vi "Main.vi"() -> ()   [LabVIEW 2021]
doc: "使用该模板构建简单状态机设计模式。各状态执行代码并决定转移状态。"
uses:
  <vilib>/Utility/miscctls.llb/LVRowAndColumnTypeDef.ctl
  controls/State.ctl
  controls/ProcessState.ctl
  <vilib>/Platform/TimedLoop/XDataNode/timing_clust.ctl
  <vilib>/Platform/TimedLoop/XDataNode/nitl_modes.ctl
  <vilib>/Platform/TimedLoop/XDataNode/wakeup.ctl
  controls/DataInitDef.ctl
  <vilib>/event_ctls.llb/eventvkey.ctl
  <vilib>/Utility/NIReport.llb/Report Type.ctl
  controls/Config Section init.ctl
  <vilib>/Platform/TimedLoop/XDataNode/XDataNode.xnode
  <vilib>/Utility/NIReport.llb/NI_report.lvclass
  <vilib>/Utility/NIReport.llb/NI_ReportGenerationCore.lvlib
  <vilib>/Utility/NIReport.llb/Excel/NI_Excel.lvclass
  <vilib>/Platform/TimedLoop/XDataNode/XDNodeRunTimeDep.lvlib
panel:
  in  "项目名":string caption="PCAN 1.6(2021)"
  in  "i2":u32
  in  "i1":i32
  out "运行ID":u32
  in  "曲线16设置":string
  in  "曲线15设置":string
  in  "曲线14设置":string
  in  "曲线13设置":string
  in  "曲线12设置":string
  in  "曲线11设置":string
  in  "曲线10设置":string
  in  "曲线9设置":string
  out "布控5设置":string
  out "CAN通道":u8
  in  "曲线8设置":string
  in  "曲线7设置":string
  in  "曲线6设置":string
  in  "曲线5设置":string
  in  "曲线4设置":string
  in  "曲线3设置":string
  in  "曲线2设置":string
  in  "曲线1设置":string
  out "故障内容":string[](array[string])
  out "故障信息":string[](array[string])
  out "故障地址":string[](array[string])
  out "故障字典":string[][](table)
  out "设控设置 8":string
  out "设控设置 7":string
  out "设控设置 6":string
  out "设控设置 5":string
  out "设控设置 4":string
  out "设控设置 3":string
  out "设控设置 2":string
  out "设控设置 1":string
  out "延时更新布尔状态":i16
  out "要发送的数据":cluster{"地址":u16, "数据":i32, "行数":i32, "ID":i32}
  out "CANBURF":u32[][](array[numeric])
  out "当前显示表格总行数":i32
  out "布控4设置":string
  out "布控2设置":string
  out "布控3设置":string
  out "控件配置文件":string[][](table)
  out "显控12设置":string
  out "显控11设置":string
  out "显控10设置":string
  out "显控9设置":string
  out "显控8设置":string
  out "显控7设置":string
  out "显控6设置":string
  out "显控5设置":string
  out "显控4设置":string
  out "显控3设置":string
  out "显控2设置":string
  out "显控1设置":string
  out "错误计数器":u32
  out "循环指针":u16
  out "布控1设置":string
  out "配置文件":string[][](array[string])
  out "选择区域起始":T1
  in  "选项卡控件":enum32{"调试界面", "波形记录"}(tab)
  in  "确定按钮":bool
  in  "数据模式":bool
  in  "布尔 5":bool
  in  "布尔 4":bool
  in  "布尔 3":bool
  in  "布尔 2":bool
  in  "布尔 1":bool
  in  "ID":u32=43690 format="%x"
  out "通信状态":string
  in  "刷新间隔":string="5" caption="ms"
  out "轮询一次周期":string caption="s"
  in  "重新连接":bool
  in  "波特率":u16(ring)=28 items=["BAUD_5K"=32639, "BAUD_10K"=26415, "BAUD_20K"=21295, "BAUD_50K"=18223, "BAUD_100K"=17199, "BAUD_125K"=796, "BAUD_250K"=284, "BAUD_500K"=28, "BAUD_1M"=20]
  in  "退出":bool=TRUE
  in  "设控8":string
  in  "设控7":string
  in  "设控6":string
  in  "设控5":string
  in  "设控4":string
  in  "设控3":string
  in  "设控2":string
  in  "设控1":string
  out "状态显示":string
  out "显控12":string
  out "显控11":string
  out "显控10":string
  out "显控9":string
  out "显控5":string
  out "显控1":string
  out "显控8":string
  out "显控7":string
  out "显控6":string
  out "显控4":string
  out "显控3":string
  out "显控2":string
  in  "设置":string caption="WARN_H字"
  in  "选择参数表":path caption="导入参数"
  in  "表格":string[][](table)
  in  "清除历史记录":bool
  out "波形图表":dynamicdata(graph)
  in  "记录波形更新":bool=TRUE
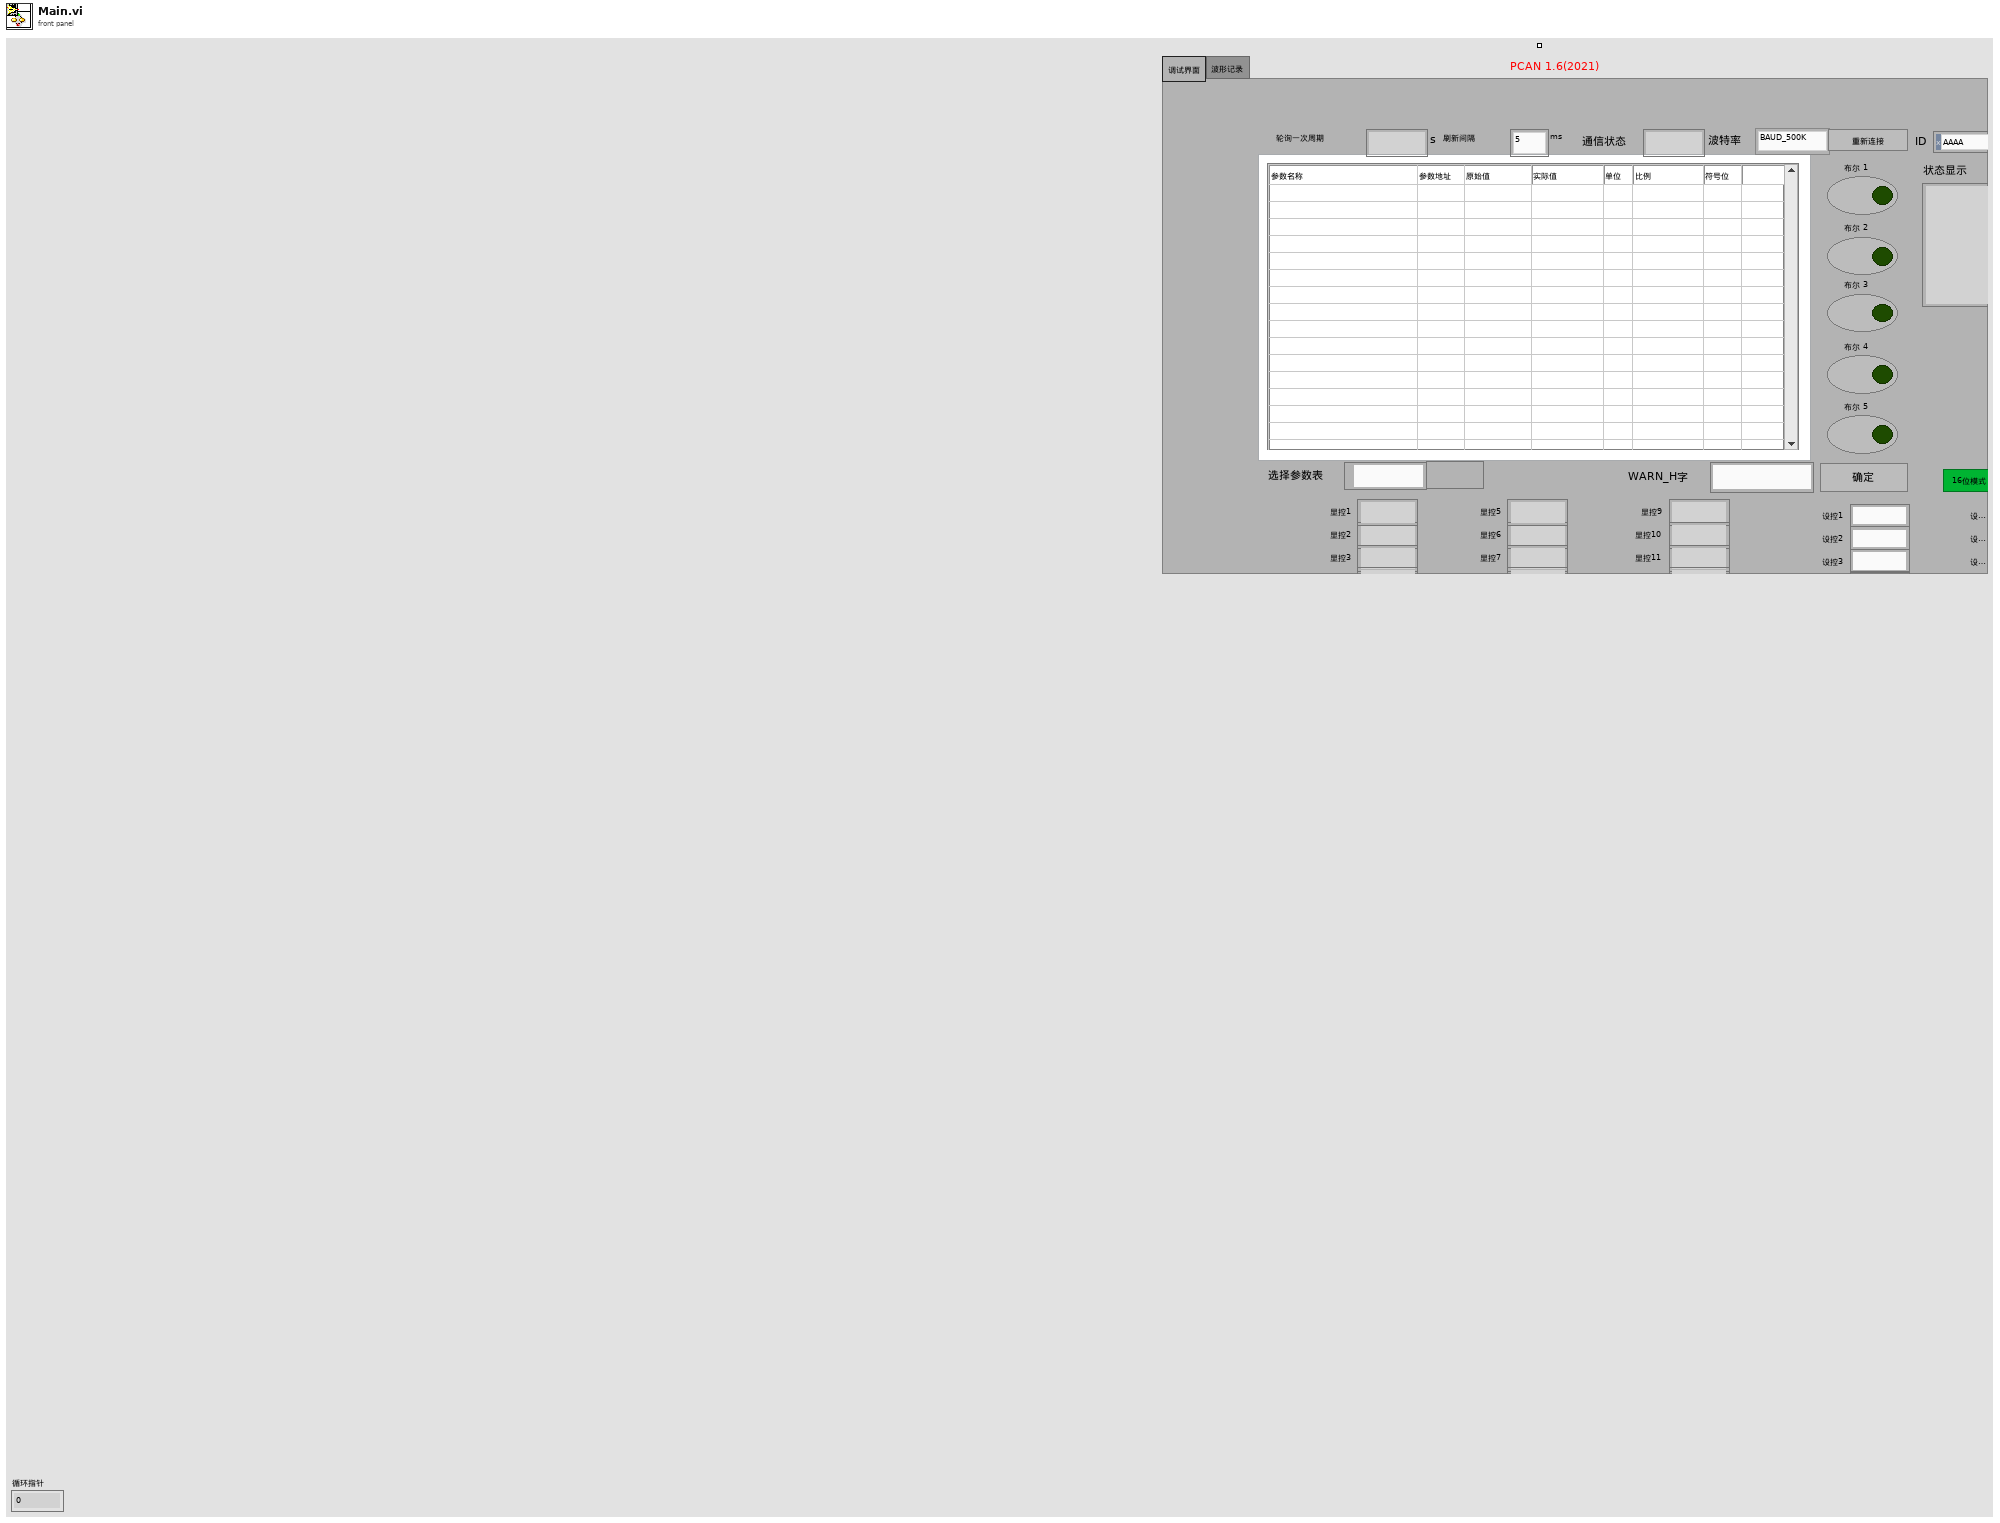
[diagram p1: front panel]
types:
  T1 = typedef "LVRowAndColumnTypeDef.ctl" = cluster{"Row":i32, "Column":i32}
  T2 = typedef "ProcessState.ctl" = enum16{"Start", "Process", "Exit"}
  T3 = typedef "State.ctl" = enum16{"Initialize", "ResetCAN", "SetCAN", "Process", "Exit", "ERROR", "STOP"}
  T4 = typedef "XDNodeRunTimeDep.lvlib/timing_clust.ctl" = cluster{"Expected End [f-1]":u64, "Actual End [f-1]":u64, "Finished Late? [f-1]":bool, "Expected End [i-1]":u64, "Actual End [i-1]":u64, "Finished Late? [i-1]":bool, "Expected Start [i]":u64, "Actual Start [i]":u64, "Expected Start [f]":u64, "Actual Start [f]":u64, "Source Name":string, "Structure Name":string, "Period":i64, "Deadline":i64, "Offset":i64, "Start":i64, "Priority":i32, "Timeout":i32, "Mode":T5, "Wakeup Reason":T6, "Error":errorcluster, "Source Type":string, "Secondary Source Type":string, "Global End Time":u64, "Global Start Time":u64, "Frame Duration":u64, "Iteration Duration":u64, "Assigned CPU":i32, "I/O Scan Engine Mode":u32}
  T5 = typedef "XDNodeRunTimeDep.lvlib/nitl_modes.ctl" = enum32{"No Change", "Process missed periods, maintain original phase", "Discard missed periods, maintain original phase", "Process missed periods, ignore original phase", "Discard missed periods, ignore original phase"}
  T6 = typedef "XDNodeRunTimeDep.lvlib/wakeup.ctl" = enum32{"Normal", "Aborted", "Asynchronous wakeup", "Timing source error", "Timed loop error", "Timeout"}
  T7 = typedef "eventvkey.ctl" = enum16{"ASCII", "Enter", "Return", "Shift", "Ctrl", "Alt", "Cmd", "Opt", "Caps", "NumLock", "Clear", "Break", "Up", "Down", "Left", "Right", "Insert", "Delete", "Home", "End", "PageUp", "PageDown", "Escape", "Help", "Pause", "ScrollLock", "F1", "F2", "F3", "F4", "F5", "F6", "F7", "F8", "F9", "F10", "F11", "F12", "F13", "F14", "F15", "F16", "F17", "F18", "F19", "F20", "F21", "F22", "F23", "F24", "Play", "VolumeUp", "VolumeDown", "Mute", "Two Byte Char"}
  T8 = typedef "NI_ReportGenerationCore.lvlib/Report Type.ctl" = enum16{"HTML", "Word", "Excel"}
  T9 = typedef "DataInitDef.ctl" = u16
  T10 = cluster{u16, i64, "Row":i32, "offset past number":i32}
  T11 = cluster{"position (excel)":cluster{"row":i32, "column":i32}, "name (excel)":string, "bookmark (word)":string}
  T12 = typedef "Config Section init.ctl" = u16
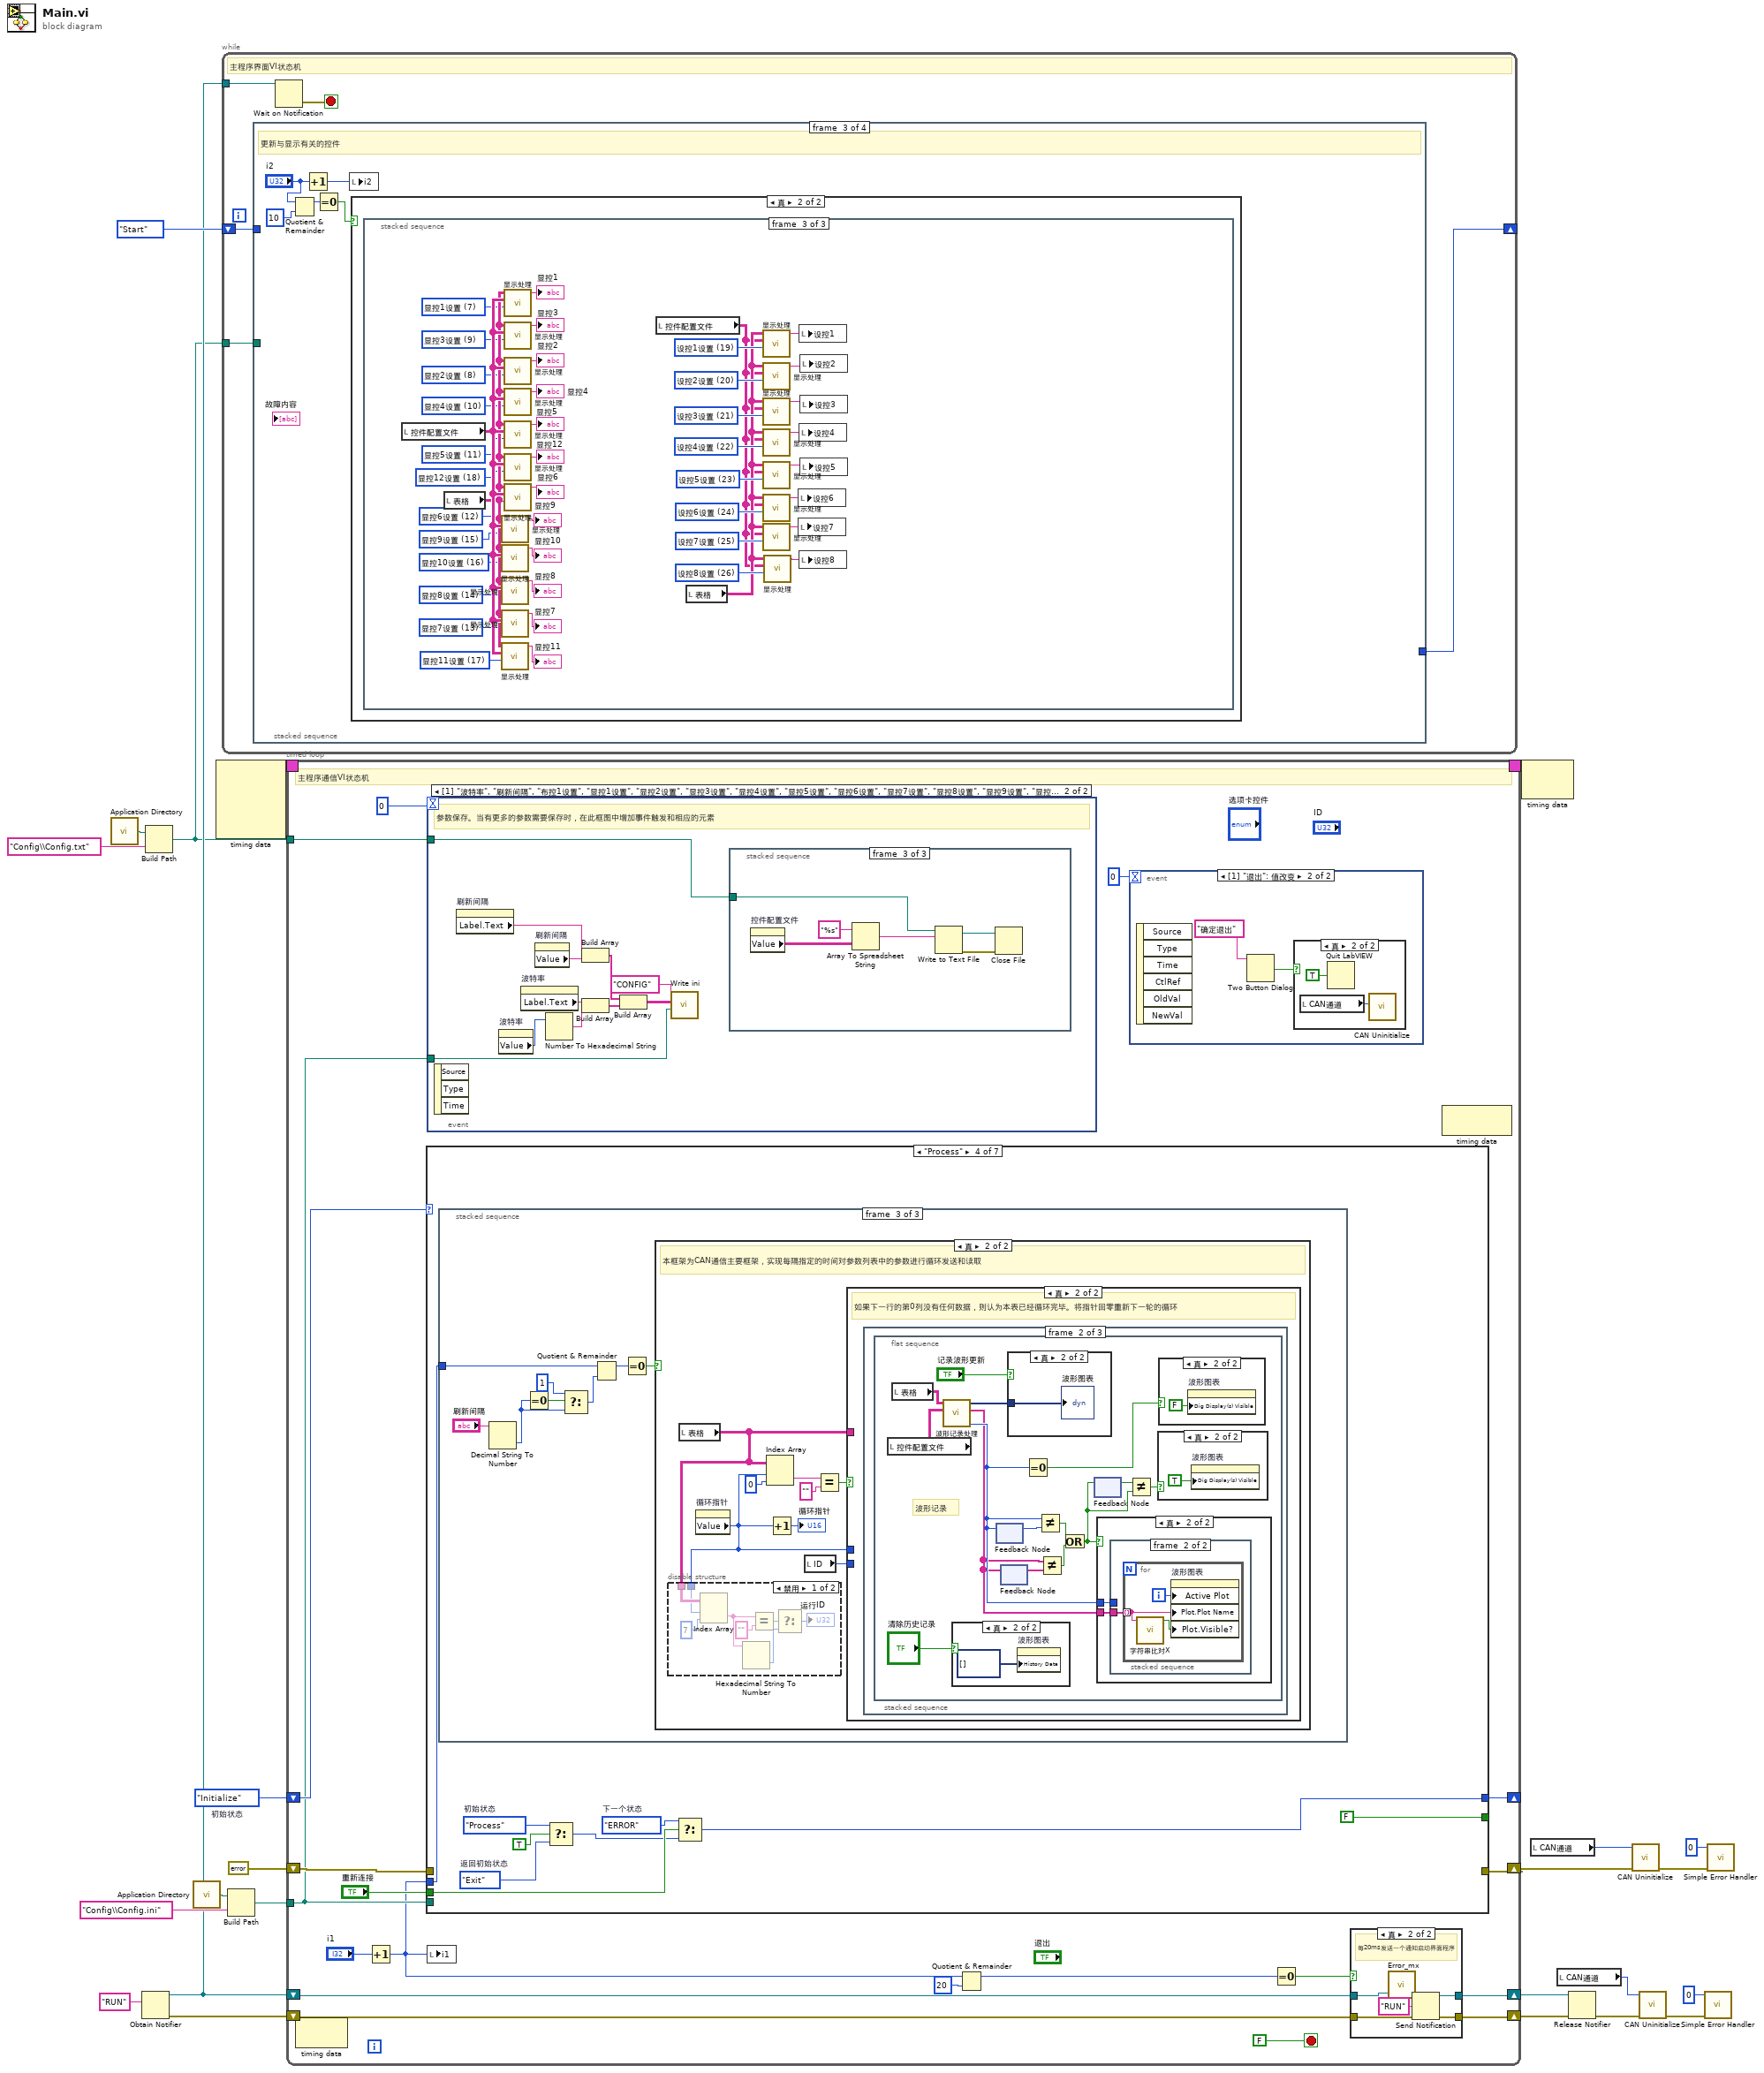
[diagram p0: block diagram]
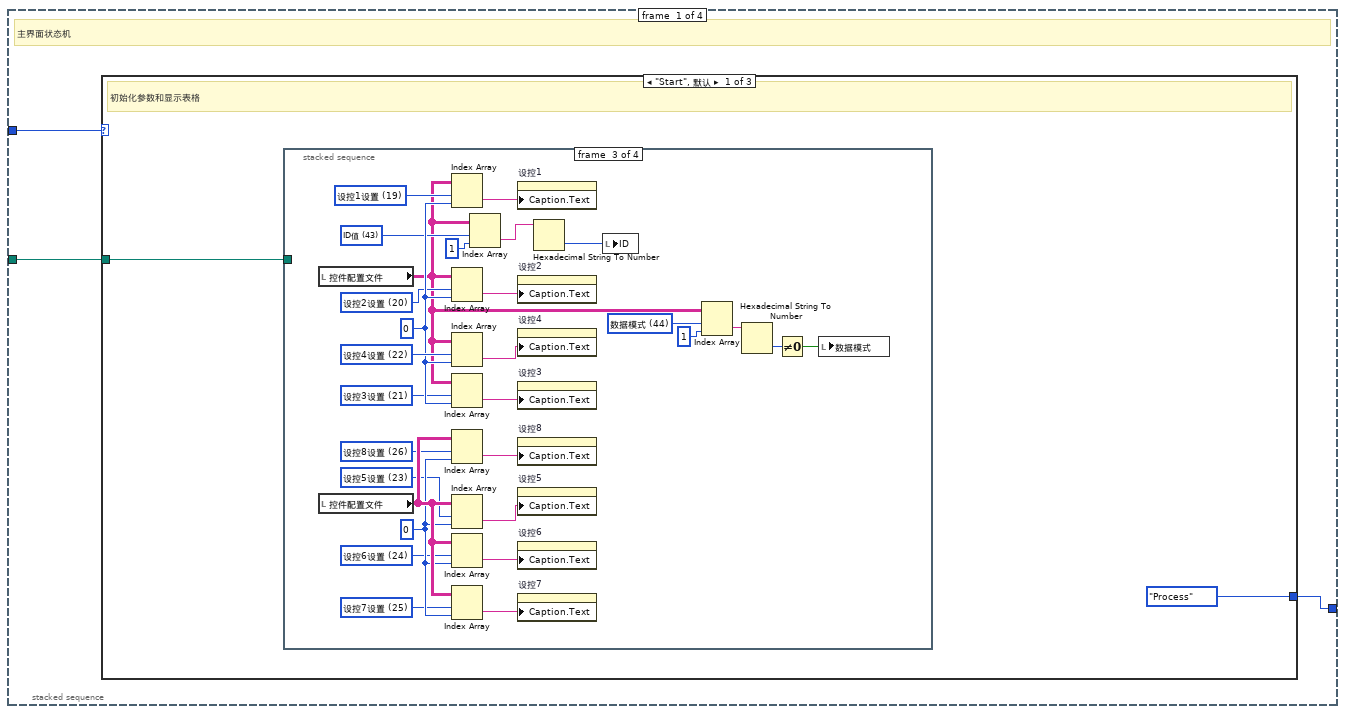
[diagram p2: hidden frame]
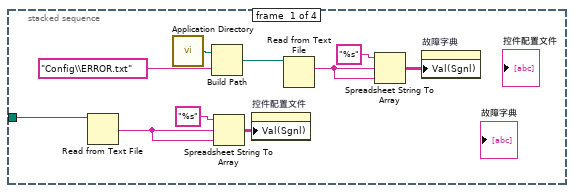
[diagram p3: hidden frame]
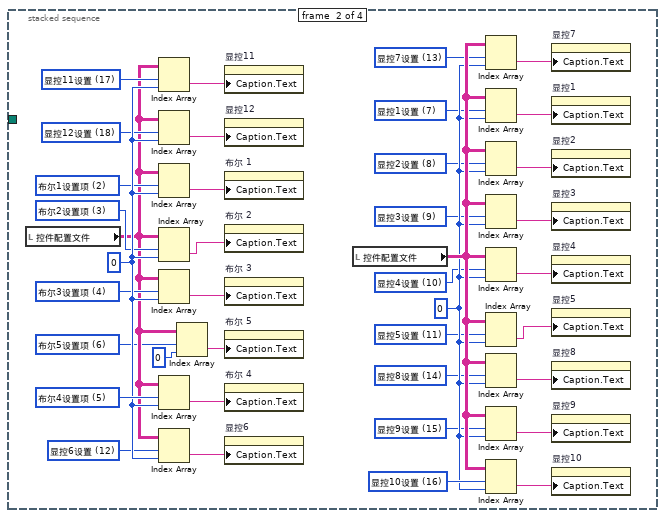
[diagram p4: hidden frame]
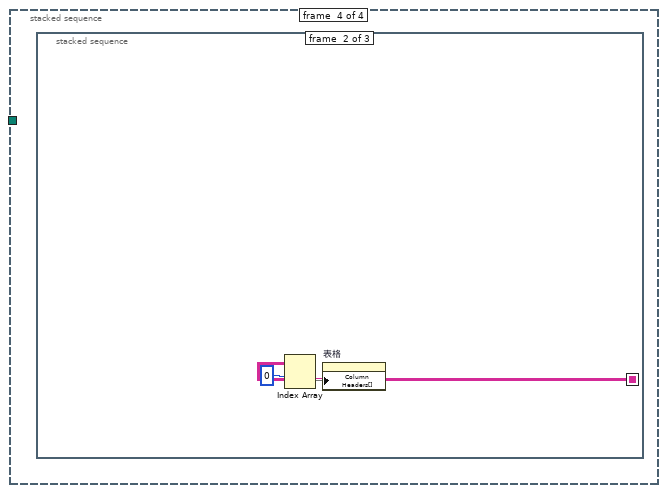
[diagram p5: hidden frame]
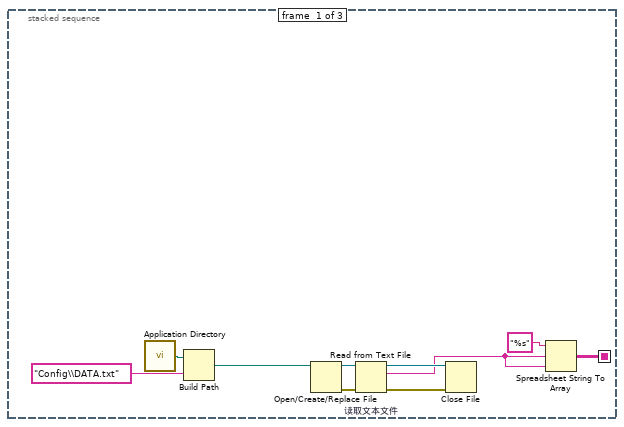
[diagram p6: hidden frame]
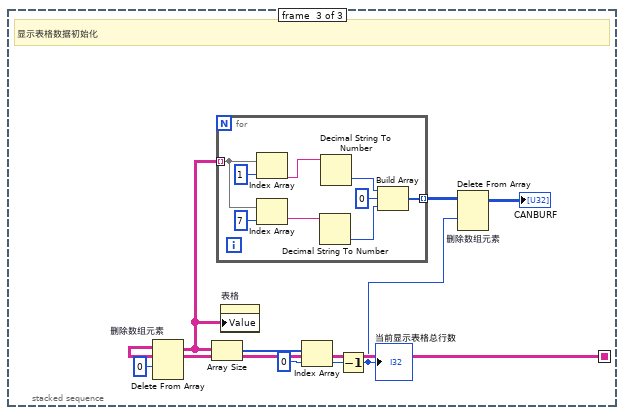
[diagram p7: hidden frame]
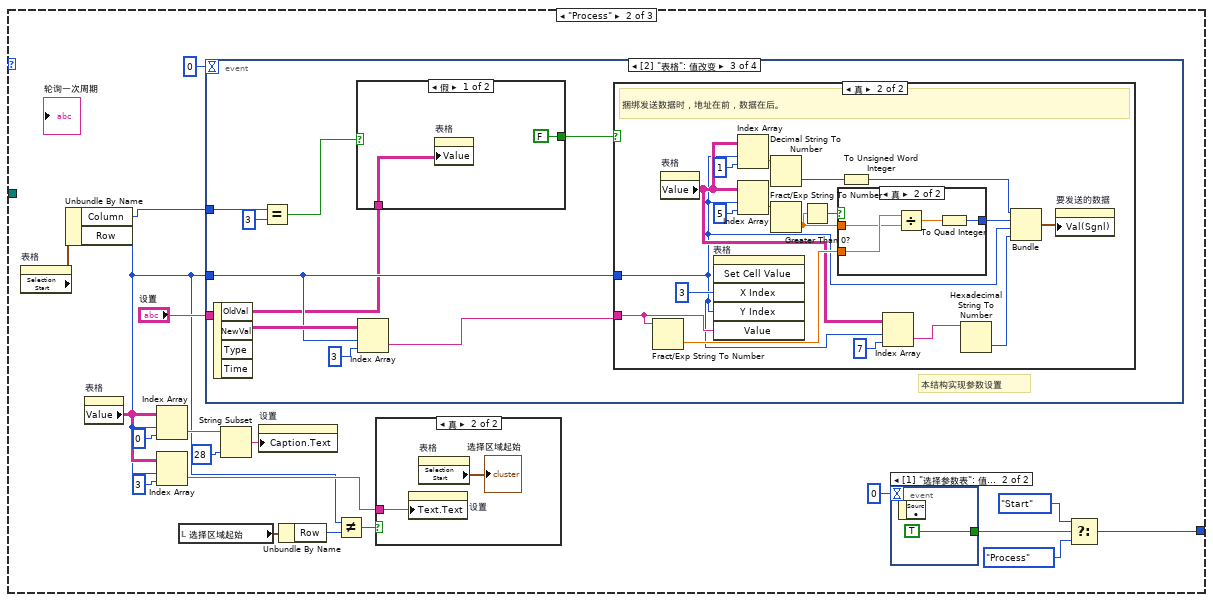
[diagram p8: hidden frame]
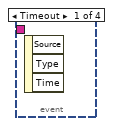
[diagram p10: hidden frame]
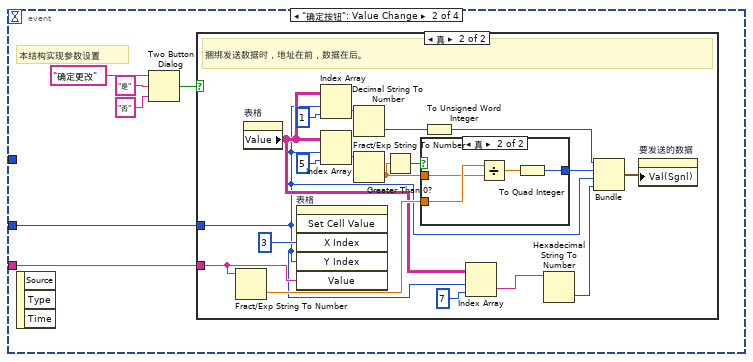
[diagram p11: hidden frame]
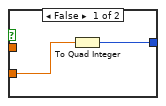
[diagram p13: hidden frame]
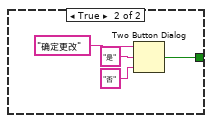
[diagram p14: hidden frame]
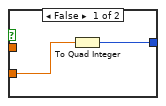
[diagram p16: hidden frame]
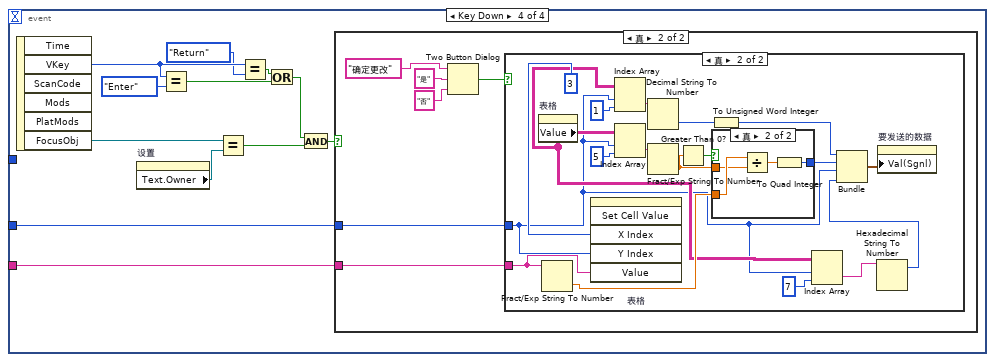
[diagram p17: hidden frame]
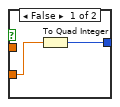
[diagram p20: hidden frame]
diagram:
  w24 = State."Initialize"  # 初始状态
  n1 = call <vilib>:"Application Directory.vi"() -> ("Application Directory"=w9:path)
  n2 = Obtain Notifier(notification data type="RUN" ("通知")) -> (notifier out=w10:refnum<notifier>, error out=w14:errorcluster)  [unwired: 3 in, 1 out]
  n3 = Build Path(base path=w9, name or relative path="Config\\Config.txt" ("名称或相对路径")) -> (appended path=w7:path)
  n4 = call <vilib>:"Application Directory.vi"() -> ("Application Directory"=w16:path)
  n5 = node-c288() -> (w20:T4)  [unwired: 4 in]
  n6 = while {
    shift-right: [w28] -> _
    shift-left: ProcessState."Start" ("ProcessState") -> [w29]
    tunnel: w10 -> [w26]
    tunnel: w7 -> [w25]
    stop <- w27 stop-if-true
    # "主程序界面VI状态机"
    n7 = stacked-sequence {
      tunnel: w29 -> [w32 _ _ _]
      tunnel: [w31 _ _ _] -> w28
      tunnel: w25 -> [w30 _ _ _]
      frame #0 {
        # "主界面状态机"
        n8 = case shown="\"Start\", 默认" w32 {
          tunnel: [ProcessState."Process" ("ProcessState") w161 ProcessState."Exit" ("ProcessState")] -> w31
          tunnel: w30 -> [w33 _ _]
          frame "Start", Default {
            # "初始化参数和显示表格"
            n9 = stacked-sequence {
              tunnel: w33 -> [w42 _ _ _]
              frame #0 {
                n10 = Read from Text File(file (use dialog)=w42) -> (text=w44:string)  [unwired: 3 in, 3 out]
                n11 = call <vilib>:"Application Directory.vi"() -> ("Application Directory"=w39:path)
                n12 = Build Path(base path=w39, name or relative path="Config\\ERROR.txt" ("名称或相对路径")) -> (appended path=w37:path)
                n13 = Spreadsheet String To Array(format string="%s" ("格式字符串"), spreadsheet string=w44, array type (2D Dbl)=w44) -> (array=w36:string[][])  [unwired: 1 in]
                n14 = property on="控件配置文件" class="Tbl (严格)"("Val(Sgnl)"=w36) -> ()  [unwired: 2 in, 2 out]
                n15 = Read from Text File(file (use dialog)=w37) -> (text=w41:string)  [unwired: 3 in, 3 out]
                n16 = Spreadsheet String To Array(format string="%s" ("格式字符串"), spreadsheet string=w41, array type (2D Dbl)=w41) -> (array=w35:string[][])  [unwired: 1 in]
                n17 = property on="故障字典" class="Tbl (严格)"("Val(Sgnl)"=w35) -> ()  [unwired: 2 in, 2 out]
              }
              frame #1 {
                w45 = T9 6 items=["刷新间隔", "波特率", "布尔1设置项", "布尔2设置项", "布尔3设置项", "布尔4设置项", "布尔5设置项", "显控1设置", "显控2设置", "显控3设置", "显控4设置", "显控5设置", "显控6设置", "显控7设置", "显控8设置", "显控9设置", "显控10设置", "显控11设置", "显控12设置", "设控1设置", "设控2设置", "设控3设置", "设控4设置", "设控5设置", "设控6设置", "设控7设置", "设控8设置", "曲线1设置", "曲线2设置", "曲线3设置", "曲线4设置", "曲线5设置", "曲线6设置", "曲线7设置", "曲线8设置", "曲线9设置", "曲线10设置", "曲线11设置", "曲线12设置", "曲线13设置", "曲线14设置", "曲线15设置", "曲线16设置", "ID值"] ("DataInitDef")
                w65 = 0 ("禁用的索引 (列)")
                w66 = T9 5 items=["刷新间隔", "波特率", "布尔1设置项", "布尔2设置项", "布尔3设置项", "布尔4设置项", "布尔5设置项", "显控1设置", "显控2设置", "显控3设置", "显控4设置", "显控5设置", "显控6设置", "显控7设置", "显控8设置", "显控9设置", "显控10设置", "显控11设置", "显控12设置", "设控1设置", "设控2设置", "设控3设置", "设控4设置", "设控5设置", "设控6设置", "设控7设置", "设控8设置", "曲线1设置", "曲线2设置", "曲线3设置", "曲线4设置", "曲线5设置", "曲线6设置", "曲线7设置", "曲线8设置", "曲线9设置", "曲线10设置", "曲线11设置", "曲线12设置", "曲线13设置", "曲线14设置", "曲线15设置", "曲线16设置", "ID值"] ("DataInitDef")
                w64 = T9 4 items=["刷新间隔", "波特率", "布尔1设置项", "布尔2设置项", "布尔3设置项", "布尔4设置项", "布尔5设置项", "显控1设置", "显控2设置", "显控3设置", "显控4设置", "显控5设置", "显控6设置", "显控7设置", "显控8设置", "显控9设置", "显控10设置", "显控11设置", "显控12设置", "设控1设置", "设控2设置", "设控3设置", "设控4设置", "设控5设置", "设控6设置", "设控7设置", "设控8设置", "曲线1设置", "曲线2设置", "曲线3设置", "曲线4设置", "曲线5设置", "曲线6设置", "曲线7设置", "曲线8设置", "曲线9设置", "曲线10设置", "曲线11设置", "曲线12设置", "曲线13设置", "曲线14设置", "曲线15设置", "曲线16设置", "ID值"] ("DataInitDef")
                w63 = T9 3 items=["刷新间隔", "波特率", "布尔1设置项", "布尔2设置项", "布尔3设置项", "布尔4设置项", "布尔5设置项", "显控1设置", "显控2设置", "显控3设置", "显控4设置", "显控5设置", "显控6设置", "显控7设置", "显控8设置", "显控9设置", "显控10设置", "显控11设置", "显控12设置", "设控1设置", "设控2设置", "设控3设置", "设控4设置", "设控5设置", "设控6设置", "设控7设置", "设控8设置", "曲线1设置", "曲线2设置", "曲线3设置", "曲线4设置", "曲线5设置", "曲线6设置", "曲线7设置", "曲线8设置", "曲线9设置", "曲线10设置", "曲线11设置", "曲线12设置", "曲线13设置", "曲线14设置", "曲线15设置", "曲线16设置", "ID值"] ("DataInitDef")
                w62 = T9 2 items=["刷新间隔", "波特率", "布尔1设置项", "布尔2设置项", "布尔3设置项", "布尔4设置项", "布尔5设置项", "显控1设置", "显控2设置", "显控3设置", "显控4设置", "显控5设置", "显控6设置", "显控7设置", "显控8设置", "显控9设置", "显控10设置", "显控11设置", "显控12设置", "设控1设置", "设控2设置", "设控3设置", "设控4设置", "设控5设置", "设控6设置", "设控7设置", "设控8设置", "曲线1设置", "曲线2设置", "曲线3设置", "曲线4设置", "曲线5设置", "曲线6设置", "曲线7设置", "曲线8设置", "曲线9设置", "曲线10设置", "曲线11设置", "曲线12设置", "曲线13设置", "曲线14设置", "曲线15设置", "曲线16设置", "ID值"] ("DataInitDef")
                w61 = T9 18 items=["刷新间隔", "波特率", "布尔1设置项", "布尔2设置项", "布尔3设置项", "布尔4设置项", "布尔5设置项", "显控1设置", "显控2设置", "显控3设置", "显控4设置", "显控5设置", "显控6设置", "显控7设置", "显控8设置", "显控9设置", "显控10设置", "显控11设置", "显控12设置", "设控1设置", "设控2设置", "设控3设置", "设控4设置", "设控5设置", "设控6设置", "设控7设置", "设控8设置", "曲线1设置", "曲线2设置", "曲线3设置", "曲线4设置", "曲线5设置", "曲线6设置", "曲线7设置", "曲线8设置", "曲线9设置", "曲线10设置", "曲线11设置", "曲线12设置", "曲线13设置", "曲线14设置", "曲线15设置", "曲线16设置", "ID值"] ("DataInitDef")
                w60 = T9 17 items=["刷新间隔", "波特率", "布尔1设置项", "布尔2设置项", "布尔3设置项", "布尔4设置项", "布尔5设置项", "显控1设置", "显控2设置", "显控3设置", "显控4设置", "显控5设置", "显控6设置", "显控7设置", "显控8设置", "显控9设置", "显控10设置", "显控11设置", "显控12设置", "设控1设置", "设控2设置", "设控3设置", "设控4设置", "设控5设置", "设控6设置", "设控7设置", "设控8设置", "曲线1设置", "曲线2设置", "曲线3设置", "曲线4设置", "曲线5设置", "曲线6设置", "曲线7设置", "曲线8设置", "曲线9设置", "曲线10设置", "曲线11设置", "曲线12设置", "曲线13设置", "曲线14设置", "曲线15设置", "曲线16设置", "ID值"] ("DataInitDef")
                w59 = T9 16 items=["刷新间隔", "波特率", "布尔1设置项", "布尔2设置项", "布尔3设置项", "布尔4设置项", "布尔5设置项", "显控1设置", "显控2设置", "显控3设置", "显控4设置", "显控5设置", "显控6设置", "显控7设置", "显控8设置", "显控9设置", "显控10设置", "显控11设置", "显控12设置", "设控1设置", "设控2设置", "设控3设置", "设控4设置", "设控5设置", "设控6设置", "设控7设置", "设控8设置", "曲线1设置", "曲线2设置", "曲线3设置", "曲线4设置", "曲线5设置", "曲线6设置", "曲线7设置", "曲线8设置", "曲线9设置", "曲线10设置", "曲线11设置", "曲线12设置", "曲线13设置", "曲线14设置", "曲线15设置", "曲线16设置", "ID值"] ("DataInitDef")
                w57 = T9 15 items=["刷新间隔", "波特率", "布尔1设置项", "布尔2设置项", "布尔3设置项", "布尔4设置项", "布尔5设置项", "显控1设置", "显控2设置", "显控3设置", "显控4设置", "显控5设置", "显控6设置", "显控7设置", "显控8设置", "显控9设置", "显控10设置", "显控11设置", "显控12设置", "设控1设置", "设控2设置", "设控3设置", "设控4设置", "设控5设置", "设控6设置", "设控7设置", "设控8设置", "曲线1设置", "曲线2设置", "曲线3设置", "曲线4设置", "曲线5设置", "曲线6设置", "曲线7设置", "曲线8设置", "曲线9设置", "曲线10设置", "曲线11设置", "曲线12设置", "曲线13设置", "曲线14设置", "曲线15设置", "曲线16设置", "ID值"] ("DataInitDef")
                w56 = T9 14 items=["刷新间隔", "波特率", "布尔1设置项", "布尔2设置项", "布尔3设置项", "布尔4设置项", "布尔5设置项", "显控1设置", "显控2设置", "显控3设置", "显控4设置", "显控5设置", "显控6设置", "显控7设置", "显控8设置", "显控9设置", "显控10设置", "显控11设置", "显控12设置", "设控1设置", "设控2设置", "设控3设置", "设控4设置", "设控5设置", "设控6设置", "设控7设置", "设控8设置", "曲线1设置", "曲线2设置", "曲线3设置", "曲线4设置", "曲线5设置", "曲线6设置", "曲线7设置", "曲线8设置", "曲线9设置", "曲线10设置", "曲线11设置", "曲线12设置", "曲线13设置", "曲线14设置", "曲线15设置", "曲线16设置", "ID值"] ("DataInitDef")
                w55 = T9 11 items=["刷新间隔", "波特率", "布尔1设置项", "布尔2设置项", "布尔3设置项", "布尔4设置项", "布尔5设置项", "显控1设置", "显控2设置", "显控3设置", "显控4设置", "显控5设置", "显控6设置", "显控7设置", "显控8设置", "显控9设置", "显控10设置", "显控11设置", "显控12设置", "设控1设置", "设控2设置", "设控3设置", "设控4设置", "设控5设置", "设控6设置", "设控7设置", "设控8设置", "曲线1设置", "曲线2设置", "曲线3设置", "曲线4设置", "曲线5设置", "曲线6设置", "曲线7设置", "曲线8设置", "曲线9设置", "曲线10设置", "曲线11设置", "曲线12设置", "曲线13设置", "曲线14设置", "曲线15设置", "曲线16设置", "ID值"] ("DataInitDef")
                w54 = T9 10 items=["刷新间隔", "波特率", "布尔1设置项", "布尔2设置项", "布尔3设置项", "布尔4设置项", "布尔5设置项", "显控1设置", "显控2设置", "显控3设置", "显控4设置", "显控5设置", "显控6设置", "显控7设置", "显控8设置", "显控9设置", "显控10设置", "显控11设置", "显控12设置", "设控1设置", "设控2设置", "设控3设置", "设控4设置", "设控5设置", "设控6设置", "设控7设置", "设控8设置", "曲线1设置", "曲线2设置", "曲线3设置", "曲线4设置", "曲线5设置", "曲线6设置", "曲线7设置", "曲线8设置", "曲线9设置", "曲线10设置", "曲线11设置", "曲线12设置", "曲线13设置", "曲线14设置", "曲线15设置", "曲线16设置", "ID值"] ("DataInitDef")
                w53 = T9 9 items=["刷新间隔", "波特率", "布尔1设置项", "布尔2设置项", "布尔3设置项", "布尔4设置项", "布尔5设置项", "显控1设置", "显控2设置", "显控3设置", "显控4设置", "显控5设置", "显控6设置", "显控7设置", "显控8设置", "显控9设置", "显控10设置", "显控11设置", "显控12设置", "设控1设置", "设控2设置", "设控3设置", "设控4设置", "设控5设置", "设控6设置", "设控7设置", "设控8设置", "曲线1设置", "曲线2设置", "曲线3设置", "曲线4设置", "曲线5设置", "曲线6设置", "曲线7设置", "曲线8设置", "曲线9设置", "曲线10设置", "曲线11设置", "曲线12设置", "曲线13设置", "曲线14设置", "曲线15设置", "曲线16设置", "ID值"] ("DataInitDef")
                w52 = T9 8 items=["刷新间隔", "波特率", "布尔1设置项", "布尔2设置项", "布尔3设置项", "布尔4设置项", "布尔5设置项", "显控1设置", "显控2设置", "显控3设置", "显控4设置", "显控5设置", "显控6设置", "显控7设置", "显控8设置", "显控9设置", "显控10设置", "显控11设置", "显控12设置", "设控1设置", "设控2设置", "设控3设置", "设控4设置", "设控5设置", "设控6设置", "设控7设置", "设控8设置", "曲线1设置", "曲线2设置", "曲线3设置", "曲线4设置", "曲线5设置", "曲线6设置", "曲线7设置", "曲线8设置", "曲线9设置", "曲线10设置", "曲线11设置", "曲线12设置", "曲线13设置", "曲线14设置", "曲线15设置", "曲线16设置", "ID值"] ("DataInitDef")
                w51 = T9 7 items=["刷新间隔", "波特率", "布尔1设置项", "布尔2设置项", "布尔3设置项", "布尔4设置项", "布尔5设置项", "显控1设置", "显控2设置", "显控3设置", "显控4设置", "显控5设置", "显控6设置", "显控7设置", "显控8设置", "显控9设置", "显控10设置", "显控11设置", "显控12设置", "设控1设置", "设控2设置", "设控3设置", "设控4设置", "设控5设置", "设控6设置", "设控7设置", "设控8设置", "曲线1设置", "曲线2设置", "曲线3设置", "曲线4设置", "曲线5设置", "曲线6设置", "曲线7设置", "曲线8设置", "曲线9设置", "曲线10设置", "曲线11设置", "曲线12设置", "曲线13设置", "曲线14设置", "曲线15设置", "曲线16设置", "ID值"] ("DataInitDef")
                w50 = T9 13 items=["刷新间隔", "波特率", "布尔1设置项", "布尔2设置项", "布尔3设置项", "布尔4设置项", "布尔5设置项", "显控1设置", "显控2设置", "显控3设置", "显控4设置", "显控5设置", "显控6设置", "显控7设置", "显控8设置", "显控9设置", "显控10设置", "显控11设置", "显控12设置", "设控1设置", "设控2设置", "设控3设置", "设控4设置", "设控5设置", "设控6设置", "设控7设置", "设控8设置", "曲线1设置", "曲线2设置", "曲线3设置", "曲线4设置", "曲线5设置", "曲线6设置", "曲线7设置", "曲线8设置", "曲线9设置", "曲线10设置", "曲线11设置", "曲线12设置", "曲线13设置", "曲线14设置", "曲线15设置", "曲线16设置", "ID值"] ("DataInitDef")
                w49 = T9 12 items=["刷新间隔", "波特率", "布尔1设置项", "布尔2设置项", "布尔3设置项", "布尔4设置项", "布尔5设置项", "显控1设置", "显控2设置", "显控3设置", "显控4设置", "显控5设置", "显控6设置", "显控7设置", "显控8设置", "显控9设置", "显控10设置", "显控11设置", "显控12设置", "设控1设置", "设控2设置", "设控3设置", "设控4设置", "设控5设置", "设控6设置", "设控7设置", "设控8设置", "曲线1设置", "曲线2设置", "曲线3设置", "曲线4设置", "曲线5设置", "曲线6设置", "曲线7设置", "曲线8设置", "曲线9设置", "曲线10设置", "曲线11设置", "曲线12设置", "曲线13设置", "曲线14设置", "曲线15设置", "曲线16设置", "ID值"] ("DataInitDef")
                w58 = 0 ("禁用的索引 (列)")
                n18 = local read "控件配置文件"() -> (w47:string[][])
                n19 = Index Array(array=w47, index (row)=w60, index (col)=w65) -> (element=w77:string)
                n20 = Index Array(array=w47, index (row)=w61, index (col)=w65) -> (element=w78:string)
                n21 = Index Array(array=w47, index (row)=w62, index (col)=w65) -> (element=w80:string)
                n22 = Index Array(array=w47, index (row)=w63, index (col)=w65) -> (element=w81:string)
                n23 = Index Array(array=w47, index (row)=w64, index (col)=w65) -> (element=w82:string)
                n24 = Index Array(array=w47, index (row)=w66, index (col)=w65) -> (element=w83:string)
                n25 = Index Array(array=w47, index (row)=w49, index (col)=w65) -> (element=w67:string)
                n26 = Index Array(array=w47, index (row)=w45, index (col)=0 ("禁用的索引 (列)")) -> (element=w48:string)
                n27 = property on="显控11" class="Str"("Caption.Text"=w77) -> ()  [unwired: 2 in, 2 out]
                n28 = property on="显控12" class="Str"("Caption.Text"=w78) -> ()  [unwired: 2 in, 2 out]
                n29 = property on="布尔 1" class="Bool (严格)"("Caption.Text"=w80) -> ()  [unwired: 2 in, 2 out]
                n30 = property on="布尔 2" class="Bool (严格)"("Caption.Text"=w81) -> ()  [unwired: 2 in, 2 out]
                n31 = property on="布尔 3" class="Bool (严格)"("Caption.Text"=w82) -> ()  [unwired: 2 in, 2 out]
                n32 = property on="布尔 5" class="Bool (严格)"("Caption.Text"=w48) -> ()  [unwired: 2 in, 2 out]
                n33 = property on="布尔 4" class="Bool (严格)"("Caption.Text"=w83) -> ()  [unwired: 2 in, 2 out]
                n34 = property on="显控6" class="Str"("Caption.Text"=w67) -> ()  [unwired: 2 in, 2 out]
                n35 = local read "控件配置文件"() -> (w79:string[][])
                n36 = Index Array(array=w79, index (row)=w50, index (col)=w58) -> (element=w68:string)
                n37 = Index Array(array=w79, index (row)=w51, index (col)=w58) -> (element=w69:string)
                n38 = Index Array(array=w79, index (row)=w52, index (col)=w58) -> (element=w70:string)
                n39 = Index Array(array=w79, index (row)=w53, index (col)=w58) -> (element=w71:string)
                n40 = Index Array(array=w79, index (row)=w54, index (col)=w58) -> (element=w72:string)
                n41 = Index Array(array=w79, index (row)=w55, index (col)=w58) -> (element=w73:string)
                n42 = Index Array(array=w79, index (row)=w56, index (col)=w58) -> (element=w74:string)
                n43 = Index Array(array=w79, index (row)=w57, index (col)=w58) -> (element=w75:string)
                n44 = Index Array(array=w79, index (row)=w59, index (col)=w58) -> (element=w76:string)
                n45 = property on="显控7" class="Str"("Caption.Text"=w68) -> ()  [unwired: 2 in, 2 out]
                n46 = property on="显控1" class="Str"("Caption.Text"=w69) -> ()  [unwired: 2 in, 2 out]
                n47 = property on="显控2" class="Str"("Caption.Text"=w70) -> ()  [unwired: 2 in, 2 out]
                n48 = property on="显控3" class="Str"("Caption.Text"=w71) -> ()  [unwired: 2 in, 2 out]
                n49 = property on="显控4" class="Str"("Caption.Text"=w72) -> ()  [unwired: 2 in, 2 out]
                n50 = property on="显控5" class="Str"("Caption.Text"=w73) -> ()  [unwired: 2 in, 2 out]
                n51 = property on="显控8" class="Str"("Caption.Text"=w74) -> ()  [unwired: 2 in, 2 out]
                n52 = property on="显控9" class="Str"("Caption.Text"=w75) -> ()  [unwired: 2 in, 2 out]
                n53 = property on="显控10" class="Str"("Caption.Text"=w76) -> ()  [unwired: 2 in, 2 out]
              }
              frame #2 {
                w84 = T9 44 items=["刷新间隔", "波特率", "布尔1设置项", "布尔2设置项", "布尔3设置项", "布尔4设置项", "布尔5设置项", "显控1设置", "显控2设置", "显控3设置", "显控4设置", "显控5设置", "显控6设置", "显控7设置", "显控8设置", "显控9设置", "显控10设置", "显控11设置", "显控12设置", "设控1设置", "设控2设置", "设控3设置", "设控4设置", "设控5设置", "设控6设置", "设控7设置", "设控8设置", "曲线1设置", "曲线2设置", "曲线3设置", "曲线4设置", "曲线5设置", "曲线6设置", "曲线7设置", "曲线8设置", "曲线9设置", "曲线10设置", "曲线11设置", "曲线12设置", "曲线13设置", "曲线14设置", "曲线15设置", "曲线16设置", "ID值", "数据模式"] ("DataInitDef")
                w93 = T9 43 items=["刷新间隔", "波特率", "布尔1设置项", "布尔2设置项", "布尔3设置项", "布尔4设置项", "布尔5设置项", "显控1设置", "显控2设置", "显控3设置", "显控4设置", "显控5设置", "显控6设置", "显控7设置", "显控8设置", "显控9设置", "显控10设置", "显控11设置", "显控12设置", "设控1设置", "设控2设置", "设控3设置", "设控4设置", "设控5设置", "设控6设置", "设控7设置", "设控8设置", "曲线1设置", "曲线2设置", "曲线3设置", "曲线4设置", "曲线5设置", "曲线6设置", "曲线7设置", "曲线8设置", "曲线9设置", "曲线10设置", "曲线11设置", "曲线12设置", "曲线13设置", "曲线14设置", "曲线15设置", "曲线16设置", "ID值"] ("DataInitDef")
                w103 = T9 26 items=["刷新间隔", "波特率", "布尔1设置项", "布尔2设置项", "布尔3设置项", "布尔4设置项", "布尔5设置项", "显控1设置", "显控2设置", "显控3设置", "显控4设置", "显控5设置", "显控6设置", "显控7设置", "显控8设置", "显控9设置", "显控10设置", "显控11设置", "显控12设置", "设控1设置", "设控2设置", "设控3设置", "设控4设置", "设控5设置", "设控6设置", "设控7设置", "设控8设置", "曲线1设置", "曲线2设置", "曲线3设置", "曲线4设置", "曲线5设置", "曲线6设置", "曲线7设置", "曲线8设置", "曲线9设置", "曲线10设置", "曲线11设置", "曲线12设置", "曲线13设置", "曲线14设置", "曲线15设置", "曲线16设置", "ID值"] ("DataInitDef")
                w99 = T9 25 items=["刷新间隔", "波特率", "布尔1设置项", "布尔2设置项", "布尔3设置项", "布尔4设置项", "布尔5设置项", "显控1设置", "显控2设置", "显控3设置", "显控4设置", "显控5设置", "显控6设置", "显控7设置", "显控8设置", "显控9设置", "显控10设置", "显控11设置", "显控12设置", "设控1设置", "设控2设置", "设控3设置", "设控4设置", "设控5设置", "设控6设置", "设控7设置", "设控8设置", "曲线1设置", "曲线2设置", "曲线3设置", "曲线4设置", "曲线5设置", "曲线6设置", "曲线7设置", "曲线8设置", "曲线9设置", "曲线10设置", "曲线11设置", "曲线12设置", "曲线13设置", "曲线14设置", "曲线15设置", "曲线16设置", "ID值"] ("DataInitDef")
                w101 = T9 24 items=["刷新间隔", "波特率", "布尔1设置项", "布尔2设置项", "布尔3设置项", "布尔4设置项", "布尔5设置项", "显控1设置", "显控2设置", "显控3设置", "显控4设置", "显控5设置", "显控6设置", "显控7设置", "显控8设置", "显控9设置", "显控10设置", "显控11设置", "显控12设置", "设控1设置", "设控2设置", "设控3设置", "设控4设置", "设控5设置", "设控6设置", "设控7设置", "设控8设置", "曲线1设置", "曲线2设置", "曲线3设置", "曲线4设置", "曲线5设置", "曲线6设置", "曲线7设置", "曲线8设置", "曲线9设置", "曲线10设置", "曲线11设置", "曲线12设置", "曲线13设置", "曲线14设置", "曲线15设置", "曲线16设置", "ID值"] ("DataInitDef")
                w100 = T9 23 items=["刷新间隔", "波特率", "布尔1设置项", "布尔2设置项", "布尔3设置项", "布尔4设置项", "布尔5设置项", "显控1设置", "显控2设置", "显控3设置", "显控4设置", "显控5设置", "显控6设置", "显控7设置", "显控8设置", "显控9设置", "显控10设置", "显控11设置", "显控12设置", "设控1设置", "设控2设置", "设控3设置", "设控4设置", "设控5设置", "设控6设置", "设控7设置", "设控8设置", "曲线1设置", "曲线2设置", "曲线3设置", "曲线4设置", "曲线5设置", "曲线6设置", "曲线7设置", "曲线8设置", "曲线9设置", "曲线10设置", "曲线11设置", "曲线12设置", "曲线13设置", "曲线14设置", "曲线15设置", "曲线16设置", "ID值"] ("DataInitDef")
                w102 = 0 ("禁用的索引 (列)")
                w98 = T9 22 items=["刷新间隔", "波特率", "布尔1设置项", "布尔2设置项", "布尔3设置项", "布尔4设置项", "布尔5设置项", "显控1设置", "显控2设置", "显控3设置", "显控4设置", "显控5设置", "显控6设置", "显控7设置", "显控8设置", "显控9设置", "显控10设置", "显控11设置", "显控12设置", "设控1设置", "设控2设置", "设控3设置", "设控4设置", "设控5设置", "设控6设置", "设控7设置", "设控8设置", "曲线1设置", "曲线2设置", "曲线3设置", "曲线4设置", "曲线5设置", "曲线6设置", "曲线7设置", "曲线8设置", "曲线9设置", "曲线10设置", "曲线11设置", "曲线12设置", "曲线13设置", "曲线14设置", "曲线15设置", "曲线16设置", "ID值"] ("DataInitDef")
                w94 = T9 21 items=["刷新间隔", "波特率", "布尔1设置项", "布尔2设置项", "布尔3设置项", "布尔4设置项", "布尔5设置项", "显控1设置", "显控2设置", "显控3设置", "显控4设置", "显控5设置", "显控6设置", "显控7设置", "显控8设置", "显控9设置", "显控10设置", "显控11设置", "显控12设置", "设控1设置", "设控2设置", "设控3设置", "设控4设置", "设控5设置", "设控6设置", "设控7设置", "设控8设置", "曲线1设置", "曲线2设置", "曲线3设置", "曲线4设置", "曲线5设置", "曲线6设置", "曲线7设置", "曲线8设置", "曲线9设置", "曲线10设置", "曲线11设置", "曲线12设置", "曲线13设置", "曲线14设置", "曲线15设置", "曲线16设置", "ID值"] ("DataInitDef")
                w96 = T9 20 items=["刷新间隔", "波特率", "布尔1设置项", "布尔2设置项", "布尔3设置项", "布尔4设置项", "布尔5设置项", "显控1设置", "显控2设置", "显控3设置", "显控4设置", "显控5设置", "显控6设置", "显控7设置", "显控8设置", "显控9设置", "显控10设置", "显控11设置", "显控12设置", "设控1设置", "设控2设置", "设控3设置", "设控4设置", "设控5设置", "设控6设置", "设控7设置", "设控8设置", "曲线1设置", "曲线2设置", "曲线3设置", "曲线4设置", "曲线5设置", "曲线6设置", "曲线7设置", "曲线8设置", "曲线9设置", "曲线10设置", "曲线11设置", "曲线12设置", "曲线13设置", "曲线14设置", "曲线15设置", "曲线16设置", "ID值"] ("DataInitDef")
                w95 = T9 19 items=["刷新间隔", "波特率", "布尔1设置项", "布尔2设置项", "布尔3设置项", "布尔4设置项", "布尔5设置项", "显控1设置", "显控2设置", "显控3设置", "显控4设置", "显控5设置", "显控6设置", "显控7设置", "显控8设置", "显控9设置", "显控10设置", "显控11设置", "显控12设置", "设控1设置", "设控2设置", "设控3设置", "设控4设置", "设控5设置", "设控6设置", "设控7设置", "设控8设置", "曲线1设置", "曲线2设置", "曲线3设置", "曲线4设置", "曲线5设置", "曲线6设置", "曲线7设置", "曲线8设置", "曲线9设置", "曲线10设置", "曲线11设置", "曲线12设置", "曲线13设置", "曲线14设置", "曲线15设置", "曲线16设置", "ID值"] ("DataInitDef")
                w97 = 0 ("禁用的索引 (列)")
                n54 = local read "控件配置文件"() -> (w87:string[][])
                n55 = local read "控件配置文件"() -> (w108:string[][])
                n56 = Index Array(array=w87, index (row)=w95, index (col)=w97) -> (element=w111:string)
                n57 = Index Array(array=w87, index (row)=w96, index (col)=w97) -> (element=w110:string)
                n58 = Index Array(array=w87, index (row)=w98, index (col)=w97) -> (element=w109:string)
                n59 = Index Array(array=w87, index (row)=w94, index (col)=w97) -> (element=w112:string)
                n60 = Index Array(array=w108, index (row)=w103, index (col)=w102) -> (element=w107:string)
                n61 = Index Array(array=w108, index (row)=w100, index (col)=w102) -> (element=w105:string)
                n62 = Index Array(array=w108, index (row)=w101, index (col)=w102) -> (element=w106:string)
                n63 = Index Array(array=w108, index (row)=w99, index (col)=w102) -> (element=w104:string)
                n64 = Index Array(array=w87, index (row)=w93, index (col)=1 ("禁用的索引 (列)")) -> (element=w91:string)
                n65 = property on="设控1" class="Str"("Caption.Text"=w111) -> ()  [unwired: 2 in, 2 out]
                n66 = property on="设控2" class="Str"("Caption.Text"=w110) -> ()  [unwired: 2 in, 2 out]
                n67 = property on="设控4" class="Str"("Caption.Text"=w109) -> ()  [unwired: 2 in, 2 out]
                n68 = property on="设控3" class="Str"("Caption.Text"=w112) -> ()  [unwired: 2 in, 2 out]
                n69 = property on="设控8" class="Str"("Caption.Text"=w107) -> ()  [unwired: 2 in, 2 out]
                n70 = property on="设控5" class="Str"("Caption.Text"=w105) -> ()  [unwired: 2 in, 2 out]
                n71 = property on="设控6" class="Str"("Caption.Text"=w106) -> ()  [unwired: 2 in, 2 out]
                n72 = property on="设控7" class="Str"("Caption.Text"=w104) -> ()  [unwired: 2 in, 2 out]
                n73 = Hexadecimal String To Number(string=w91) -> (number=w90:u32)  [unwired: 2 in, 1 out]
                n74 = local write "ID"(w90) -> ()
                n75 = Index Array(array=w87, index (row)=w84, index (col)=1 ("禁用的索引 (列)")) -> (element=w88:string)
                n76 = Hexadecimal String To Number(string=w88) -> (number=w86:u32)  [unwired: 2 in, 1 out]
                n77 = Not Equal To 0?(x=w86) -> (x != 0?=w85:bool)
                n78 = local write "数据模式"(w85) -> ()
              }
              frame #3 {
                n79 = stacked-sequence {
                  seq-local: [w113 _ _] -> [_ w123 w132]
                  frame #0 {
                    n80 = call <vilib>:"Application Directory.vi"() -> ("Application Directory"=w119:path)
                    n81 = Build Path(base path=w119, name or relative path="Config\\DATA.txt" ("名称或相对路径")) -> (appended path=w120:path)
                    n82 = Open/Create/Replace File(file path (use dialog)=w120) -> (refnum out=w118:refnum<file>, error out=w117:errorcluster)  [unwired: 5 in, 1 out]
                    n83 = Read from Text File "读取文本文件"(file (use dialog)=w118, error in=w117) -> (refnum out=w121:refnum<file>, text=w116:string, error out=w122:errorcluster)  [unwired: 2 in, 1 out]
                    n84 = Close File(refnum=w121, error in=w122) -> ()  [unwired: 2 out]
                    n85 = Spreadsheet String To Array(format string="%s" ("格式字符串"), spreadsheet string=w116, array type (2D Dbl)=w116) -> (array=w113:string[][])  [unwired: 1 in]
                  }
                  frame #1 {
                    n86 = Index Array(array=w123, index (row)=0 ("索引 (行)")) -> (element=w125:string[])  [unwired: 1 in]
                    n87 = property on="表格" class="Tbl (严格)"("Column Headers[]"=w125) -> ()  [unwired: 2 in, 2 out]
                  }
                  frame #2 {
                    # "显示表格数据初始化"
                    n88 = Delete From Array "删除数组元素"(array=w132, index (row)=0 ("索引 (行)")) -> (array with subset deleted=w130:string[][])  [unwired: 2 in, 1 out]
                    n89 = Array Size(array=w130) -> (size(s)=w131:i32[])
                    n90 = for "For循环" {
                      tunnel: w130 -> [w141] mode=indexing
                      tunnel: [w135] -> w129 mode=indexing
                      n91 = Index Array(array=w141, index=1 ("索引")) -> (element=w140:string)
                      n92 = Index Array(array=w141, index=7 ("索引")) -> (element=w139:string)
                      n93 = Decimal String To Number(string=w139) -> (number=w136:i32)  [unwired: 2 in, 1 out]
                      n94 = Decimal String To Number(string=w140) -> (number=w138:i32)  [unwired: 2 in, 1 out]
                      n95 = Build Array(w138, u32 0 ("元素"), w136) -> (w135:u32[])
                    }
                    n96 = property on="表格" class="Tbl (严格)"("Value"=w130) -> ()  [unwired: 2 in, 2 out]
                    n97 = Index Array(array=w131, index=0 ("索引")) -> (element=w127:i32)
                    n98 = Decrement(x=w127) -> (x-1=w126:i32)
                    "当前显示表格总行数" <- w126
                    n99 = Delete From Array "删除数组元素"(array=w129, index (row)=w126) -> (array with subset deleted=→"CANBURF":u32[][])  [unwired: 2 in, 1 out]
                  }
                }
              }
            }
          }
          frame "Process" {
            n100 = property on="表格" class="Tbl (严格)"() -> ("Selection Start"=w148:T1)  [unwired: 2 in, 2 out]
            n101 = Unbundle By Name(w148) -> ("Column"=w146:i32, "Row"=w145:i32)
            n102 = property on="表格" class="Tbl (严格)"() -> ("Value"=w154:string[][])  [unwired: 2 in, 2 out]
            n103 = Index Array(array=w154, index (row)=w145, index (col)=0 ("禁用的索引 (列)")) -> (element=w157:string)
            n104 = Index Array(array=w154, index (row)=w145, index (col)=3 ("禁用的索引 (列)")) -> (element=w152:string)
            n105 = local read "选择区域起始"() -> (w149:T1)
            n106 = event shown="[2] \"表格\": 值改变" {
              selector: _ -> [_ _ _ _]
              dyn-events: _ -> [_ _ _ _]
              timeout: 0 -> [_ _ _ _]
              tunnel: w145 -> [_ w167 w202 w245]
              tunnel: "设置" -> [_ w168 _ w246]
              tunnel: w146 -> [_ _ w199 _]
              event Timeout {
                n107 = event-data() -> ()  [unwired: 1 in, 3 out]
              }
              event "确定按钮": Value Change {
                # "本结构实现参数设置"
                n108 = event-data() -> ()  [unwired: 1 in, 3 out]
                n109 = Two Button Dialog(message="确定更改" ("消息"), 1:"否" ("F按钮名称（“取消”）"), 2:"是" ("T按钮名称（“确定”）")) -> (T button?=w166:bool)
                n110 = case shown="真" w166 {
                  tunnel: w168 -> [_ w188]
                  tunnel: w167 -> [_ w175]
                  frame False {
                  }
                  frame True {
                    # "捆绑发送数据时，地址在前，数据在后。"
                    n111 = Fract/Exp String To Number(string=w188) -> (number=w185:dbl)  [unwired: 3 in, 1 out]
                    n112 = property on="表格" class="Tbl (严格)"() -> ("Value"=w176:string[][])  [unwired: 2 in, 2 out]
                    n113 = invoke on="表格" class="Tbl (严格)" method="Set Cell Value"("X Index"=3 ("X索引"), "Y Index"=w175, "Value"=w188) -> ()  [unwired: 3 in, 6 out]
                    n114 = Index Array(array=w176, index (row)=w175, index (col)=1 ("禁用的索引 (列)")) -> (element=w180:string)
                    n115 = Index Array(array=w176, index (row)=w175, index (col)=5 ("禁用的索引 (行)")) -> (element=w187:string)
                    n116 = Decimal String To Number(string=w180) -> (number=w179:i32)  [unwired: 2 in, 1 out]
                    n117 = Fract/Exp String To Number(string=w187) -> (number=w184:dbl)  [unwired: 3 in, 1 out]
                    n118 = Greater Than 0?(x=w184) -> (x > 0?=w186:bool)
                    n119 = case shown="真" w186 {
                      tunnel: w185 -> [w191 w195]
                      tunnel: w184 -> [_ w194]
                      tunnel: [w190 w192] -> w183
                      frame False {
                        n120 = To Quad Integer(1:w191) -> (0:w190:i64)
                      }
                      frame True {
                        n121 = Divide(x=w195, y=w194) -> (x/y=w193:dbl)
                        n122 = To Quad Integer(1:w193) -> (0:w192:i64)
                      }
                    }
                    n123 = To Unsigned Word Integer(number=w179) -> (unsigned 16bit integer=w178:u16)
                    n124 = Index Array(array=w176, index (row)=w175, index (col)=7 ("禁用的索引 (列)")) -> (element=w173:string)
                    n125 = Hexadecimal String To Number(string=w173) -> (number=w172:u32)  [unwired: 2 in, 1 out]
                    n126 = Bundle(w178, w183, "Row"=w175, w172) -> (w177:cluster{u16, i64, "Row":i32, u32})  [unwired: 1 in]
                    n127 = property on="要发送的数据" class="Clust (严格)"("Val(Sgnl)"=w177) -> ()  [unwired: 2 in, 2 out]
                  }
                }
              }
              event "表格": Value Change {
                # "本结构实现参数设置"
                n128 = event-data() -> ("OldVal"=w196:string[][], "NewVal"=w203:string[][])  [unwired: 1 in, 2 out]
                n129 = Equal?(x=w199, y=3) -> (x = y?=w197:bool)
                n130 = case shown="假" w197 {
                  tunnel: [FALSE ("T button?") w207] -> w204
                  tunnel: w196 -> [w206 _]
                  frame False {
                    n131 = property on="表格" class="Tbl (严格)"("Value"=w206) -> ()  [unwired: 2 in, 2 out]
                  }
                  frame True {
                    n132 = Two Button Dialog(message="确定更改" ("消息"), 1:"否" ("F按钮名称（“取消”）"), 2:"是" ("T按钮名称（“确定”）")) -> (T button?=w207:bool)
                  }
                }
                n133 = Index Array(array=w203, index (row)=w202, index (col)=3 ("禁用的索引 (列)")) -> (element=w201:string)
                n134 = case shown="真" w204 {
                  tunnel: w201 -> [_ w227]
                  tunnel: w202 -> [_ w214]
                  frame False {
                  }
                  frame True {
                    # "捆绑发送数据时，地址在前，数据在后。"
                    n135 = Fract/Exp String To Number(string=w227) -> (number=w224:dbl)  [unwired: 3 in, 1 out]
                    n136 = property on="表格" class="Tbl (严格)"() -> ("Value"=w215:string[][])  [unwired: 2 in, 2 out]
                    n137 = invoke on="表格" class="Tbl (严格)" method="Set Cell Value"("X Index"=3 ("X索引"), "Y Index"=w214, "Value"=w227) -> ()  [unwired: 3 in, 6 out]
                    n138 = Index Array(array=w215, index (row)=w214, index (col)=1 ("禁用的索引 (列)")) -> (element=w219:string)
                    n139 = Index Array(array=w215, index (row)=w214, index (col)=5 ("禁用的索引 (行)")) -> (element=w226:string)
                    n140 = Decimal String To Number(string=w219) -> (number=w218:i32)  [unwired: 2 in, 1 out]
                    n141 = Fract/Exp String To Number(string=w226) -> (number=w223:dbl)  [unwired: 3 in, 1 out]
                    n142 = Greater Than 0?(x=w223) -> (x > 0?=w225:bool)
                    n143 = case shown="真" w225 {
                      tunnel: w224 -> [w230 w234]
                      tunnel: w223 -> [_ w233]
                      tunnel: [w229 w231] -> w222
                      frame False {
                        n144 = To Quad Integer(1:w230) -> (0:w229:i64)
                      }
                      frame True {
                        n145 = Divide(x=w234, y=w233) -> (x/y=w232:dbl)
                        n146 = To Quad Integer(1:w232) -> (0:w231:i64)
                      }
                    }
                    n147 = To Unsigned Word Integer(number=w218) -> (unsigned 16bit integer=w217:u16)
                    n148 = Index Array(array=w215, index (row)=w214, index (col)=7 ("禁用的索引 (列)")) -> (element=w212:string)
                    n149 = Hexadecimal String To Number(string=w212) -> (number=w211:u32)  [unwired: 2 in, 1 out]
                    n150 = Bundle(w217, w222, "Row"=w214, w211) -> (w216:cluster{u16, i64, "Row":i32, u32})  [unwired: 1 in]
                    n151 = property on="要发送的数据" class="Clust (严格)"("Val(Sgnl)"=w216) -> ()  [unwired: 2 in, 2 out]
                  }
                }
              }
              event Key Down {
                n152 = event-data() -> ("VKey"=w239:T7, "FocusObj"=w243:refnum<vi>)  [unwired: 1 in, 4 out]
                n153 = property on="设置" class="Str"() -> ("Text.Owner"=w242:refnum<vi>)  [unwired: 2 in, 2 out]
                n154 = Equal?(x=w239, y=eventvkey."Enter") -> (x = y?=w236:bool)
                n155 = Equal?(x=w243, y=w242) -> (x = y?=w240:bool)
                n156 = Equal?(x=w239, y=eventvkey."Return") -> (x = y?=w237:bool)
                n157 = Or(x=w237, y=w236) -> (x .or. y?=w235:bool)
                n158 = And(x=w235, y=w240) -> (x .and. y?=w241:bool)
                n159 = case shown="真" w241 {
                  tunnel: w246 -> [_ w248]
                  tunnel: w245 -> [_ w247]
                  frame False {
                  }
                  frame True {
                    n160 = Two Button Dialog(message="确定更改" ("消息"), 1:"否" ("F按钮名称（“取消”）"), 2:"是" ("T按钮名称（“确定”）")) -> (T button?=w249:bool)
                    n161 = case shown="真" w249 {
                      tunnel: w248 -> [_ w264]
                      tunnel: w247 -> [_ w254]
                      frame False {
                      }
                      frame True {
                        n162 = property on="表格" class="Tbl (严格)"() -> ("Value"=w255:string[][])  [unwired: 2 in, 2 out]
                        n163 = Fract/Exp String To Number(string=w264) -> (number=w263:dbl)  [unwired: 3 in, 1 out]
                        n164 = invoke on="表格" class="Tbl (严格)" method="Set Cell Value"("X Index"=3 ("X索引"), "Y Index"=w254, "Value"=w264) -> ()  [unwired: 3 in, 6 out]
                        n165 = Index Array(array=w255, index (row)=w254, index (col)=1 ("禁用的索引 (列)")) -> (element=w262:string)
                        n166 = Index Array(array=w255, index (row)=w254, index (col)=5 ("禁用的索引 (行)")) -> (element=w269:string)
                        n167 = Decimal String To Number(string=w262) -> (number=w260:i32)  [unwired: 2 in, 1 out]
                        n168 = Fract/Exp String To Number(string=w269) -> (number=w267:dbl)  [unwired: 3 in, 1 out]
                        n169 = Greater Than 0?(x=w267) -> (x > 0?=w268:bool)
                        n170 = To Unsigned Word Integer(number=w260) -> (unsigned 16bit integer=w259:u16)
                        n171 = case shown="真" w268 {
                          tunnel: w263 -> [w272 w276]
                          tunnel: w267 -> [_ w275]
                          tunnel: [w271 w273] -> w261
                          frame False {
                            n172 = To Quad Integer(1:w272) -> (0:w271:i64)
                          }
                          frame True {
                            n173 = Divide(x=w276, y=w275) -> (x/y=w274:dbl)
                            n174 = To Quad Integer(1:w274) -> (0:w273:i64)
                          }
                        }
                        n175 = Index Array(array=w255, index (row)=w254, index (col)=7 ("禁用的索引 (列)")) -> (element=w256:string)
                        n176 = Hexadecimal String To Number(string=w256) -> (offset past number=w253:i32)  [unwired: 2 in, 1 out]
                        n177 = Bundle(w259, w261, "Row"=w254, "offset past number"=w253) -> (w258:T10)  [unwired: 1 in]
                        n178 = property on="要发送的数据" class="Clust (严格)"("Val(Sgnl)"=w258) -> ()  [unwired: 2 in, 2 out]
                      }
                    }
                  }
                }
              }
            }
            n179 = String Subset(string=w157, length (rest)=28 ("长度（剩余）")) -> (substring=w156:string)  [unwired: 1 in]
            n180 = property on="设置" class="Str"("Caption.Text"=w156) -> ()  [unwired: 2 in, 2 out]
            n181 = Unbundle By Name(w149) -> ("Row"=w144:i32)
            n182 = Not Equal?(x=w145, y=w144) -> (x != y?=w151:bool)
            n183 = case shown="真" w151 {
              tunnel: w152 -> [_ w165]
              frame False {
              }
              frame True {
                n184 = property on="设置" class="Str"("Text.Text"=w165) -> ()  [unwired: 2 in, 2 out]
                n185 = property on="表格" class="Tbl (严格)"() -> ("Selection Start"=→"选择区域起始":T1)  [unwired: 2 in, 2 out]
              }
            }
            n186 = event shown="[1] \"选择参数表\": 值改变" {
              selector: _ -> [_ _]
              dyn-events: _ -> [_ _]
              timeout: 0 -> [_ _]
              tunnel: [FALSE TRUE] -> w163
              event Timeout {
                n187 = event-data() -> ()  [unwired: 1 in, 3 out]
              }
              event "选择参数表": Value Change {
                n188 = event-data() -> ()  [unwired: 1 in, 1 out]
              }
            }
            n189 = Select(t=ProcessState."Start" ("ProcessState"), s=w163, f=ProcessState."Process" ("ProcessState")) -> (s? t:f=w161:T2)
          }
          frame "Exit" {
            # "信号处理。信号处理引擎本身也是一个带退出的状态机"
          }
        }
      }
      frame #1 {
        n190 = stacked-sequence {
          frame #0 {
            # "布尔状态更新处理代码"
            n191 = event shown="[0] 超时" {
              selector: _ -> [_ _ _ _ _ _ _ _ _ _ _ _ _ _]
              dyn-events: _ -> [_ _ _ _ _ _ _ _ _ _ _ _ _ _]
              timeout: 0 -> [_ _ _ _ _ _ _ _ _ _ _ _ _ _]
              event Timeout {
                n192 = event-data() -> ()  [unwired: 1 in, 3 out]
                n193 = local read "延时更新布尔状态"() -> (w281:i16)
                n194 = Increment(x=w281) -> (x+1=w282:i16)
                n195 = Greater?(x=w281, y=i16 8) -> (0:w283:bool)
                n196 = case shown="真" w283 {
                  tunnel: w282 -> [w285 _]
                  frame False {
                    n197 = local write "延时更新布尔状态"(w285) -> ()
                  }
                  frame True {
                    w286 = T9 6 items=["刷新间隔", "波特率", "布尔1设置项", "布尔2设置项", "布尔3设置项", "布尔4设置项", "布尔5设置项", "显控1设置", "显控2设置", "显控3设置", "显控4设置", "显控5设置", "显控6设置", "显控7设置", "显控8设置", "显控9设置", "显控10设置", "显控11设置", "显控12设置", "设控1设置", "设控2设置", "设控3设置", "设控4设置", "设控5设置", "设控6设置", "设控7设置", "设控8设置", "曲线1设置", "曲线2设置", "曲线3设置", "曲线4设置", "曲线5设置", "曲线6设置", "曲线7设置", "曲线8设置", "曲线9设置", "曲线10设置", "曲线11设置", "曲线12设置", "曲线13设置", "曲线14设置", "曲线15设置", "曲线16设置", "ID值"] ("DataInitDef")
                    w294 = T9 5 items=["刷新间隔", "波特率", "布尔1设置项", "布尔2设置项", "布尔3设置项", "布尔4设置项", "布尔5设置项", "显控1设置", "显控2设置", "显控3设置", "显控4设置", "显控5设置", "显控6设置", "显控7设置", "显控8设置", "显控9设置", "显控10设置", "显控11设置", "显控12设置", "设控1设置", "设控2设置", "设控3设置", "设控4设置", "设控5设置", "设控6设置", "设控7设置", "设控8设置", "曲线1设置", "曲线2设置", "曲线3设置", "曲线4设置", "曲线5设置", "曲线6设置", "曲线7设置", "曲线8设置", "曲线9设置", "曲线10设置", "曲线11设置", "曲线12设置", "曲线13设置", "曲线14设置", "曲线15设置", "曲线16设置", "ID值"] ("DataInitDef")
                    w298 = T9 4 items=["刷新间隔", "波特率", "布尔1设置项", "布尔2设置项", "布尔3设置项", "布尔4设置项", "布尔5设置项", "显控1设置", "显控2设置", "显控3设置", "显控4设置", "显控5设置", "显控6设置", "显控7设置", "显控8设置", "显控9设置", "显控10设置", "显控11设置", "显控12设置", "设控1设置", "设控2设置", "设控3设置", "设控4设置", "设控5设置", "设控6设置", "设控7设置", "设控8设置", "曲线1设置", "曲线2设置", "曲线3设置", "曲线4设置", "曲线5设置", "曲线6设置", "曲线7设置", "曲线8设置", "曲线9设置", "曲线10设置", "曲线11设置", "曲线12设置", "曲线13设置", "曲线14设置", "曲线15设置", "曲线16设置", "ID值"] ("DataInitDef")
                    w302 = T9 3 items=["刷新间隔", "波特率", "布尔1设置项", "布尔2设置项", "布尔3设置项", "布尔4设置项", "布尔5设置项", "显控1设置", "显控2设置", "显控3设置", "显控4设置", "显控5设置", "显控6设置", "显控7设置", "显控8设置", "显控9设置", "显控10设置", "显控11设置", "显控12设置", "设控1设置", "设控2设置", "设控3设置", "设控4设置", "设控5设置", "设控6设置", "设控7设置", "设控8设置", "曲线1设置", "曲线2设置", "曲线3设置", "曲线4设置", "曲线5设置", "曲线6设置", "曲线7设置", "曲线8设置", "曲线9设置", "曲线10设置", "曲线11设置", "曲线12设置", "曲线13设置", "曲线14设置", "曲线15设置", "曲线16设置", "ID值"] ("DataInitDef")
                    w306 = T9 2 items=["刷新间隔", "波特率", "布尔1设置项", "布尔2设置项", "布尔3设置项", "布尔4设置项", "布尔5设置项", "显控1设置", "显控2设置", "显控3设置", "显控4设置", "显控5设置", "显控6设置", "显控7设置", "显控8设置", "显控9设置", "显控10设置", "显控11设置", "显控12设置", "设控1设置", "设控2设置", "设控3设置", "设控4设置", "设控5设置", "设控6设置", "设控7设置", "设控8设置", "曲线1设置", "曲线2设置", "曲线3设置", "曲线4设置", "曲线5设置", "曲线6设置", "曲线7设置", "曲线8设置", "曲线9设置", "曲线10设置", "曲线11设置", "曲线12设置", "曲线13设置", "曲线14设置", "曲线15设置", "曲线16设置", "ID值"] ("DataInitDef")
                    # "布尔控件状态与表格显示联动"
                    n198 = local write "延时更新布尔状态"(i16 5 ("延时更新布尔状态")) -> ()
                    n199 = local read "控件配置文件"() -> (w287:string[][])
                    n200 = Index Array(array=w287, index (row)=w286, index (col)=1 ("禁用的索引 (列)")) -> (element=w289:string)
                    n201 = Index Array(array=w287, index (row)=w306, index (col)=1 ("禁用的索引 (列)")) -> (element=w304:string)
                    n202 = Index Array(array=w287, index (row)=w302, index (col)=1 ("禁用的索引 (列)")) -> (element=w300:string)
                    n203 = Index Array(array=w287, index (row)=w298, index (col)=1 ("禁用的索引 (列)")) -> (element=w296:string)
                    n204 = Index Array(array=w287, index (row)=w294, index (col)=1 ("禁用的索引 (列)")) -> (element=w292:string)
                    n205 = call "字符串比对X.vi"("字符串"=w289) -> ("布尔"=w290:bool)  [unwired: 10 in]
                    n206 = call "字符串比对X.vi"("字符串"=w304) -> ("布尔"=w305:bool)  [unwired: 10 in]
                    n207 = call "字符串比对X.vi"("字符串"=w300) -> ("布尔"=w301:bool)  [unwired: 10 in]
                    n208 = local read "表格"() -> (w291:string[][])
                    n209 = call "字符串比对X.vi"("字符串"=w296) -> ("布尔"=w297:bool)  [unwired: 10 in]
                    n210 = call "字符串比对X.vi"("字符串"=w292) -> ("布尔"=w293:bool)  [unwired: 10 in]
                    n211 = case shown="真" w305 {
                      tunnel: w291 -> [_ w346]
                      tunnel: w304 -> [_ w345]
                      frame False {
                      }
                      frame True {
                        n212 = Decimal String To Number(string=w345) -> (number=w347:i32)  [unwired: 2 in, 1 out]
                        n213 = Index Array(array=w346, index (row)=w347, index (col)=2 ("禁用的索引 (列)")) -> (element=w344:string)
                        n214 = Decimal String To Number(string=w344) -> (number=w343:i32)  [unwired: 2 in, 1 out]
                        n215 = Equal?(x=1, y=w343) -> (x = y?=w342:bool)
                        n216 = property on="布尔 1" class="Bool (严格)"("Value"=w342) -> ()  [unwired: 2 in, 2 out]
                      }
                    }
                    n217 = case shown="真" w301 {
                      tunnel: w291 -> [_ w338]
                      tunnel: w300 -> [_ w337]
                      frame False {
                      }
                      frame True {
                        n218 = Decimal String To Number(string=w337) -> (number=w339:i32)  [unwired: 2 in, 1 out]
                        n219 = Index Array(array=w338, index (row)=w339, index (col)=2 ("禁用的索引 (列)")) -> (element=w336:string)
                        n220 = Decimal String To Number(string=w336) -> (number=w335:i32)  [unwired: 2 in, 1 out]
                        n221 = Equal?(x=1, y=w335) -> (x = y?=w334:bool)
                        n222 = property on="布尔 2" class="Bool (严格)"("Value"=w334) -> ()  [unwired: 2 in, 2 out]
                      }
                    }
                    n223 = case shown="真" w297 {
                      tunnel: w291 -> [_ w330]
                      tunnel: w296 -> [_ w329]
                      frame False {
                      }
                      frame True {
                        n224 = Decimal String To Number(string=w329) -> (number=w331:i32)  [unwired: 2 in, 1 out]
                        n225 = Index Array(array=w330, index (row)=w331, index (col)=2 ("禁用的索引 (列)")) -> (element=w328:string)
                        n226 = Decimal String To Number(string=w328) -> (number=w327:i32)  [unwired: 2 in, 1 out]
                        n227 = Equal?(x=1, y=w327) -> (x = y?=w326:bool)
                        n228 = property on="布尔 3" class="Bool (严格)"("Value"=w326) -> ()  [unwired: 2 in, 2 out]
                      }
                    }
                    n229 = case shown="真" w293 {
                      tunnel: w291 -> [_ w322]
                      tunnel: w292 -> [_ w321]
                      frame False {
                      }
                      frame True {
                        n230 = Decimal String To Number(string=w321) -> (number=w323:i32)  [unwired: 2 in, 1 out]
                        n231 = Index Array(array=w322, index (row)=w323, index (col)=2 ("禁用的索引 (列)")) -> (element=w320:string)
                        n232 = Decimal String To Number(string=w320) -> (number=w319:i32)  [unwired: 2 in, 1 out]
                        n233 = Equal?(x=1, y=w319) -> (x = y?=w318:bool)
                        n234 = property on="布尔 4" class="Bool (严格)"("Value"=w318) -> ()  [unwired: 2 in, 2 out]
                      }
                    }
                    n235 = case shown="真" w290 {
                      tunnel: w291 -> [_ w314]
                      tunnel: w289 -> [_ w313]
                      frame False {
                      }
                      frame True {
                        n236 = Decimal String To Number(string=w313) -> (number=w315:i32)  [unwired: 2 in, 1 out]
                        n237 = Index Array(array=w314, index (row)=w315, index (col)=2 ("禁用的索引 (列)")) -> (element=w312:string)
                        n238 = Decimal String To Number(string=w312) -> (number=w311:i32)  [unwired: 2 in, 1 out]
                        n239 = Equal?(x=1, y=w311) -> (x = y?=w310:bool)
                        n240 = property on="布尔 5" class="Bool (严格)"("Value"=w310) -> ()  [unwired: 2 in, 2 out]
                      }
                    }
                  }
                }
              }
              event "布尔 1": Value Change {
                w356 = T9 2 items=["刷新间隔", "波特率", "布尔1设置项", "布尔2设置项", "布尔3设置项", "布尔4设置项", "布尔5设置项", "显控1设置", "显控2设置", "显控3设置", "显控4设置", "显控5设置", "显控6设置", "显控7设置", "显控8设置", "显控9设置", "显控10设置", "显控11设置", "显控12设置", "设控1设置", "设控2设置", "设控3设置", "设控4设置", "设控5设置", "设控6设置", "设控7设置", "设控8设置", "曲线1设置", "曲线2设置", "曲线3设置", "曲线4设置", "曲线5设置", "曲线6设置", "曲线7设置", "曲线8设置", "曲线9设置", "曲线10设置", "曲线11设置", "曲线12设置", "曲线13设置", "曲线14设置", "曲线15设置", "曲线16设置", "ID值"] ("DataInitDef")
                n241 = event-data() -> ("NewVal"=w349:bool)  [unwired: 1 in]
                n242 = local read "控件配置文件"() -> (w355:string[][])
                n243 = Index Array(array=w355, index (row)=w356, index (col)=1 ("禁用的索引 (列)")) -> (element=w354:string)
                n244 = Not Equal?(x=w354, y="") -> (x != y?=w351:bool)
                n245 = Not Equal?(x=w354, y="X") -> (x != y?=w350:bool)
                n246 = And(x=w351, y=w350) -> (x .and. y?=w352:bool)
                n247 = case shown="真" w352 {
                  tunnel: w349 -> [_ w371]
                  tunnel: w354 -> [_ w368]
                  frame False {
                  }
                  frame True {
                    n248 = Decimal String To Number(string=w368) -> (number=w361:i32)  [unwired: 2 in, 1 out]
                    n249 = local write "延时更新布尔状态"(i16 0 ("延时更新布尔状态")) -> ()
                    n250 = property on="表格" class="Tbl (严格)"() -> ("Value"=w362:string[][])  [unwired: 2 in, 2 out]
                    n251 = Index Array(array=w362, index (row)=w361, index (col)=7 ("禁用的索引 (列)")) -> (element=w360:string)
                    n252 = Index Array(array=w362, index (row)=w361, index (col)=1 ("禁用的索引 (列)")) -> (element=w367:string)
                    n253 = Hexadecimal String To Number(string=w360) -> (number=w359:u32)  [unwired: 2 in, 1 out]
                    n254 = Decimal String To Number(string=w367) -> (number=w365:i32)  [unwired: 2 in, 1 out]
                    n255 = To Unsigned Word Integer(number=w365) -> (unsigned 16bit integer=w372:u16)
                    n256 = Boolean To (0,1)(Boolean=w371) -> (0, 1=w370:i16)
                    n257 = Bundle(w372, w370, w361, w359) -> (w369:cluster{u16, i16, i32, u32})  [unwired: 1 in]
                    n258 = property on="要发送的数据" class="Clust (严格)"("Val(Sgnl)"=w369) -> ()  [unwired: 2 in, 2 out]
                  }
                }
              }
              event "设控1": Value Change {
                w376 = T9 19 items=["刷新间隔", "波特率", "布尔1设置项", "布尔2设置项", "布尔3设置项", "布尔4设置项", "布尔5设置项", "显控1设置", "显控2设置", "显控3设置", "显控4设置", "显控5设置", "显控6设置", "显控7设置", "显控8设置", "显控9设置", "显控10设置", "显控11设置", "显控12设置", "设控1设置", "设控2设置", "设控3设置", "设控4设置", "设控5设置", "设控6设置", "设控7设置", "设控8设置", "曲线1设置", "曲线2设置", "曲线3设置", "曲线4设置", "曲线5设置", "曲线6设置", "曲线7设置", "曲线8设置", "曲线9设置", "曲线10设置", "曲线11设置", "曲线12设置", "曲线13设置", "曲线14设置", "曲线15设置", "曲线16设置", "ID值"] ("DataInitDef")
                n259 = event-data() -> ("NewVal"=w377:string)  [unwired: 1 in, 5 out]
                n260 = Two Button Dialog(message="确定修改？" ("消息")) -> (T button?=w378:bool)  [unwired: 2 in]
                n261 = local read "控件配置文件"() -> (w375:string[][])
                n262 = property on="表格" class="Tbl (严格)"() -> ("Value"=w374:string[][])  [unwired: 2 in, 2 out]
                n263 = call "设控值写入.vi"("表格"=w374, "控件配置文件"=w375, "DataInitDef"=w376, "NewVal"=w377, "布尔"=w378) -> ("输出簇"=w373:cluster{u16, i32, i32, i32})  [unwired: 10 in]
                n264 = property on="要发送的数据" class="Clust (严格)"("Val(Sgnl)"=w373) -> ()  [unwired: 2 in, 2 out]
              }
              event "设控2": Value Change {
                w382 = T9 20 items=["刷新间隔", "波特率", "布尔1设置项", "布尔2设置项", "布尔3设置项", "布尔4设置项", "布尔5设置项", "显控1设置", "显控2设置", "显控3设置", "显控4设置", "显控5设置", "显控6设置", "显控7设置", "显控8设置", "显控9设置", "显控10设置", "显控11设置", "显控12设置", "设控1设置", "设控2设置", "设控3设置", "设控4设置", "设控5设置", "设控6设置", "设控7设置", "设控8设置", "曲线1设置", "曲线2设置", "曲线3设置", "曲线4设置", "曲线5设置", "曲线6设置", "曲线7设置", "曲线8设置", "曲线9设置", "曲线10设置", "曲线11设置", "曲线12设置", "曲线13设置", "曲线14设置", "曲线15设置", "曲线16设置", "ID值"] ("DataInitDef")
                n265 = event-data() -> ("NewVal"=w381:string)  [unwired: 1 in, 5 out]
                n266 = Two Button Dialog(message="确定修改？" ("消息")) -> (T button?=w380:bool)  [unwired: 2 in]
                n267 = local read "控件配置文件"() -> (w383:string[][])
                n268 = property on="表格" class="Tbl (严格)"() -> ("Value"=w384:string[][])  [unwired: 2 in, 2 out]
                n269 = call "设控值写入.vi"("表格"=w384, "控件配置文件"=w383, "DataInitDef"=w382, "NewVal"=w381, "布尔"=w380) -> ("输出簇"=w385:cluster{u16, i32, i32, i32})  [unwired: 10 in]
                n270 = property on="要发送的数据" class="Clust (严格)"("Val(Sgnl)"=w385) -> ()  [unwired: 2 in, 2 out]
              }
              event "设控3": Value Change {
                w390 = T9 21 items=["刷新间隔", "波特率", "布尔1设置项", "布尔2设置项", "布尔3设置项", "布尔4设置项", "布尔5设置项", "显控1设置", "显控2设置", "显控3设置", "显控4设置", "显控5设置", "显控6设置", "显控7设置", "显控8设置", "显控9设置", "显控10设置", "显控11设置", "显控12设置", "设控1设置", "设控2设置", "设控3设置", "设控4设置", "设控5设置", "设控6设置", "设控7设置", "设控8设置", "曲线1设置", "曲线2设置", "曲线3设置", "曲线4设置", "曲线5设置", "曲线6设置", "曲线7设置", "曲线8设置", "曲线9设置", "曲线10设置", "曲线11设置", "曲线12设置", "曲线13设置", "曲线14设置", "曲线15设置", "曲线16设置", "ID值"] ("DataInitDef")
                n271 = event-data() -> ("NewVal"=w389:string)  [unwired: 1 in, 5 out]
                n272 = Two Button Dialog(message="确定修改？" ("消息")) -> (T button?=w388:bool)  [unwired: 2 in]
                n273 = local read "控件配置文件"() -> (w391:string[][])
                n274 = property on="表格" class="Tbl (严格)"() -> ("Value"=w392:string[][])  [unwired: 2 in, 2 out]
                n275 = call "设控值写入.vi"("表格"=w392, "控件配置文件"=w391, "DataInitDef"=w390, "NewVal"=w389, "布尔"=w388) -> ("输出簇"=w387:cluster{u16, i32, i32, i32})  [unwired: 10 in]
                n276 = property on="要发送的数据" class="Clust (严格)"("Val(Sgnl)"=w387) -> ()  [unwired: 2 in, 2 out]
              }
              event "设控4": Value Change {
                w397 = T9 22 items=["刷新间隔", "波特率", "布尔1设置项", "布尔2设置项", "布尔3设置项", "布尔4设置项", "布尔5设置项", "显控1设置", "显控2设置", "显控3设置", "显控4设置", "显控5设置", "显控6设置", "显控7设置", "显控8设置", "显控9设置", "显控10设置", "显控11设置", "显控12设置", "设控1设置", "设控2设置", "设控3设置", "设控4设置", "设控5设置", "设控6设置", "设控7设置", "设控8设置", "曲线1设置", "曲线2设置", "曲线3设置", "曲线4设置", "曲线5设置", "曲线6设置", "曲线7设置", "曲线8设置", "曲线9设置", "曲线10设置", "曲线11设置", "曲线12设置", "曲线13设置", "曲线14设置", "曲线15设置", "曲线16设置", "ID值"] ("DataInitDef")
                n277 = event-data() -> ("NewVal"=w396:string)  [unwired: 1 in, 5 out]
                n278 = Two Button Dialog(message="确定修改？" ("消息")) -> (T button?=w395:bool)  [unwired: 2 in]
                n279 = local read "控件配置文件"() -> (w398:string[][])
                n280 = property on="表格" class="Tbl (严格)"() -> ("Value"=w399:string[][])  [unwired: 2 in, 2 out]
                n281 = call "设控值写入.vi"("表格"=w399, "控件配置文件"=w398, "DataInitDef"=w397, "NewVal"=w396, "布尔"=w395) -> ("输出簇"=w394:cluster{u16, i32, i32, i32})  [unwired: 10 in]
                n282 = property on="要发送的数据" class="Clust (严格)"("Val(Sgnl)"=w394) -> ()  [unwired: 2 in, 2 out]
              }
              event "设控5": Value Change {
                w403 = T9 23 items=["刷新间隔", "波特率", "布尔1设置项", "布尔2设置项", "布尔3设置项", "布尔4设置项", "布尔5设置项", "显控1设置", "显控2设置", "显控3设置", "显控4设置", "显控5设置", "显控6设置", "显控7设置", "显控8设置", "显控9设置", "显控10设置", "显控11设置", "显控12设置", "设控1设置", "设控2设置", "设控3设置", "设控4设置", "设控5设置", "设控6设置", "设控7设置", "设控8设置", "曲线1设置", "曲线2设置", "曲线3设置", "曲线4设置", "曲线5设置", "曲线6设置", "曲线7设置", "曲线8设置", "曲线9设置", "曲线10设置", "曲线11设置", "曲线12设置", "曲线13设置", "曲线14设置", "曲线15设置", "曲线16设置", "ID值"] ("DataInitDef")
                n283 = event-data() -> ("NewVal"=w402:string)  [unwired: 1 in, 5 out]
                n284 = Two Button Dialog(message="确定修改？" ("消息")) -> (T button?=w401:bool)  [unwired: 2 in]
                n285 = local read "控件配置文件"() -> (w404:string[][])
                n286 = property on="表格" class="Tbl (严格)"() -> ("Value"=w405:string[][])  [unwired: 2 in, 2 out]
                n287 = call "设控值写入.vi"("表格"=w405, "控件配置文件"=w404, "DataInitDef"=w403, "NewVal"=w402, "布尔"=w401) -> ("输出簇"=w406:cluster{u16, i32, i32, i32})  [unwired: 10 in]
                n288 = property on="要发送的数据" class="Clust (严格)"("Val(Sgnl)"=w406) -> ()  [unwired: 2 in, 2 out]
              }
              event "设控6": Value Change {
                w410 = T9 24 items=["刷新间隔", "波特率", "布尔1设置项", "布尔2设置项", "布尔3设置项", "布尔4设置项", "布尔5设置项", "显控1设置", "显控2设置", "显控3设置", "显控4设置", "显控5设置", "显控6设置", "显控7设置", "显控8设置", "显控9设置", "显控10设置", "显控11设置", "显控12设置", "设控1设置", "设控2设置", "设控3设置", "设控4设置", "设控5设置", "设控6设置", "设控7设置", "设控8设置", "曲线1设置", "曲线2设置", "曲线3设置", "曲线4设置", "曲线5设置", "曲线6设置", "曲线7设置", "曲线8设置", "曲线9设置", "曲线10设置", "曲线11设置", "曲线12设置", "曲线13设置", "曲线14设置", "曲线15设置", "曲线16设置", "ID值"] ("DataInitDef")
                n289 = event-data() -> ("NewVal"=w409:string)  [unwired: 1 in, 5 out]
                n290 = Two Button Dialog(message="确定修改？" ("消息")) -> (T button?=w408:bool)  [unwired: 2 in]
                n291 = local read "控件配置文件"() -> (w411:string[][])
                n292 = property on="表格" class="Tbl (严格)"() -> ("Value"=w412:string[][])  [unwired: 2 in, 2 out]
                n293 = call "设控值写入.vi"("表格"=w412, "控件配置文件"=w411, "DataInitDef"=w410, "NewVal"=w409, "布尔"=w408) -> ("输出簇"=w413:cluster{u16, i32, i32, i32})  [unwired: 10 in]
                n294 = property on="要发送的数据" class="Clust (严格)"("Val(Sgnl)"=w413) -> ()  [unwired: 2 in, 2 out]
              }
              event "设控7": Value Change {
                w417 = T9 25 items=["刷新间隔", "波特率", "布尔1设置项", "布尔2设置项", "布尔3设置项", "布尔4设置项", "布尔5设置项", "显控1设置", "显控2设置", "显控3设置", "显控4设置", "显控5设置", "显控6设置", "显控7设置", "显控8设置", "显控9设置", "显控10设置", "显控11设置", "显控12设置", "设控1设置", "设控2设置", "设控3设置", "设控4设置", "设控5设置", "设控6设置", "设控7设置", "设控8设置", "曲线1设置", "曲线2设置", "曲线3设置", "曲线4设置", "曲线5设置", "曲线6设置", "曲线7设置", "曲线8设置", "曲线9设置", "曲线10设置", "曲线11设置", "曲线12设置", "曲线13设置", "曲线14设置", "曲线15设置", "曲线16设置", "ID值"] ("DataInitDef")
                n295 = event-data() -> ("NewVal"=w416:string)  [unwired: 1 in, 5 out]
                n296 = Two Button Dialog(message="确定修改？" ("消息")) -> (T button?=w415:bool)  [unwired: 2 in]
                n297 = local read "控件配置文件"() -> (w418:string[][])
                n298 = property on="表格" class="Tbl (严格)"() -> ("Value"=w419:string[][])  [unwired: 2 in, 2 out]
                n299 = call "设控值写入.vi"("表格"=w419, "控件配置文件"=w418, "DataInitDef"=w417, "NewVal"=w416, "布尔"=w415) -> ("输出簇"=w420:cluster{u16, i32, i32, i32})  [unwired: 10 in]
                n300 = property on="要发送的数据" class="Clust (严格)"("Val(Sgnl)"=w420) -> ()  [unwired: 2 in, 2 out]
              }
              event "设控8": Value Change {
                w424 = T9 26 items=["刷新间隔", "波特率", "布尔1设置项", "布尔2设置项", "布尔3设置项", "布尔4设置项", "布尔5设置项", "显控1设置", "显控2设置", "显控3设置", "显控4设置", "显控5设置", "显控6设置", "显控7设置", "显控8设置", "显控9设置", "显控10设置", "显控11设置", "显控12设置", "设控1设置", "设控2设置", "设控3设置", "设控4设置", "设控5设置", "设控6设置", "设控7设置", "设控8设置", "曲线1设置", "曲线2设置", "曲线3设置", "曲线4设置", "曲线5设置", "曲线6设置", "曲线7设置", "曲线8设置", "曲线9设置", "曲线10设置", "曲线11设置", "曲线12设置", "曲线13设置", "曲线14设置", "曲线15设置", "曲线16设置", "ID值"] ("DataInitDef")
                n301 = event-data() -> ("NewVal"=w423:string)  [unwired: 1 in, 5 out]
                n302 = Two Button Dialog(message="确定修改？" ("消息")) -> (T button?=w422:bool)  [unwired: 2 in]
                n303 = local read "控件配置文件"() -> (w425:string[][])
                n304 = property on="表格" class="Tbl (严格)"() -> ("Value"=w426:string[][])  [unwired: 2 in, 2 out]
                n305 = call "设控值写入.vi"("表格"=w426, "控件配置文件"=w425, "DataInitDef"=w424, "NewVal"=w423, "布尔"=w422) -> ("输出簇"=w427:cluster{u16, i32, i32, i32})  [unwired: 10 in]
                n306 = property on="要发送的数据" class="Clust (严格)"("Val(Sgnl)"=w427) -> ()  [unwired: 2 in, 2 out]
              }
              event "布尔 2": Value Change {
                w436 = T9 3 items=["刷新间隔", "波特率", "布尔1设置项", "布尔2设置项", "布尔3设置项", "布尔4设置项", "布尔5设置项", "显控1设置", "显控2设置", "显控3设置", "显控4设置", "显控5设置", "显控6设置", "显控7设置", "显控8设置", "显控9设置", "显控10设置", "显控11设置", "显控12设置", "设控1设置", "设控2设置", "设控3设置", "设控4设置", "设控5设置", "设控6设置", "设控7设置", "设控8设置", "曲线1设置", "曲线2设置", "曲线3设置", "曲线4设置", "曲线5设置", "曲线6设置", "曲线7设置", "曲线8设置", "曲线9设置", "曲线10设置", "曲线11设置", "曲线12设置", "曲线13设置", "曲线14设置", "曲线15设置", "曲线16设置", "ID值"] ("DataInitDef")
                n307 = event-data() -> ("NewVal"=w429:bool)  [unwired: 1 in]
                n308 = local read "控件配置文件"() -> (w435:string[][])
                n309 = Index Array(array=w435, index (row)=w436, index (col)=1 ("禁用的索引 (列)")) -> (element=w434:string)
                n310 = Not Equal?(x=w434, y="") -> (x != y?=w431:bool)
                n311 = Not Equal?(x=w434, y="X") -> (x != y?=w430:bool)
                n312 = And(x=w431, y=w430) -> (x .and. y?=w432:bool)
                n313 = case shown="真" w432 {
                  tunnel: w429 -> [_ w440]
                  tunnel: w434 -> [_ w441]
                  frame False {
                  }
                  frame True {
                    n314 = local write "延时更新布尔状态"(i16 0 ("延时更新布尔状态")) -> ()
                    n315 = property on="表格" class="Tbl (严格)"() -> ("Value"=w442:string[][])  [unwired: 2 in, 2 out]
                    n316 = call "布尔数据处理.vi"("布尔输入"=w440, "行数"=w441, "表格"=w442) -> ("要发送的数据"=w439:cluster{"地址":u16, "数据":i32, "行数":i32, "ID":i32})  [unwired: 8 in]
                    n317 = property on="要发送的数据" class="Clust (严格)"("Val(Sgnl)"=w439) -> ()  [unwired: 2 in, 2 out]
                  }
                }
              }
              event "布尔 3": Value Change {
                w451 = T9 4 items=["刷新间隔", "波特率", "布尔1设置项", "布尔2设置项", "布尔3设置项", "布尔4设置项", "布尔5设置项", "显控1设置", "显控2设置", "显控3设置", "显控4设置", "显控5设置", "显控6设置", "显控7设置", "显控8设置", "显控9设置", "显控10设置", "显控11设置", "显控12设置", "设控1设置", "设控2设置", "设控3设置", "设控4设置", "设控5设置", "设控6设置", "设控7设置", "设控8设置", "曲线1设置", "曲线2设置", "曲线3设置", "曲线4设置", "曲线5设置", "曲线6设置", "曲线7设置", "曲线8设置", "曲线9设置", "曲线10设置", "曲线11设置", "曲线12设置", "曲线13设置", "曲线14设置", "曲线15设置", "曲线16设置", "ID值"] ("DataInitDef")
                n318 = event-data() -> ("NewVal"=w444:bool)  [unwired: 1 in]
                n319 = local read "控件配置文件"() -> (w450:string[][])
                n320 = Index Array(array=w450, index (row)=w451, index (col)=1 ("禁用的索引 (列)")) -> (element=w449:string)
                n321 = Not Equal?(x=w449, y="") -> (x != y?=w446:bool)
                n322 = Not Equal?(x=w449, y="X") -> (x != y?=w445:bool)
                n323 = And(x=w446, y=w445) -> (x .and. y?=w447:bool)
                n324 = case shown="真" w447 {
                  tunnel: w449 -> [_ w456]
                  tunnel: w444 -> [_ w455]
                  frame False {
                  }
                  frame True {
                    n325 = local write "延时更新布尔状态"(i16 0 ("延时更新布尔状态")) -> ()
                    n326 = property on="表格" class="Tbl (严格)"() -> ("Value"=w457:string[][])  [unwired: 2 in, 2 out]
                    n327 = call "布尔数据处理.vi"("布尔输入"=w455, "行数"=w456, "表格"=w457) -> ("要发送的数据"=w454:cluster{"地址":u16, "数据":i32, "行数":i32, "ID":i32})  [unwired: 8 in]
                    n328 = property on="要发送的数据" class="Clust (严格)"("Val(Sgnl)"=w454) -> ()  [unwired: 2 in, 2 out]
                  }
                }
              }
              event "布尔 4": Value Change {
                w462 = T9 5 items=["刷新间隔", "波特率", "布尔1设置项", "布尔2设置项", "布尔3设置项", "布尔4设置项", "布尔5设置项", "显控1设置", "显控2设置", "显控3设置", "显控4设置", "显控5设置", "显控6设置", "显控7设置", "显控8设置", "显控9设置", "显控10设置", "显控11设置", "显控12设置", "设控1设置", "设控2设置", "设控3设置", "设控4设置", "设控5设置", "设控6设置", "设控7设置", "设控8设置", "曲线1设置", "曲线2设置", "曲线3设置", "曲线4设置", "曲线5设置", "曲线6设置", "曲线7设置", "曲线8设置", "曲线9设置", "曲线10设置", "曲线11设置", "曲线12设置", "曲线13设置", "曲线14设置", "曲线15设置", "曲线16设置", "ID值"] ("DataInitDef")
                n329 = event-data() -> ("NewVal"=w459:bool)  [unwired: 1 in]
                n330 = local read "控件配置文件"() -> (w468:string[][])
                n331 = Index Array(array=w468, index (row)=w462, index (col)=1 ("禁用的索引 (列)")) -> (element=w467:string)
                n332 = Not Equal?(x=w467, y="") -> (x != y?=w465:bool)
                n333 = Not Equal?(x=w467, y="X") -> (x != y?=w464:bool)
                n334 = And(x=w465, y=w464) -> (x .and. y?=w466:bool)
                n335 = case shown="真" w466 {
                  tunnel: w459 -> [_ w470]
                  tunnel: w467 -> [_ w471]
                  frame False {
                  }
                  frame True {
                    n336 = local write "延时更新布尔状态"(i16 0 ("延时更新布尔状态")) -> ()
                    n337 = property on="表格" class="Tbl (严格)"() -> ("Value"=w472:string[][])  [unwired: 2 in, 2 out]
                    n338 = call "布尔数据处理.vi"("布尔输入"=w470, "行数"=w471, "表格"=w472) -> ("要发送的数据"=w469:cluster{"地址":u16, "数据":i32, "行数":i32, "ID":i32})  [unwired: 8 in]
                    n339 = property on="要发送的数据" class="Clust (严格)"("Val(Sgnl)"=w469) -> ()  [unwired: 2 in, 2 out]
                  }
                }
              }
              event "布尔 5": Value Change {
                w474 = T9 6 items=["刷新间隔", "波特率", "布尔1设置项", "布尔2设置项", "布尔3设置项", "布尔4设置项", "布尔5设置项", "显控1设置", "显控2设置", "显控3设置", "显控4设置", "显控5设置", "显控6设置", "显控7设置", "显控8设置", "显控9设置", "显控10设置", "显控11设置", "显控12设置", "设控1设置", "设控2设置", "设控3设置", "设控4设置", "设控5设置", "设控6设置", "设控7设置", "设控8设置", "曲线1设置", "曲线2设置", "曲线3设置", "曲线4设置", "曲线5设置", "曲线6设置", "曲线7设置", "曲线8设置", "曲线9设置", "曲线10设置", "曲线11设置", "曲线12设置", "曲线13设置", "曲线14设置", "曲线15设置", "曲线16设置", "ID值"] ("DataInitDef")
                n340 = event-data() -> ("NewVal"=w475:bool)  [unwired: 1 in]
                n341 = local read "控件配置文件"() -> (w483:string[][])
                n342 = Index Array(array=w483, index (row)=w474, index (col)=1 ("禁用的索引 (列)")) -> (element=w482:string)
                n343 = Not Equal?(x=w482, y="") -> (x != y?=w480:bool)
                n344 = Not Equal?(x=w482, y="X") -> (x != y?=w479:bool)
                n345 = And(x=w480, y=w479) -> (x .and. y?=w481:bool)
                n346 = case shown="真" w481 {
                  tunnel: w475 -> [_ w485]
                  tunnel: w482 -> [_ w486]
                  frame False {
                  }
                  frame True {
                    n347 = local write "延时更新布尔状态"(i16 0 ("延时更新布尔状态")) -> ()
                    n348 = property on="表格" class="Tbl (严格)"() -> ("Value"=w487:string[][])  [unwired: 2 in, 2 out]
                    n349 = call "布尔数据处理.vi"("布尔输入"=w485, "行数"=w486, "表格"=w487) -> ("要发送的数据"=w484:cluster{"地址":u16, "数据":i32, "行数":i32, "ID":i32})  [unwired: 8 in]
                    n350 = property on="要发送的数据" class="Clust (严格)"("Val(Sgnl)"=w484) -> ()  [unwired: 2 in, 2 out]
                  }
                }
              }
            }
          }
          frame #1 {
            # "处理表格右键关联的代码"
            n351 = event "事件结构" shown="[1] \"表格\": 快捷菜单选择（用户）" {
              selector: _ -> [_ _]
              dyn-events: _ -> [_ _]
              timeout: 0 -> [_ _]
              event Timeout {
                n352 = event-data() -> ()  [unwired: 1 in, 3 out]
              }
              event "表格": Shortcut Menu Selection (User) {
                # "处理关联到布尔控件的代码"
                n353 = event-data() -> ("ItemTag"=w490:string)  [unwired: 1 in, 7 out]
                n354 = case shown="\"关联到设控5\"" w490 {
                  frame "假", Default {
                  }
                  frame "关联到布控1" {
                    w498 = T9 2 items=["刷新间隔", "波特率", "布尔1设置项", "布尔2设置项", "布尔3设置项", "布尔4设置项", "布尔5设置项", "显控1设置", "显控2设置", "显控3设置", "显控4设置", "显控5设置", "显控6设置", "显控7设置", "显控8设置", "显控9设置", "显控10设置", "显控11设置", "显控12设置", "设控1设置", "设控2设置", "设控3设置", "设控4设置", "设控5设置", "设控6设置", "设控7设置", "设控8设置", "曲线1设置", "曲线2设置", "曲线3设置", "曲线4设置", "曲线5设置", "曲线6设置", "曲线7设置", "曲线8设置", "曲线9设置", "曲线10设置", "曲线11设置", "曲线12设置", "曲线13设置", "曲线14设置", "曲线15设置", "曲线16设置", "ID值"] ("DataInitDef")
                    n355 = property on="表格" class="Tbl (严格)"() -> ("Selection Start"=w500:T1)  [unwired: 2 in, 2 out]
                    n356 = Unbundle By Name(w500) -> ("Row"=w495:i32)
                    n357 = property on="表格" class="Tbl (严格)"() -> ("Value"=w501:string[][])  [unwired: 2 in, 2 out]
                    n358 = Number To Decimal String(number=w495) -> (decimal integer string=w494:string)  [unwired: 1 in]
                    n359 = Index Array(array=w501, index (row)=w495, index (col)=0 ("禁用的索引 (列)")) -> (element=w492:string)
                    n360 = String Subset(string=w492, length (rest)=10 ("长度（剩余）")) -> (substring=w491:string)  [unwired: 1 in]
                    n361 = invoke on="控件配置文件" class="Tbl (严格)" method="Set Cell Value"("X Index"=1 ("X索引"), "Y Index"=w498, "Value"=w494) -> ()  [unwired: 3 in, 6 out]
                    n362 = property on="布控1设置" class="Str"("Val(Sgnl)"=w491) -> ()  [unwired: 2 in, 2 out]
                    n363 = property on="布尔 1" class="Bool (严格)"("Caption.Text"=w491) -> ()  [unwired: 2 in, 2 out]
                    n364 = invoke on="控件配置文件" class="Tbl (严格)" method="Set Cell Value"("X Index"=0 ("X索引"), "Y Index"=w498, "Value"=w491) -> ()  [unwired: 3 in, 6 out]
                  }
                  frame "关联到布控2" {
                    w512 = T9 3 items=["刷新间隔", "波特率", "布尔1设置项", "布尔2设置项", "布尔3设置项", "布尔4设置项", "布尔5设置项", "显控1设置", "显控2设置", "显控3设置", "显控4设置", "显控5设置", "显控6设置", "显控7设置", "显控8设置", "显控9设置", "显控10设置", "显控11设置", "显控12设置", "设控1设置", "设控2设置", "设控3设置", "设控4设置", "设控5设置", "设控6设置", "设控7设置", "设控8设置", "曲线1设置", "曲线2设置", "曲线3设置", "曲线4设置", "曲线5设置", "曲线6设置", "曲线7设置", "曲线8设置", "曲线9设置", "曲线10设置", "曲线11设置", "曲线12设置", "曲线13设置", "曲线14设置", "曲线15设置", "曲线16设置", "ID值"] ("DataInitDef")
                    n365 = property on="表格" class="Tbl (严格)"() -> ("Selection Start"=w506:T1)  [unwired: 2 in, 2 out]
                    n366 = Unbundle By Name(w506) -> ("Row"=w505:i32)
                    n367 = property on="表格" class="Tbl (严格)"() -> ("Value"=w507:string[][])  [unwired: 2 in, 2 out]
                    n368 = Number To Decimal String(number=w505) -> (decimal integer string=w509:string)  [unwired: 1 in]
                    n369 = Index Array(array=w507, index (row)=w505, index (col)=0 ("禁用的索引 (列)")) -> (element=w503:string)
                    n370 = String Subset(string=w503, length (rest)=10 ("长度（剩余）")) -> (substring=w502:string)  [unwired: 1 in]
                    n371 = invoke on="控件配置文件" class="Tbl (严格)" method="Set Cell Value"("X Index"=1 ("X索引"), "Y Index"=w512, "Value"=w509) -> ()  [unwired: 3 in, 6 out]
                    n372 = property on="布尔 2" class="Bool (严格)"("Caption.Text"=w502) -> ()  [unwired: 2 in, 2 out]
                    n373 = property on="布控2设置" class="Str"("Val(Sgnl)"=w502) -> ()  [unwired: 2 in, 2 out]
                    n374 = invoke on="控件配置文件" class="Tbl (严格)" method="Set Cell Value"("X Index"=0 ("X索引"), "Y Index"=w512, "Value"=w502) -> ()  [unwired: 3 in, 6 out]
                  }
                  frame "关联到布控3" {
                    w523 = T9 4 items=["刷新间隔", "波特率", "布尔1设置项", "布尔2设置项", "布尔3设置项", "布尔4设置项", "布尔5设置项", "显控1设置", "显控2设置", "显控3设置", "显控4设置", "显控5设置", "显控6设置", "显控7设置", "显控8设置", "显控9设置", "显控10设置", "显控11设置", "显控12设置", "设控1设置", "设控2设置", "设控3设置", "设控4设置", "设控5设置", "设控6设置", "设控7设置", "设控8设置", "曲线1设置", "曲线2设置", "曲线3设置", "曲线4设置", "曲线5设置", "曲线6设置", "曲线7设置", "曲线8设置", "曲线9设置", "曲线10设置", "曲线11设置", "曲线12设置", "曲线13设置", "曲线14设置", "曲线15设置", "曲线16设置", "ID值"] ("DataInitDef")
                    n375 = property on="表格" class="Tbl (严格)"() -> ("Selection Start"=w517:T1)  [unwired: 2 in, 2 out]
                    n376 = Unbundle By Name(w517) -> ("Row"=w516:i32)
                    n377 = property on="表格" class="Tbl (严格)"() -> ("Value"=w518:string[][])  [unwired: 2 in, 2 out]
                    n378 = Number To Decimal String(number=w516) -> (decimal integer string=w520:string)  [unwired: 1 in]
                    n379 = Index Array(array=w518, index (row)=w516, index (col)=0 ("禁用的索引 (列)")) -> (element=w514:string)
                    n380 = String Subset(string=w514, length (rest)=10 ("长度（剩余）")) -> (substring=w513:string)  [unwired: 1 in]
                    n381 = invoke on="控件配置文件" class="Tbl (严格)" method="Set Cell Value"("X Index"=1 ("X索引"), "Y Index"=w523, "Value"=w520) -> ()  [unwired: 3 in, 6 out]
                    n382 = property on="布控3设置" class="Str"("Val(Sgnl)"=w513) -> ()  [unwired: 2 in, 2 out]
                    n383 = property on="布尔 3" class="Bool (严格)"("Caption.Text"=w513) -> ()  [unwired: 2 in, 2 out]
                    n384 = invoke on="控件配置文件" class="Tbl (严格)" method="Set Cell Value"("X Index"=0 ("X索引"), "Y Index"=w523, "Value"=w513) -> ()  [unwired: 3 in, 6 out]
                  }
                  frame "关联到布控4" {
                    w534 = T9 5 items=["刷新间隔", "波特率", "布尔1设置项", "布尔2设置项", "布尔3设置项", "布尔4设置项", "布尔5设置项", "显控1设置", "显控2设置", "显控3设置", "显控4设置", "显控5设置", "显控6设置", "显控7设置", "显控8设置", "显控9设置", "显控10设置", "显控11设置", "显控12设置", "设控1设置", "设控2设置", "设控3设置", "设控4设置", "设控5设置", "设控6设置", "设控7设置", "设控8设置", "曲线1设置", "曲线2设置", "曲线3设置", "曲线4设置", "曲线5设置", "曲线6设置", "曲线7设置", "曲线8设置", "曲线9设置", "曲线10设置", "曲线11设置", "曲线12设置", "曲线13设置", "曲线14设置", "曲线15设置", "曲线16设置", "ID值"] ("DataInitDef")
                    n385 = property on="表格" class="Tbl (严格)"() -> ("Selection Start"=w529:T1)  [unwired: 2 in, 2 out]
                    n386 = Unbundle By Name(w529) -> ("Row"=w527:i32)
                    n387 = property on="表格" class="Tbl (严格)"() -> ("Value"=w530:string[][])  [unwired: 2 in, 2 out]
                    n388 = Number To Decimal String(number=w527) -> (decimal integer string=w531:string)  [unwired: 1 in]
                    n389 = Index Array(array=w530, index (row)=w527, index (col)=0 ("禁用的索引 (列)")) -> (element=w526:string)
                    n390 = String Subset(string=w526, length (rest)=10 ("长度（剩余）")) -> (substring=w525:string)  [unwired: 1 in]
                    n391 = invoke on="控件配置文件" class="Tbl (严格)" method="Set Cell Value"("X Index"=1 ("X索引"), "Y Index"=w534, "Value"=w531) -> ()  [unwired: 3 in, 6 out]
                    n392 = property on="布尔 4" class="Bool (严格)"("Caption.Text"=w525) -> ()  [unwired: 2 in, 2 out]
                    n393 = property on="布控4设置" class="Str"("Val(Sgnl)"=w525) -> ()  [unwired: 2 in, 2 out]
                    n394 = invoke on="控件配置文件" class="Tbl (严格)" method="Set Cell Value"("X Index"=0 ("X索引"), "Y Index"=w534, "Value"=w525) -> ()  [unwired: 3 in, 6 out]
                  }
                  frame "关联到布控5" {
                    w535 = T9 6 items=["刷新间隔", "波特率", "布尔1设置项", "布尔2设置项", "布尔3设置项", "布尔4设置项", "布尔5设置项", "显控1设置", "显控2设置", "显控3设置", "显控4设置", "显控5设置", "显控6设置", "显控7设置", "显控8设置", "显控9设置", "显控10设置", "显控11设置", "显控12设置", "设控1设置", "设控2设置", "设控3设置", "设控4设置", "设控5设置", "设控6设置", "设控7设置", "设控8设置", "曲线1设置", "曲线2设置", "曲线3设置", "曲线4设置", "曲线5设置", "曲线6设置", "曲线7设置", "曲线8设置", "曲线9设置", "曲线10设置", "曲线11设置", "曲线12设置", "曲线13设置", "曲线14设置", "曲线15设置", "曲线16设置", "ID值"] ("DataInitDef")
                    n395 = property on="表格" class="Tbl (严格)"() -> ("Selection Start"=w543:T1)  [unwired: 2 in, 2 out]
                    n396 = Unbundle By Name(w543) -> ("Row"=w542:i32)
                    n397 = property on="表格" class="Tbl (严格)"() -> ("Value"=w544:string[][])  [unwired: 2 in, 2 out]
                    n398 = Number To Decimal String(number=w542) -> (decimal integer string=w545:string)  [unwired: 1 in]
                    n399 = Index Array(array=w544, index (row)=w542, index (col)=0 ("禁用的索引 (列)")) -> (element=w541:string)
                    n400 = String Subset(string=w541, length (rest)=10 ("长度（剩余）")) -> (substring=w540:string)  [unwired: 1 in]
                    n401 = invoke on="控件配置文件" class="Tbl (严格)" method="Set Cell Value"("X Index"=1 ("X索引"), "Y Index"=w535, "Value"=w545) -> ()  [unwired: 3 in, 6 out]
                    n402 = property on="布尔 5" class="Bool (严格)"("Caption.Text"=w540) -> ()  [unwired: 2 in, 2 out]
                    n403 = property on="布控5设置" class="Str"("Val(Sgnl)"=w540) -> ()  [unwired: 2 in, 2 out]
                    n404 = invoke on="控件配置文件" class="Tbl (严格)" method="Set Cell Value"("X Index"=0 ("X索引"), "Y Index"=w535, "Value"=w540) -> ()  [unwired: 3 in, 6 out]
                  }
                  frame "关联到显控1" {
                    w552 = T9 7 items=["刷新间隔", "波特率", "布尔1设置项", "布尔2设置项", "布尔3设置项", "布尔4设置项", "布尔5设置项", "显控1设置", "显控2设置", "显控3设置", "显控4设置", "显控5设置", "显控6设置", "显控7设置", "显控8设置", "显控9设置", "显控10设置", "显控11设置", "显控12设置", "设控1设置", "设控2设置", "设控3设置", "设控4设置", "设控5设置", "设控6设置", "设控7设置", "设控8设置", "曲线1设置", "曲线2设置", "曲线3设置", "曲线4设置", "曲线5设置", "曲线6设置", "曲线7设置", "曲线8设置", "曲线9设置", "曲线10设置", "曲线11设置", "曲线12设置", "曲线13设置", "曲线14设置", "曲线15设置", "曲线16设置", "ID值"] ("DataInitDef")
                    n405 = property on="表格" class="Tbl (严格)"() -> ("Selection Start"=w556:T1)  [unwired: 2 in, 2 out]
                    n406 = Unbundle By Name(w556) -> ("Row"=w553:i32)
                    n407 = property on="表格" class="Tbl (严格)"() -> ("Value"=w555:string[][])  [unwired: 2 in, 2 out]
                    n408 = Number To Decimal String(number=w553) -> (decimal integer string=w549:string)  [unwired: 1 in]
                    n409 = Index Array(array=w555, index (row)=w553, index (col)=0 ("禁用的索引 (列)")) -> (element=w547:string)
                    n410 = String Subset(string=w547, length (rest)=16 ("长度（剩余）")) -> (substring=w546:string)  [unwired: 1 in]
                    n411 = invoke on="控件配置文件" class="Tbl (严格)" method="Set Cell Value"("X Index"=1 ("X索引"), "Y Index"=w552, "Value"=w549) -> ()  [unwired: 3 in, 6 out]
                    n412 = property on="显控1设置" class="Str"("Val(Sgnl)"=w546) -> ()  [unwired: 2 in, 2 out]
                    n413 = property on="显控1" class="Str"("Caption.Text"=w546) -> ()  [unwired: 2 in, 2 out]
                    n414 = invoke on="控件配置文件" class="Tbl (严格)" method="Set Cell Value"("X Index"=0 ("X索引"), "Y Index"=w552, "Value"=w546) -> ()  [unwired: 3 in, 6 out]
                  }
                  frame "关联到显控2" {
                    w563 = T9 8 items=["刷新间隔", "波特率", "布尔1设置项", "布尔2设置项", "布尔3设置项", "布尔4设置项", "布尔5设置项", "显控1设置", "显控2设置", "显控3设置", "显控4设置", "显控5设置", "显控6设置", "显控7设置", "显控8设置", "显控9设置", "显控10设置", "显控11设置", "显控12设置", "设控1设置", "设控2设置", "设控3设置", "设控4设置", "设控5设置", "设控6设置", "设控7设置", "设控8设置", "曲线1设置", "曲线2设置", "曲线3设置", "曲线4设置", "曲线5设置", "曲线6设置", "曲线7设置", "曲线8设置", "曲线9设置", "曲线10设置", "曲线11设置", "曲线12设置", "曲线13设置", "曲线14设置", "曲线15设置", "曲线16设置", "ID值"] ("DataInitDef")
                    n415 = property on="表格" class="Tbl (严格)"() -> ("Selection Start"=w566:T1)  [unwired: 2 in, 2 out]
                    n416 = Unbundle By Name(w566) -> ("Row"=w564:i32)
                    n417 = property on="表格" class="Tbl (严格)"() -> ("Value"=w565:string[][])  [unwired: 2 in, 2 out]
                    n418 = Number To Decimal String(number=w564) -> (decimal integer string=w560:string)  [unwired: 1 in]
                    n419 = Index Array(array=w565, index (row)=w564, index (col)=0 ("禁用的索引 (列)")) -> (element=w558:string)
                    n420 = String Subset(string=w558, length (rest)=16 ("长度（剩余）")) -> (substring=w557:string)  [unwired: 1 in]
                    n421 = invoke on="控件配置文件" class="Tbl (严格)" method="Set Cell Value"("X Index"=1 ("X索引"), "Y Index"=w563, "Value"=w560) -> ()  [unwired: 3 in, 6 out]
                    n422 = property on="显控2设置" class="Str"("Val(Sgnl)"=w557) -> ()  [unwired: 2 in, 2 out]
                    n423 = property on="显控2" class="Str"("Caption.Text"=w557) -> ()  [unwired: 2 in, 2 out]
                    n424 = invoke on="控件配置文件" class="Tbl (严格)" method="Set Cell Value"("X Index"=0 ("X索引"), "Y Index"=w563, "Value"=w557) -> ()  [unwired: 3 in, 6 out]
                  }
                  frame "关联到显控3" {
                    w574 = T9 9 items=["刷新间隔", "波特率", "布尔1设置项", "布尔2设置项", "布尔3设置项", "布尔4设置项", "布尔5设置项", "显控1设置", "显控2设置", "显控3设置", "显控4设置", "显控5设置", "显控6设置", "显控7设置", "显控8设置", "显控9设置", "显控10设置", "显控11设置", "显控12设置", "设控1设置", "设控2设置", "设控3设置", "设控4设置", "设控5设置", "设控6设置", "设控7设置", "设控8设置", "曲线1设置", "曲线2设置", "曲线3设置", "曲线4设置", "曲线5设置", "曲线6设置", "曲线7设置", "曲线8设置", "曲线9设置", "曲线10设置", "曲线11设置", "曲线12设置", "曲线13设置", "曲线14设置", "曲线15设置", "曲线16设置", "ID值"] ("DataInitDef")
                    n425 = property on="表格" class="Tbl (严格)"() -> ("Selection Start"=w577:T1)  [unwired: 2 in, 2 out]
                    n426 = Unbundle By Name(w577) -> ("Row"=w575:i32)
                    n427 = property on="表格" class="Tbl (严格)"() -> ("Value"=w576:string[][])  [unwired: 2 in, 2 out]
                    n428 = Number To Decimal String(number=w575) -> (decimal integer string=w571:string)  [unwired: 1 in]
                    n429 = Index Array(array=w576, index (row)=w575, index (col)=0 ("禁用的索引 (列)")) -> (element=w569:string)
                    n430 = String Subset(string=w569, length (rest)=16 ("长度（剩余）")) -> (substring=w568:string)  [unwired: 1 in]
                    n431 = invoke on="控件配置文件" class="Tbl (严格)" method="Set Cell Value"("X Index"=1 ("X索引"), "Y Index"=w574, "Value"=w571) -> ()  [unwired: 3 in, 6 out]
                    n432 = property on="显控3设置" class="Str"("Val(Sgnl)"=w568) -> ()  [unwired: 2 in, 2 out]
                    n433 = property on="显控3" class="Str"("Caption.Text"=w568) -> ()  [unwired: 2 in, 2 out]
                    n434 = invoke on="控件配置文件" class="Tbl (严格)" method="Set Cell Value"("X Index"=0 ("X索引"), "Y Index"=w574, "Value"=w568) -> ()  [unwired: 3 in, 6 out]
                  }
                  frame "关联到显控4" {
                    w585 = T9 10 items=["刷新间隔", "波特率", "布尔1设置项", "布尔2设置项", "布尔3设置项", "布尔4设置项", "布尔5设置项", "显控1设置", "显控2设置", "显控3设置", "显控4设置", "显控5设置", "显控6设置", "显控7设置", "显控8设置", "显控9设置", "显控10设置", "显控11设置", "显控12设置", "设控1设置", "设控2设置", "设控3设置", "设控4设置", "设控5设置", "设控6设置", "设控7设置", "设控8设置", "曲线1设置", "曲线2设置", "曲线3设置", "曲线4设置", "曲线5设置", "曲线6设置", "曲线7设置", "曲线8设置", "曲线9设置", "曲线10设置", "曲线11设置", "曲线12设置", "曲线13设置", "曲线14设置", "曲线15设置", "曲线16设置", "ID值"] ("DataInitDef")
                    n435 = property on="表格" class="Tbl (严格)"() -> ("Selection Start"=w588:T1)  [unwired: 2 in, 2 out]
                    n436 = Unbundle By Name(w588) -> ("Row"=w586:i32)
                    n437 = property on="表格" class="Tbl (严格)"() -> ("Value"=w587:string[][])  [unwired: 2 in, 2 out]
                    n438 = Number To Decimal String(number=w586) -> (decimal integer string=w582:string)  [unwired: 1 in]
                    n439 = Index Array(array=w587, index (row)=w586, index (col)=0 ("禁用的索引 (列)")) -> (element=w580:string)
                    n440 = String Subset(string=w580, length (rest)=16 ("长度（剩余）")) -> (substring=w579:string)  [unwired: 1 in]
                    n441 = invoke on="控件配置文件" class="Tbl (严格)" method="Set Cell Value"("X Index"=1 ("X索引"), "Y Index"=w585, "Value"=w582) -> ()  [unwired: 3 in, 6 out]
                    n442 = property on="显控4设置" class="Str"("Val(Sgnl)"=w579) -> ()  [unwired: 2 in, 2 out]
                    n443 = property on="显控4" class="Str"("Caption.Text"=w579) -> ()  [unwired: 2 in, 2 out]
                    n444 = invoke on="控件配置文件" class="Tbl (严格)" method="Set Cell Value"("X Index"=0 ("X索引"), "Y Index"=w585, "Value"=w579) -> ()  [unwired: 3 in, 6 out]
                  }
                  frame "关联到显控5" {
                    w596 = T9 11 items=["刷新间隔", "波特率", "布尔1设置项", "布尔2设置项", "布尔3设置项", "布尔4设置项", "布尔5设置项", "显控1设置", "显控2设置", "显控3设置", "显控4设置", "显控5设置", "显控6设置", "显控7设置", "显控8设置", "显控9设置", "显控10设置", "显控11设置", "显控12设置", "设控1设置", "设控2设置", "设控3设置", "设控4设置", "设控5设置", "设控6设置", "设控7设置", "设控8设置", "曲线1设置", "曲线2设置", "曲线3设置", "曲线4设置", "曲线5设置", "曲线6设置", "曲线7设置", "曲线8设置", "曲线9设置", "曲线10设置", "曲线11设置", "曲线12设置", "曲线13设置", "曲线14设置", "曲线15设置", "曲线16设置", "ID值"] ("DataInitDef")
                    n445 = property on="表格" class="Tbl (严格)"() -> ("Selection Start"=w599:T1)  [unwired: 2 in, 2 out]
                    n446 = Unbundle By Name(w599) -> ("Row"=w597:i32)
                    n447 = property on="表格" class="Tbl (严格)"() -> ("Value"=w598:string[][])  [unwired: 2 in, 2 out]
                    n448 = Number To Decimal String(number=w597) -> (decimal integer string=w593:string)  [unwired: 1 in]
                    n449 = Index Array(array=w598, index (row)=w597, index (col)=0 ("禁用的索引 (列)")) -> (element=w591:string)
                    n450 = String Subset(string=w591, length (rest)=16 ("长度（剩余）")) -> (substring=w590:string)  [unwired: 1 in]
                    n451 = invoke on="控件配置文件" class="Tbl (严格)" method="Set Cell Value"("X Index"=1 ("X索引"), "Y Index"=w596, "Value"=w593) -> ()  [unwired: 3 in, 6 out]
                    n452 = property on="显控5设置" class="Str"("Val(Sgnl)"=w590) -> ()  [unwired: 2 in, 2 out]
                    n453 = property on="显控5" class="Str"("Caption.Text"=w590) -> ()  [unwired: 2 in, 2 out]
                    n454 = invoke on="控件配置文件" class="Tbl (严格)" method="Set Cell Value"("X Index"=0 ("X索引"), "Y Index"=w596, "Value"=w590) -> ()  [unwired: 3 in, 6 out]
                  }
                  frame "关联到显控6" {
                    w607 = T9 12 items=["刷新间隔", "波特率", "布尔1设置项", "布尔2设置项", "布尔3设置项", "布尔4设置项", "布尔5设置项", "显控1设置", "显控2设置", "显控3设置", "显控4设置", "显控5设置", "显控6设置", "显控7设置", "显控8设置", "显控9设置", "显控10设置", "显控11设置", "显控12设置", "设控1设置", "设控2设置", "设控3设置", "设控4设置", "设控5设置", "设控6设置", "设控7设置", "设控8设置", "曲线1设置", "曲线2设置", "曲线3设置", "曲线4设置", "曲线5设置", "曲线6设置", "曲线7设置", "曲线8设置", "曲线9设置", "曲线10设置", "曲线11设置", "曲线12设置", "曲线13设置", "曲线14设置", "曲线15设置", "曲线16设置", "ID值"] ("DataInitDef")
                    n455 = property on="表格" class="Tbl (严格)"() -> ("Selection Start"=w610:T1)  [unwired: 2 in, 2 out]
                    n456 = Unbundle By Name(w610) -> ("Row"=w608:i32)
                    n457 = property on="表格" class="Tbl (严格)"() -> ("Value"=w609:string[][])  [unwired: 2 in, 2 out]
                    n458 = Number To Decimal String(number=w608) -> (decimal integer string=w604:string)  [unwired: 1 in]
                    n459 = Index Array(array=w609, index (row)=w608, index (col)=0 ("禁用的索引 (列)")) -> (element=w602:string)
                    n460 = String Subset(string=w602, length (rest)=16 ("长度（剩余）")) -> (substring=w601:string)  [unwired: 1 in]
                    n461 = invoke on="控件配置文件" class="Tbl (严格)" method="Set Cell Value"("X Index"=1 ("X索引"), "Y Index"=w607, "Value"=w604) -> ()  [unwired: 3 in, 6 out]
                    n462 = property on="显控6设置" class="Str"("Val(Sgnl)"=w601) -> ()  [unwired: 2 in, 2 out]
                    n463 = property on="显控6" class="Str"("Caption.Text"=w601) -> ()  [unwired: 2 in, 2 out]
                    n464 = invoke on="控件配置文件" class="Tbl (严格)" method="Set Cell Value"("X Index"=0 ("X索引"), "Y Index"=w607, "Value"=w601) -> ()  [unwired: 3 in, 6 out]
                  }
                  frame "关联到显控7" {
                    w618 = T9 13 items=["刷新间隔", "波特率", "布尔1设置项", "布尔2设置项", "布尔3设置项", "布尔4设置项", "布尔5设置项", "显控1设置", "显控2设置", "显控3设置", "显控4设置", "显控5设置", "显控6设置", "显控7设置", "显控8设置", "显控9设置", "显控10设置", "显控11设置", "显控12设置", "设控1设置", "设控2设置", "设控3设置", "设控4设置", "设控5设置", "设控6设置", "设控7设置", "设控8设置", "曲线1设置", "曲线2设置", "曲线3设置", "曲线4设置", "曲线5设置", "曲线6设置", "曲线7设置", "曲线8设置", "曲线9设置", "曲线10设置", "曲线11设置", "曲线12设置", "曲线13设置", "曲线14设置", "曲线15设置", "曲线16设置", "ID值"] ("DataInitDef")
                    n465 = property on="表格" class="Tbl (严格)"() -> ("Selection Start"=w621:T1)  [unwired: 2 in, 2 out]
                    n466 = Unbundle By Name(w621) -> ("Row"=w619:i32)
                    n467 = property on="表格" class="Tbl (严格)"() -> ("Value"=w620:string[][])  [unwired: 2 in, 2 out]
                    n468 = Number To Decimal String(number=w619) -> (decimal integer string=w615:string)  [unwired: 1 in]
                    n469 = Index Array(array=w620, index (row)=w619, index (col)=0 ("禁用的索引 (列)")) -> (element=w613:string)
                    n470 = String Subset(string=w613, length (rest)=16 ("长度（剩余）")) -> (substring=w612:string)  [unwired: 1 in]
                    n471 = invoke on="控件配置文件" class="Tbl (严格)" method="Set Cell Value"("X Index"=1 ("X索引"), "Y Index"=w618, "Value"=w615) -> ()  [unwired: 3 in, 6 out]
                    n472 = property on="显控7设置" class="Str"("Val(Sgnl)"=w612) -> ()  [unwired: 2 in, 2 out]
                    n473 = property on="显控7" class="Str"("Caption.Text"=w612) -> ()  [unwired: 2 in, 2 out]
                    n474 = invoke on="控件配置文件" class="Tbl (严格)" method="Set Cell Value"("X Index"=0 ("X索引"), "Y Index"=w618, "Value"=w612) -> ()  [unwired: 3 in, 6 out]
                  }
                  frame "关联到显控8" {
                    w629 = T9 14 items=["刷新间隔", "波特率", "布尔1设置项", "布尔2设置项", "布尔3设置项", "布尔4设置项", "布尔5设置项", "显控1设置", "显控2设置", "显控3设置", "显控4设置", "显控5设置", "显控6设置", "显控7设置", "显控8设置", "显控9设置", "显控10设置", "显控11设置", "显控12设置", "设控1设置", "设控2设置", "设控3设置", "设控4设置", "设控5设置", "设控6设置", "设控7设置", "设控8设置", "曲线1设置", "曲线2设置", "曲线3设置", "曲线4设置", "曲线5设置", "曲线6设置", "曲线7设置", "曲线8设置", "曲线9设置", "曲线10设置", "曲线11设置", "曲线12设置", "曲线13设置", "曲线14设置", "曲线15设置", "曲线16设置", "ID值"] ("DataInitDef")
                    n475 = property on="表格" class="Tbl (严格)"() -> ("Selection Start"=w632:T1)  [unwired: 2 in, 2 out]
                    n476 = Unbundle By Name(w632) -> ("Row"=w630:i32)
                    n477 = property on="表格" class="Tbl (严格)"() -> ("Value"=w631:string[][])  [unwired: 2 in, 2 out]
                    n478 = Number To Decimal String(number=w630) -> (decimal integer string=w626:string)  [unwired: 1 in]
                    n479 = Index Array(array=w631, index (row)=w630, index (col)=0 ("禁用的索引 (列)")) -> (element=w624:string)
                    n480 = String Subset(string=w624, length (rest)=16 ("长度（剩余）")) -> (substring=w623:string)  [unwired: 1 in]
                    n481 = invoke on="控件配置文件" class="Tbl (严格)" method="Set Cell Value"("X Index"=1 ("X索引"), "Y Index"=w629, "Value"=w626) -> ()  [unwired: 3 in, 6 out]
                    n482 = property on="显控8设置" class="Str"("Val(Sgnl)"=w623) -> ()  [unwired: 2 in, 2 out]
                    n483 = property on="显控8" class="Str"("Caption.Text"=w623) -> ()  [unwired: 2 in, 2 out]
                    n484 = invoke on="控件配置文件" class="Tbl (严格)" method="Set Cell Value"("X Index"=0 ("X索引"), "Y Index"=w629, "Value"=w623) -> ()  [unwired: 3 in, 6 out]
                  }
                  frame "关联到显控9" {
                    w640 = T9 15 items=["刷新间隔", "波特率", "布尔1设置项", "布尔2设置项", "布尔3设置项", "布尔4设置项", "布尔5设置项", "显控1设置", "显控2设置", "显控3设置", "显控4设置", "显控5设置", "显控6设置", "显控7设置", "显控8设置", "显控9设置", "显控10设置", "显控11设置", "显控12设置", "设控1设置", "设控2设置", "设控3设置", "设控4设置", "设控5设置", "设控6设置", "设控7设置", "设控8设置", "曲线1设置", "曲线2设置", "曲线3设置", "曲线4设置", "曲线5设置", "曲线6设置", "曲线7设置", "曲线8设置", "曲线9设置", "曲线10设置", "曲线11设置", "曲线12设置", "曲线13设置", "曲线14设置", "曲线15设置", "曲线16设置", "ID值"] ("DataInitDef")
                    n485 = property on="表格" class="Tbl (严格)"() -> ("Selection Start"=w643:T1)  [unwired: 2 in, 2 out]
                    n486 = Unbundle By Name(w643) -> ("Row"=w641:i32)
                    n487 = property on="表格" class="Tbl (严格)"() -> ("Value"=w642:string[][])  [unwired: 2 in, 2 out]
                    n488 = Number To Decimal String(number=w641) -> (decimal integer string=w637:string)  [unwired: 1 in]
                    n489 = Index Array(array=w642, index (row)=w641, index (col)=0 ("禁用的索引 (列)")) -> (element=w635:string)
                    n490 = String Subset(string=w635, length (rest)=16 ("长度（剩余）")) -> (substring=w634:string)  [unwired: 1 in]
                    n491 = invoke on="控件配置文件" class="Tbl (严格)" method="Set Cell Value"("X Index"=1 ("X索引"), "Y Index"=w640, "Value"=w637) -> ()  [unwired: 3 in, 6 out]
                    n492 = property on="显控9设置" class="Str"("Val(Sgnl)"=w634) -> ()  [unwired: 2 in, 2 out]
                    n493 = property on="显控9" class="Str"("Caption.Text"=w634) -> ()  [unwired: 2 in, 2 out]
                    n494 = invoke on="控件配置文件" class="Tbl (严格)" method="Set Cell Value"("X Index"=0 ("X索引"), "Y Index"=w640, "Value"=w634) -> ()  [unwired: 3 in, 6 out]
                  }
                  frame "关联到显控10" {
                    w651 = T9 16 items=["刷新间隔", "波特率", "布尔1设置项", "布尔2设置项", "布尔3设置项", "布尔4设置项", "布尔5设置项", "显控1设置", "显控2设置", "显控3设置", "显控4设置", "显控5设置", "显控6设置", "显控7设置", "显控8设置", "显控9设置", "显控10设置", "显控11设置", "显控12设置", "设控1设置", "设控2设置", "设控3设置", "设控4设置", "设控5设置", "设控6设置", "设控7设置", "设控8设置", "曲线1设置", "曲线2设置", "曲线3设置", "曲线4设置", "曲线5设置", "曲线6设置", "曲线7设置", "曲线8设置", "曲线9设置", "曲线10设置", "曲线11设置", "曲线12设置", "曲线13设置", "曲线14设置", "曲线15设置", "曲线16设置", "ID值"] ("DataInitDef")
                    n495 = property on="表格" class="Tbl (严格)"() -> ("Selection Start"=w654:T1)  [unwired: 2 in, 2 out]
                    n496 = Unbundle By Name(w654) -> ("Row"=w652:i32)
                    n497 = property on="表格" class="Tbl (严格)"() -> ("Value"=w653:string[][])  [unwired: 2 in, 2 out]
                    n498 = Number To Decimal String(number=w652) -> (decimal integer string=w648:string)  [unwired: 1 in]
                    n499 = Index Array(array=w653, index (row)=w652, index (col)=0 ("禁用的索引 (列)")) -> (element=w646:string)
                    n500 = String Subset(string=w646, length (rest)=16 ("长度（剩余）")) -> (substring=w645:string)  [unwired: 1 in]
                    n501 = invoke on="控件配置文件" class="Tbl (严格)" method="Set Cell Value"("X Index"=1 ("X索引"), "Y Index"=w651, "Value"=w648) -> ()  [unwired: 3 in, 6 out]
                    n502 = property on="显控10" class="Str"("Caption.Text"=w645) -> ()  [unwired: 2 in, 2 out]
                    n503 = property on="显控10设置" class="Str"("Val(Sgnl)"=w645) -> ()  [unwired: 2 in, 2 out]
                    n504 = invoke on="控件配置文件" class="Tbl (严格)" method="Set Cell Value"("X Index"=0 ("X索引"), "Y Index"=w651, "Value"=w645) -> ()  [unwired: 3 in, 6 out]
                  }
                  frame "关联到显控11" {
                    w662 = T9 17 items=["刷新间隔", "波特率", "布尔1设置项", "布尔2设置项", "布尔3设置项", "布尔4设置项", "布尔5设置项", "显控1设置", "显控2设置", "显控3设置", "显控4设置", "显控5设置", "显控6设置", "显控7设置", "显控8设置", "显控9设置", "显控10设置", "显控11设置", "显控12设置", "设控1设置", "设控2设置", "设控3设置", "设控4设置", "设控5设置", "设控6设置", "设控7设置", "设控8设置", "曲线1设置", "曲线2设置", "曲线3设置", "曲线4设置", "曲线5设置", "曲线6设置", "曲线7设置", "曲线8设置", "曲线9设置", "曲线10设置", "曲线11设置", "曲线12设置", "曲线13设置", "曲线14设置", "曲线15设置", "曲线16设置", "ID值"] ("DataInitDef")
                    n505 = property on="表格" class="Tbl (严格)"() -> ("Selection Start"=w665:T1)  [unwired: 2 in, 2 out]
                    n506 = Unbundle By Name(w665) -> ("Row"=w663:i32)
                    n507 = property on="表格" class="Tbl (严格)"() -> ("Value"=w664:string[][])  [unwired: 2 in, 2 out]
                    n508 = Number To Decimal String(number=w663) -> (decimal integer string=w659:string)  [unwired: 1 in]
                    n509 = Index Array(array=w664, index (row)=w663, index (col)=0 ("禁用的索引 (列)")) -> (element=w657:string)
                    n510 = String Subset(string=w657, length (rest)=16 ("长度（剩余）")) -> (substring=w656:string)  [unwired: 1 in]
                    n511 = invoke on="控件配置文件" class="Tbl (严格)" method="Set Cell Value"("X Index"=1 ("X索引"), "Y Index"=w662, "Value"=w659) -> ()  [unwired: 3 in, 6 out]
                    n512 = property on="显控11" class="Str"("Caption.Text"=w656) -> ()  [unwired: 2 in, 2 out]
                    n513 = property on="显控11设置" class="Str"("Val(Sgnl)"=w656) -> ()  [unwired: 2 in, 2 out]
                    n514 = invoke on="控件配置文件" class="Tbl (严格)" method="Set Cell Value"("X Index"=0 ("X索引"), "Y Index"=w662, "Value"=w656) -> ()  [unwired: 3 in, 6 out]
                  }
                  frame "关联到显控12" {
                    w672 = T9 18 items=["刷新间隔", "波特率", "布尔1设置项", "布尔2设置项", "布尔3设置项", "布尔4设置项", "布尔5设置项", "显控1设置", "显控2设置", "显控3设置", "显控4设置", "显控5设置", "显控6设置", "显控7设置", "显控8设置", "显控9设置", "显控10设置", "显控11设置", "显控12设置", "设控1设置", "设控2设置", "设控3设置", "设控4设置", "设控5设置", "设控6设置", "设控7设置", "设控8设置", "曲线1设置", "曲线2设置", "曲线3设置", "曲线4设置", "曲线5设置", "曲线6设置", "曲线7设置", "曲线8设置", "曲线9设置", "曲线10设置", "曲线11设置", "曲线12设置", "曲线13设置", "曲线14设置", "曲线15设置", "曲线16设置", "ID值"] ("DataInitDef")
                    n515 = property on="表格" class="Tbl (严格)"() -> ("Selection Start"=w676:T1)  [unwired: 2 in, 2 out]
                    n516 = Unbundle By Name(w676) -> ("Row"=w674:i32)
                    n517 = property on="表格" class="Tbl (严格)"() -> ("Value"=w675:string[][])  [unwired: 2 in, 2 out]
                    n518 = Number To Decimal String(number=w674) -> (decimal integer string=w670:string)  [unwired: 1 in]
                    n519 = Index Array(array=w675, index (row)=w674, index (col)=0 ("禁用的索引 (列)")) -> (element=w668:string)
                    n520 = String Subset(string=w668, length (rest)=16 ("长度（剩余）")) -> (substring=w667:string)  [unwired: 1 in]
                    n521 = invoke on="控件配置文件" class="Tbl (严格)" method="Set Cell Value"("X Index"=1 ("X索引"), "Y Index"=w672, "Value"=w670) -> ()  [unwired: 3 in, 6 out]
                    n522 = property on="显控12" class="Str"("Caption.Text"=w667) -> ()  [unwired: 2 in, 2 out]
                    n523 = property on="显控12设置" class="Str"("Val(Sgnl)"=w667) -> ()  [unwired: 2 in, 2 out]
                    n524 = invoke on="控件配置文件" class="Tbl (严格)" method="Set Cell Value"("X Index"=0 ("X索引"), "Y Index"=w672, "Value"=w667) -> ()  [unwired: 3 in, 6 out]
                  }
                  frame "关联到曲线1" {
                    w688 = T9 27 items=["刷新间隔", "波特率", "布尔1设置项", "布尔2设置项", "布尔3设置项", "布尔4设置项", "布尔5设置项", "显控1设置", "显控2设置", "显控3设置", "显控4设置", "显控5设置", "显控6设置", "显控7设置", "显控8设置", "显控9设置", "显控10设置", "显控11设置", "显控12设置", "设控1设置", "设控2设置", "设控3设置", "设控4设置", "设控5设置", "设控6设置", "设控7设置", "设控8设置", "曲线1设置", "曲线2设置", "曲线3设置", "曲线4设置", "曲线5设置", "曲线6设置", "曲线7设置", "曲线8设置", "曲线9设置", "曲线10设置", "曲线11设置", "曲线12设置", "曲线13设置", "曲线14设置", "曲线15设置", "曲线16设置", "ID值"] ("DataInitDef")
                    n525 = property on="表格" class="Tbl (严格)"() -> ("Selection Start"=w686:T1)  [unwired: 2 in, 2 out]
                    n526 = Unbundle By Name(w686) -> ("Row"=w684:i32)
                    n527 = property on="表格" class="Tbl (严格)"() -> ("Value"=w685:string[][])  [unwired: 2 in, 2 out]
                    n528 = Number To Decimal String(number=w684) -> (decimal integer string=w681:string)  [unwired: 1 in]
                    n529 = Index Array(array=w685, index (row)=w684, index (col)=0 ("禁用的索引 (列)")) -> (element=w679:string)
                    n530 = String Subset(string=w679, length (rest)=16 ("长度（剩余）")) -> (substring=w678:string)  [unwired: 1 in]
                    n531 = property on="曲线1设置" class="Str"("Val(Sgnl)"=w678) -> ()  [unwired: 2 in, 2 out]
                    n532 = invoke on="控件配置文件" class="Tbl (严格)" method="Set Cell Value"("X Index"=1 ("X索引"), "Y Index"=w688, "Value"=w681) -> ()  [unwired: 3 in, 6 out]
                    n533 = invoke on="控件配置文件" class="Tbl (严格)" method="Set Cell Value"("X Index"=0 ("X索引"), "Y Index"=w688, "Value"=w678) -> ()  [unwired: 3 in, 6 out]
                  }
                  frame "关联到曲线2" {
                    w699 = T9 28 items=["刷新间隔", "波特率", "布尔1设置项", "布尔2设置项", "布尔3设置项", "布尔4设置项", "布尔5设置项", "显控1设置", "显控2设置", "显控3设置", "显控4设置", "显控5设置", "显控6设置", "显控7设置", "显控8设置", "显控9设置", "显控10设置", "显控11设置", "显控12设置", "设控1设置", "设控2设置", "设控3设置", "设控4设置", "设控5设置", "设控6设置", "设控7设置", "设控8设置", "曲线1设置", "曲线2设置", "曲线3设置", "曲线4设置", "曲线5设置", "曲线6设置", "曲线7设置", "曲线8设置", "曲线9设置", "曲线10设置", "曲线11设置", "曲线12设置", "曲线13设置", "曲线14设置", "曲线15设置", "曲线16设置", "ID值"] ("DataInitDef")
                    n534 = property on="表格" class="Tbl (严格)"() -> ("Selection Start"=w697:T1)  [unwired: 2 in, 2 out]
                    n535 = Unbundle By Name(w697) -> ("Row"=w695:i32)
                    n536 = property on="表格" class="Tbl (严格)"() -> ("Value"=w696:string[][])  [unwired: 2 in, 2 out]
                    n537 = Number To Decimal String(number=w695) -> (decimal integer string=w692:string)  [unwired: 1 in]
                    n538 = Index Array(array=w696, index (row)=w695, index (col)=0 ("禁用的索引 (列)")) -> (element=w690:string)
                    n539 = String Subset(string=w690, length (rest)=16 ("长度（剩余）")) -> (substring=w689:string)  [unwired: 1 in]
                    n540 = property on="曲线2设置" class="Str"("Val(Sgnl)"=w689) -> ()  [unwired: 2 in, 2 out]
                    n541 = invoke on="控件配置文件" class="Tbl (严格)" method="Set Cell Value"("X Index"=1 ("X索引"), "Y Index"=w699, "Value"=w692) -> ()  [unwired: 3 in, 6 out]
                    n542 = invoke on="控件配置文件" class="Tbl (严格)" method="Set Cell Value"("X Index"=0 ("X索引"), "Y Index"=w699, "Value"=w689) -> ()  [unwired: 3 in, 6 out]
                  }
                  frame "关联到曲线3" {
                    w710 = T9 29 items=["刷新间隔", "波特率", "布尔1设置项", "布尔2设置项", "布尔3设置项", "布尔4设置项", "布尔5设置项", "显控1设置", "显控2设置", "显控3设置", "显控4设置", "显控5设置", "显控6设置", "显控7设置", "显控8设置", "显控9设置", "显控10设置", "显控11设置", "显控12设置", "设控1设置", "设控2设置", "设控3设置", "设控4设置", "设控5设置", "设控6设置", "设控7设置", "设控8设置", "曲线1设置", "曲线2设置", "曲线3设置", "曲线4设置", "曲线5设置", "曲线6设置", "曲线7设置", "曲线8设置", "曲线9设置", "曲线10设置", "曲线11设置", "曲线12设置", "曲线13设置", "曲线14设置", "曲线15设置", "曲线16设置", "ID值"] ("DataInitDef")
                    n543 = property on="表格" class="Tbl (严格)"() -> ("Selection Start"=w708:T1)  [unwired: 2 in, 2 out]
                    n544 = Unbundle By Name(w708) -> ("Row"=w706:i32)
                    n545 = property on="表格" class="Tbl (严格)"() -> ("Value"=w707:string[][])  [unwired: 2 in, 2 out]
                    n546 = Number To Decimal String(number=w706) -> (decimal integer string=w703:string)  [unwired: 1 in]
                    n547 = Index Array(array=w707, index (row)=w706, index (col)=0 ("禁用的索引 (列)")) -> (element=w701:string)
                    n548 = String Subset(string=w701, length (rest)=16 ("长度（剩余）")) -> (substring=w700:string)  [unwired: 1 in]
                    n549 = property on="曲线3设置" class="Str"("Val(Sgnl)"=w700) -> ()  [unwired: 2 in, 2 out]
                    n550 = invoke on="控件配置文件" class="Tbl (严格)" method="Set Cell Value"("X Index"=1 ("X索引"), "Y Index"=w710, "Value"=w703) -> ()  [unwired: 3 in, 6 out]
                    n551 = invoke on="控件配置文件" class="Tbl (严格)" method="Set Cell Value"("X Index"=0 ("X索引"), "Y Index"=w710, "Value"=w700) -> ()  [unwired: 3 in, 6 out]
                  }
                  frame "关联到曲线4" {
                    w721 = T9 30 items=["刷新间隔", "波特率", "布尔1设置项", "布尔2设置项", "布尔3设置项", "布尔4设置项", "布尔5设置项", "显控1设置", "显控2设置", "显控3设置", "显控4设置", "显控5设置", "显控6设置", "显控7设置", "显控8设置", "显控9设置", "显控10设置", "显控11设置", "显控12设置", "设控1设置", "设控2设置", "设控3设置", "设控4设置", "设控5设置", "设控6设置", "设控7设置", "设控8设置", "曲线1设置", "曲线2设置", "曲线3设置", "曲线4设置", "曲线5设置", "曲线6设置", "曲线7设置", "曲线8设置", "曲线9设置", "曲线10设置", "曲线11设置", "曲线12设置", "曲线13设置", "曲线14设置", "曲线15设置", "曲线16设置", "ID值"] ("DataInitDef")
                    n552 = property on="表格" class="Tbl (严格)"() -> ("Selection Start"=w719:T1)  [unwired: 2 in, 2 out]
                    n553 = Unbundle By Name(w719) -> ("Row"=w717:i32)
                    n554 = property on="表格" class="Tbl (严格)"() -> ("Value"=w718:string[][])  [unwired: 2 in, 2 out]
                    n555 = Number To Decimal String(number=w717) -> (decimal integer string=w714:string)  [unwired: 1 in]
                    n556 = Index Array(array=w718, index (row)=w717, index (col)=0 ("禁用的索引 (列)")) -> (element=w712:string)
                    n557 = String Subset(string=w712, length (rest)=16 ("长度（剩余）")) -> (substring=w711:string)  [unwired: 1 in]
                    n558 = property on="曲线4设置" class="Str"("Val(Sgnl)"=w711) -> ()  [unwired: 2 in, 2 out]
                    n559 = invoke on="控件配置文件" class="Tbl (严格)" method="Set Cell Value"("X Index"=1 ("X索引"), "Y Index"=w721, "Value"=w714) -> ()  [unwired: 3 in, 6 out]
                    n560 = invoke on="控件配置文件" class="Tbl (严格)" method="Set Cell Value"("X Index"=0 ("X索引"), "Y Index"=w721, "Value"=w711) -> ()  [unwired: 3 in, 6 out]
                  }
                  frame "关联到曲线5" {
                    w732 = T9 31 items=["刷新间隔", "波特率", "布尔1设置项", "布尔2设置项", "布尔3设置项", "布尔4设置项", "布尔5设置项", "显控1设置", "显控2设置", "显控3设置", "显控4设置", "显控5设置", "显控6设置", "显控7设置", "显控8设置", "显控9设置", "显控10设置", "显控11设置", "显控12设置", "设控1设置", "设控2设置", "设控3设置", "设控4设置", "设控5设置", "设控6设置", "设控7设置", "设控8设置", "曲线1设置", "曲线2设置", "曲线3设置", "曲线4设置", "曲线5设置", "曲线6设置", "曲线7设置", "曲线8设置", "曲线9设置", "曲线10设置", "曲线11设置", "曲线12设置", "曲线13设置", "曲线14设置", "曲线15设置", "曲线16设置", "ID值"] ("DataInitDef")
                    n561 = property on="表格" class="Tbl (严格)"() -> ("Selection Start"=w730:T1)  [unwired: 2 in, 2 out]
                    n562 = Unbundle By Name(w730) -> ("Row"=w728:i32)
                    n563 = property on="表格" class="Tbl (严格)"() -> ("Value"=w729:string[][])  [unwired: 2 in, 2 out]
                    n564 = Number To Decimal String(number=w728) -> (decimal integer string=w725:string)  [unwired: 1 in]
                    n565 = Index Array(array=w729, index (row)=w728, index (col)=0 ("禁用的索引 (列)")) -> (element=w723:string)
                    n566 = String Subset(string=w723, length (rest)=16 ("长度（剩余）")) -> (substring=w722:string)  [unwired: 1 in]
                    n567 = property on="曲线5设置" class="Str"("Val(Sgnl)"=w722) -> ()  [unwired: 2 in, 2 out]
                    n568 = invoke on="控件配置文件" class="Tbl (严格)" method="Set Cell Value"("X Index"=1 ("X索引"), "Y Index"=w732, "Value"=w725) -> ()  [unwired: 3 in, 6 out]
                    n569 = invoke on="控件配置文件" class="Tbl (严格)" method="Set Cell Value"("X Index"=0 ("X索引"), "Y Index"=w732, "Value"=w722) -> ()  [unwired: 3 in, 6 out]
                  }
                  frame "关联到曲线6" {
                    w743 = T9 32 items=["刷新间隔", "波特率", "布尔1设置项", "布尔2设置项", "布尔3设置项", "布尔4设置项", "布尔5设置项", "显控1设置", "显控2设置", "显控3设置", "显控4设置", "显控5设置", "显控6设置", "显控7设置", "显控8设置", "显控9设置", "显控10设置", "显控11设置", "显控12设置", "设控1设置", "设控2设置", "设控3设置", "设控4设置", "设控5设置", "设控6设置", "设控7设置", "设控8设置", "曲线1设置", "曲线2设置", "曲线3设置", "曲线4设置", "曲线5设置", "曲线6设置", "曲线7设置", "曲线8设置", "曲线9设置", "曲线10设置", "曲线11设置", "曲线12设置", "曲线13设置", "曲线14设置", "曲线15设置", "曲线16设置", "ID值"] ("DataInitDef")
                    n570 = property on="表格" class="Tbl (严格)"() -> ("Selection Start"=w741:T1)  [unwired: 2 in, 2 out]
                    n571 = Unbundle By Name(w741) -> ("Row"=w739:i32)
                    n572 = property on="表格" class="Tbl (严格)"() -> ("Value"=w740:string[][])  [unwired: 2 in, 2 out]
                    n573 = Number To Decimal String(number=w739) -> (decimal integer string=w736:string)  [unwired: 1 in]
                    n574 = Index Array(array=w740, index (row)=w739, index (col)=0 ("禁用的索引 (列)")) -> (element=w734:string)
                    n575 = String Subset(string=w734, length (rest)=16 ("长度（剩余）")) -> (substring=w733:string)  [unwired: 1 in]
                    n576 = property on="曲线6设置" class="Str"("Val(Sgnl)"=w733) -> ()  [unwired: 2 in, 2 out]
                    n577 = invoke on="控件配置文件" class="Tbl (严格)" method="Set Cell Value"("X Index"=1 ("X索引"), "Y Index"=w743, "Value"=w736) -> ()  [unwired: 3 in, 6 out]
                    n578 = invoke on="控件配置文件" class="Tbl (严格)" method="Set Cell Value"("X Index"=0 ("X索引"), "Y Index"=w743, "Value"=w733) -> ()  [unwired: 3 in, 6 out]
                  }
                  frame "关联到曲线7" {
                    w754 = T9 33 items=["刷新间隔", "波特率", "布尔1设置项", "布尔2设置项", "布尔3设置项", "布尔4设置项", "布尔5设置项", "显控1设置", "显控2设置", "显控3设置", "显控4设置", "显控5设置", "显控6设置", "显控7设置", "显控8设置", "显控9设置", "显控10设置", "显控11设置", "显控12设置", "设控1设置", "设控2设置", "设控3设置", "设控4设置", "设控5设置", "设控6设置", "设控7设置", "设控8设置", "曲线1设置", "曲线2设置", "曲线3设置", "曲线4设置", "曲线5设置", "曲线6设置", "曲线7设置", "曲线8设置", "曲线9设置", "曲线10设置", "曲线11设置", "曲线12设置", "曲线13设置", "曲线14设置", "曲线15设置", "曲线16设置", "ID值"] ("DataInitDef")
                    n579 = property on="表格" class="Tbl (严格)"() -> ("Selection Start"=w752:T1)  [unwired: 2 in, 2 out]
                    n580 = Unbundle By Name(w752) -> ("Row"=w750:i32)
                    n581 = property on="表格" class="Tbl (严格)"() -> ("Value"=w751:string[][])  [unwired: 2 in, 2 out]
                    n582 = Number To Decimal String(number=w750) -> (decimal integer string=w747:string)  [unwired: 1 in]
                    n583 = Index Array(array=w751, index (row)=w750, index (col)=0 ("禁用的索引 (列)")) -> (element=w745:string)
                    n584 = String Subset(string=w745, length (rest)=16 ("长度（剩余）")) -> (substring=w744:string)  [unwired: 1 in]
                    n585 = property on="曲线7设置" class="Str"("Val(Sgnl)"=w744) -> ()  [unwired: 2 in, 2 out]
                    n586 = invoke on="控件配置文件" class="Tbl (严格)" method="Set Cell Value"("X Index"=1 ("X索引"), "Y Index"=w754, "Value"=w747) -> ()  [unwired: 3 in, 6 out]
                    n587 = invoke on="控件配置文件" class="Tbl (严格)" method="Set Cell Value"("X Index"=0 ("X索引"), "Y Index"=w754, "Value"=w744) -> ()  [unwired: 3 in, 6 out]
                  }
                  frame "关联到曲线8" {
                    w757 = T9 34 items=["刷新间隔", "波特率", "布尔1设置项", "布尔2设置项", "布尔3设置项", "布尔4设置项", "布尔5设置项", "显控1设置", "显控2设置", "显控3设置", "显控4设置", "显控5设置", "显控6设置", "显控7设置", "显控8设置", "显控9设置", "显控10设置", "显控11设置", "显控12设置", "设控1设置", "设控2设置", "设控3设置", "设控4设置", "设控5设置", "设控6设置", "设控7设置", "设控8设置", "曲线1设置", "曲线2设置", "曲线3设置", "曲线4设置", "曲线5设置", "曲线6设置", "曲线7设置", "曲线8设置", "曲线9设置", "曲线10设置", "曲线11设置", "曲线12设置", "曲线13设置", "曲线14设置", "曲线15设置", "曲线16设置", "ID值"] ("DataInitDef")
                    n588 = property on="表格" class="Tbl (严格)"() -> ("Selection Start"=w765:T1)  [unwired: 2 in, 2 out]
                    n589 = Unbundle By Name(w765) -> ("Row"=w763:i32)
                    n590 = property on="表格" class="Tbl (严格)"() -> ("Value"=w764:string[][])  [unwired: 2 in, 2 out]
                    n591 = Number To Decimal String(number=w763) -> (decimal integer string=w762:string)  [unwired: 1 in]
                    n592 = Index Array(array=w764, index (row)=w763, index (col)=0 ("禁用的索引 (列)")) -> (element=w761:string)
                    n593 = String Subset(string=w761, length (rest)=16 ("长度（剩余）")) -> (substring=w760:string)  [unwired: 1 in]
                    n594 = property on="曲线8设置" class="Str"("Val(Sgnl)"=w760) -> ()  [unwired: 2 in, 2 out]
                    n595 = invoke on="控件配置文件" class="Tbl (严格)" method="Set Cell Value"("X Index"=1 ("X索引"), "Y Index"=w757, "Value"=w762) -> ()  [unwired: 3 in, 6 out]
                    n596 = invoke on="控件配置文件" class="Tbl (严格)" method="Set Cell Value"("X Index"=0 ("X索引"), "Y Index"=w757, "Value"=w760) -> ()  [unwired: 3 in, 6 out]
                  }
                  frame "关联到曲线9" {
                    w776 = T9 35 items=["刷新间隔", "波特率", "布尔1设置项", "布尔2设置项", "布尔3设置项", "布尔4设置项", "布尔5设置项", "显控1设置", "显控2设置", "显控3设置", "显控4设置", "显控5设置", "显控6设置", "显控7设置", "显控8设置", "显控9设置", "显控10设置", "显控11设置", "显控12设置", "设控1设置", "设控2设置", "设控3设置", "设控4设置", "设控5设置", "设控6设置", "设控7设置", "设控8设置", "曲线1设置", "曲线2设置", "曲线3设置", "曲线4设置", "曲线5设置", "曲线6设置", "曲线7设置", "曲线8设置", "曲线9设置", "曲线10设置", "曲线11设置", "曲线12设置", "曲线13设置", "曲线14设置", "曲线15设置", "曲线16设置", "ID值"] ("DataInitDef")
                    n597 = property on="表格" class="Tbl (严格)"() -> ("Selection Start"=w775:T1)  [unwired: 2 in, 2 out]
                    n598 = Unbundle By Name(w775) -> ("Row"=w773:i32)
                    n599 = property on="表格" class="Tbl (严格)"() -> ("Value"=w774:string[][])  [unwired: 2 in, 2 out]
                    n600 = Number To Decimal String(number=w773) -> (decimal integer string=w772:string)  [unwired: 1 in]
                    n601 = Index Array(array=w774, index (row)=w773, index (col)=0 ("禁用的索引 (列)")) -> (element=w771:string)
                    n602 = String Subset(string=w771, length (rest)=16 ("长度（剩余）")) -> (substring=w770:string)  [unwired: 1 in]
                    n603 = property on="曲线9设置" class="Str"("Val(Sgnl)"=w770) -> ()  [unwired: 2 in, 2 out]
                    n604 = invoke on="控件配置文件" class="Tbl (严格)" method="Set Cell Value"("X Index"=1 ("X索引"), "Y Index"=w776, "Value"=w772) -> ()  [unwired: 3 in, 6 out]
                    n605 = invoke on="控件配置文件" class="Tbl (严格)" method="Set Cell Value"("X Index"=0 ("X索引"), "Y Index"=w776, "Value"=w770) -> ()  [unwired: 3 in, 6 out]
                  }
                  frame "关联到曲线10" {
                    w779 = T9 36 items=["刷新间隔", "波特率", "布尔1设置项", "布尔2设置项", "布尔3设置项", "布尔4设置项", "布尔5设置项", "显控1设置", "显控2设置", "显控3设置", "显控4设置", "显控5设置", "显控6设置", "显控7设置", "显控8设置", "显控9设置", "显控10设置", "显控11设置", "显控12设置", "设控1设置", "设控2设置", "设控3设置", "设控4设置", "设控5设置", "设控6设置", "设控7设置", "设控8设置", "曲线1设置", "曲线2设置", "曲线3设置", "曲线4设置", "曲线5设置", "曲线6设置", "曲线7设置", "曲线8设置", "曲线9设置", "曲线10设置", "曲线11设置", "曲线12设置", "曲线13设置", "曲线14设置", "曲线15设置", "曲线16设置", "ID值"] ("DataInitDef")
                    n606 = property on="表格" class="Tbl (严格)"() -> ("Selection Start"=w782:T1)  [unwired: 2 in, 2 out]
                    n607 = Unbundle By Name(w782) -> ("Row"=w784:i32)
                    n608 = property on="表格" class="Tbl (严格)"() -> ("Value"=w783:string[][])  [unwired: 2 in, 2 out]
                    n609 = Number To Decimal String(number=w784) -> (decimal integer string=w785:string)  [unwired: 1 in]
                    n610 = Index Array(array=w783, index (row)=w784, index (col)=0 ("禁用的索引 (列)")) -> (element=w786:string)
                    n611 = String Subset(string=w786, length (rest)=16 ("长度（剩余）")) -> (substring=w787:string)  [unwired: 1 in]
                    n612 = property on="曲线10设置" class="Str"("Val(Sgnl)"=w787) -> ()  [unwired: 2 in, 2 out]
                    n613 = invoke on="控件配置文件" class="Tbl (严格)" method="Set Cell Value"("X Index"=1 ("X索引"), "Y Index"=w779, "Value"=w785) -> ()  [unwired: 3 in, 6 out]
                    n614 = invoke on="控件配置文件" class="Tbl (严格)" method="Set Cell Value"("X Index"=0 ("X索引"), "Y Index"=w779, "Value"=w787) -> ()  [unwired: 3 in, 6 out]
                  }
                  frame "关联到曲线11" {
                    w790 = T9 37 items=["刷新间隔", "波特率", "布尔1设置项", "布尔2设置项", "布尔3设置项", "布尔4设置项", "布尔5设置项", "显控1设置", "显控2设置", "显控3设置", "显控4设置", "显控5设置", "显控6设置", "显控7设置", "显控8设置", "显控9设置", "显控10设置", "显控11设置", "显控12设置", "设控1设置", "设控2设置", "设控3设置", "设控4设置", "设控5设置", "设控6设置", "设控7设置", "设控8设置", "曲线1设置", "曲线2设置", "曲线3设置", "曲线4设置", "曲线5设置", "曲线6设置", "曲线7设置", "曲线8设置", "曲线9设置", "曲线10设置", "曲线11设置", "曲线12设置", "曲线13设置", "曲线14设置", "曲线15设置", "曲线16设置", "ID值"] ("DataInitDef")
                    n615 = property on="表格" class="Tbl (严格)"() -> ("Selection Start"=w793:T1)  [unwired: 2 in, 2 out]
                    n616 = Unbundle By Name(w793) -> ("Row"=w795:i32)
                    n617 = property on="表格" class="Tbl (严格)"() -> ("Value"=w794:string[][])  [unwired: 2 in, 2 out]
                    n618 = Number To Decimal String(number=w795) -> (decimal integer string=w796:string)  [unwired: 1 in]
                    n619 = Index Array(array=w794, index (row)=w795, index (col)=0 ("禁用的索引 (列)")) -> (element=w797:string)
                    n620 = String Subset(string=w797, length (rest)=16 ("长度（剩余）")) -> (substring=w798:string)  [unwired: 1 in]
                    n621 = property on="曲线11设置" class="Str"("Val(Sgnl)"=w798) -> ()  [unwired: 2 in, 2 out]
                    n622 = invoke on="控件配置文件" class="Tbl (严格)" method="Set Cell Value"("X Index"=1 ("X索引"), "Y Index"=w790, "Value"=w796) -> ()  [unwired: 3 in, 6 out]
                    n623 = invoke on="控件配置文件" class="Tbl (严格)" method="Set Cell Value"("X Index"=0 ("X索引"), "Y Index"=w790, "Value"=w798) -> ()  [unwired: 3 in, 6 out]
                  }
                  frame "关联到曲线12" {
                    w801 = T9 38 items=["刷新间隔", "波特率", "布尔1设置项", "布尔2设置项", "布尔3设置项", "布尔4设置项", "布尔5设置项", "显控1设置", "显控2设置", "显控3设置", "显控4设置", "显控5设置", "显控6设置", "显控7设置", "显控8设置", "显控9设置", "显控10设置", "显控11设置", "显控12设置", "设控1设置", "设控2设置", "设控3设置", "设控4设置", "设控5设置", "设控6设置", "设控7设置", "设控8设置", "曲线1设置", "曲线2设置", "曲线3设置", "曲线4设置", "曲线5设置", "曲线6设置", "曲线7设置", "曲线8设置", "曲线9设置", "曲线10设置", "曲线11设置", "曲线12设置", "曲线13设置", "曲线14设置", "曲线15设置", "曲线16设置", "ID值"] ("DataInitDef")
                    n624 = property on="表格" class="Tbl (严格)"() -> ("Selection Start"=w804:T1)  [unwired: 2 in, 2 out]
                    n625 = Unbundle By Name(w804) -> ("Row"=w806:i32)
                    n626 = property on="表格" class="Tbl (严格)"() -> ("Value"=w805:string[][])  [unwired: 2 in, 2 out]
                    n627 = Number To Decimal String(number=w806) -> (decimal integer string=w807:string)  [unwired: 1 in]
                    n628 = Index Array(array=w805, index (row)=w806, index (col)=0 ("禁用的索引 (列)")) -> (element=w808:string)
                    n629 = String Subset(string=w808, length (rest)=16 ("长度（剩余）")) -> (substring=w809:string)  [unwired: 1 in]
                    n630 = property on="曲线12设置" class="Str"("Val(Sgnl)"=w809) -> ()  [unwired: 2 in, 2 out]
                    n631 = invoke on="控件配置文件" class="Tbl (严格)" method="Set Cell Value"("X Index"=1 ("X索引"), "Y Index"=w801, "Value"=w807) -> ()  [unwired: 3 in, 6 out]
                    n632 = invoke on="控件配置文件" class="Tbl (严格)" method="Set Cell Value"("X Index"=0 ("X索引"), "Y Index"=w801, "Value"=w809) -> ()  [unwired: 3 in, 6 out]
                  }
                  frame "关联到曲线13" {
                    w812 = T9 39 items=["刷新间隔", "波特率", "布尔1设置项", "布尔2设置项", "布尔3设置项", "布尔4设置项", "布尔5设置项", "显控1设置", "显控2设置", "显控3设置", "显控4设置", "显控5设置", "显控6设置", "显控7设置", "显控8设置", "显控9设置", "显控10设置", "显控11设置", "显控12设置", "设控1设置", "设控2设置", "设控3设置", "设控4设置", "设控5设置", "设控6设置", "设控7设置", "设控8设置", "曲线1设置", "曲线2设置", "曲线3设置", "曲线4设置", "曲线5设置", "曲线6设置", "曲线7设置", "曲线8设置", "曲线9设置", "曲线10设置", "曲线11设置", "曲线12设置", "曲线13设置", "曲线14设置", "曲线15设置", "曲线16设置", "ID值"] ("DataInitDef")
                    n633 = property on="表格" class="Tbl (严格)"() -> ("Selection Start"=w815:T1)  [unwired: 2 in, 2 out]
                    n634 = Unbundle By Name(w815) -> ("Row"=w817:i32)
                    n635 = property on="表格" class="Tbl (严格)"() -> ("Value"=w816:string[][])  [unwired: 2 in, 2 out]
                    n636 = Number To Decimal String(number=w817) -> (decimal integer string=w818:string)  [unwired: 1 in]
                    n637 = Index Array(array=w816, index (row)=w817, index (col)=0 ("禁用的索引 (列)")) -> (element=w819:string)
                    n638 = String Subset(string=w819, length (rest)=16 ("长度（剩余）")) -> (substring=w820:string)  [unwired: 1 in]
                    n639 = property on="曲线13设置" class="Str"("Val(Sgnl)"=w820) -> ()  [unwired: 2 in, 2 out]
                    n640 = invoke on="控件配置文件" class="Tbl (严格)" method="Set Cell Value"("X Index"=1 ("X索引"), "Y Index"=w812, "Value"=w818) -> ()  [unwired: 3 in, 6 out]
                    n641 = invoke on="控件配置文件" class="Tbl (严格)" method="Set Cell Value"("X Index"=0 ("X索引"), "Y Index"=w812, "Value"=w820) -> ()  [unwired: 3 in, 6 out]
                  }
                  frame "关联到曲线14" {
                    w823 = T9 40 items=["刷新间隔", "波特率", "布尔1设置项", "布尔2设置项", "布尔3设置项", "布尔4设置项", "布尔5设置项", "显控1设置", "显控2设置", "显控3设置", "显控4设置", "显控5设置", "显控6设置", "显控7设置", "显控8设置", "显控9设置", "显控10设置", "显控11设置", "显控12设置", "设控1设置", "设控2设置", "设控3设置", "设控4设置", "设控5设置", "设控6设置", "设控7设置", "设控8设置", "曲线1设置", "曲线2设置", "曲线3设置", "曲线4设置", "曲线5设置", "曲线6设置", "曲线7设置", "曲线8设置", "曲线9设置", "曲线10设置", "曲线11设置", "曲线12设置", "曲线13设置", "曲线14设置", "曲线15设置", "曲线16设置", "ID值"] ("DataInitDef")
                    n642 = property on="表格" class="Tbl (严格)"() -> ("Selection Start"=w826:T1)  [unwired: 2 in, 2 out]
                    n643 = Unbundle By Name(w826) -> ("Row"=w828:i32)
                    n644 = property on="表格" class="Tbl (严格)"() -> ("Value"=w827:string[][])  [unwired: 2 in, 2 out]
                    n645 = Number To Decimal String(number=w828) -> (decimal integer string=w829:string)  [unwired: 1 in]
                    n646 = Index Array(array=w827, index (row)=w828, index (col)=0 ("禁用的索引 (列)")) -> (element=w830:string)
                    n647 = String Subset(string=w830, length (rest)=16 ("长度（剩余）")) -> (substring=w831:string)  [unwired: 1 in]
                    n648 = property on="曲线14设置" class="Str"("Val(Sgnl)"=w831) -> ()  [unwired: 2 in, 2 out]
                    n649 = invoke on="控件配置文件" class="Tbl (严格)" method="Set Cell Value"("X Index"=1 ("X索引"), "Y Index"=w823, "Value"=w829) -> ()  [unwired: 3 in, 6 out]
                    n650 = invoke on="控件配置文件" class="Tbl (严格)" method="Set Cell Value"("X Index"=0 ("X索引"), "Y Index"=w823, "Value"=w831) -> ()  [unwired: 3 in, 6 out]
                  }
                  frame "关联到曲线15" {
                    w834 = T9 41 items=["刷新间隔", "波特率", "布尔1设置项", "布尔2设置项", "布尔3设置项", "布尔4设置项", "布尔5设置项", "显控1设置", "显控2设置", "显控3设置", "显控4设置", "显控5设置", "显控6设置", "显控7设置", "显控8设置", "显控9设置", "显控10设置", "显控11设置", "显控12设置", "设控1设置", "设控2设置", "设控3设置", "设控4设置", "设控5设置", "设控6设置", "设控7设置", "设控8设置", "曲线1设置", "曲线2设置", "曲线3设置", "曲线4设置", "曲线5设置", "曲线6设置", "曲线7设置", "曲线8设置", "曲线9设置", "曲线10设置", "曲线11设置", "曲线12设置", "曲线13设置", "曲线14设置", "曲线15设置", "曲线16设置", "ID值"] ("DataInitDef")
                    n651 = property on="表格" class="Tbl (严格)"() -> ("Selection Start"=w837:T1)  [unwired: 2 in, 2 out]
                    n652 = Unbundle By Name(w837) -> ("Row"=w839:i32)
                    n653 = property on="表格" class="Tbl (严格)"() -> ("Value"=w838:string[][])  [unwired: 2 in, 2 out]
                    n654 = Number To Decimal String(number=w839) -> (decimal integer string=w840:string)  [unwired: 1 in]
                    n655 = Index Array(array=w838, index (row)=w839, index (col)=0 ("禁用的索引 (列)")) -> (element=w841:string)
                    n656 = String Subset(string=w841, length (rest)=16 ("长度（剩余）")) -> (substring=w842:string)  [unwired: 1 in]
                    n657 = property on="曲线15设置" class="Str"("Val(Sgnl)"=w842) -> ()  [unwired: 2 in, 2 out]
                    n658 = invoke on="控件配置文件" class="Tbl (严格)" method="Set Cell Value"("X Index"=1 ("X索引"), "Y Index"=w834, "Value"=w840) -> ()  [unwired: 3 in, 6 out]
                    n659 = invoke on="控件配置文件" class="Tbl (严格)" method="Set Cell Value"("X Index"=0 ("X索引"), "Y Index"=w834, "Value"=w842) -> ()  [unwired: 3 in, 6 out]
                  }
                  frame "关联到曲线16" {
                    w845 = T9 42 items=["刷新间隔", "波特率", "布尔1设置项", "布尔2设置项", "布尔3设置项", "布尔4设置项", "布尔5设置项", "显控1设置", "显控2设置", "显控3设置", "显控4设置", "显控5设置", "显控6设置", "显控7设置", "显控8设置", "显控9设置", "显控10设置", "显控11设置", "显控12设置", "设控1设置", "设控2设置", "设控3设置", "设控4设置", "设控5设置", "设控6设置", "设控7设置", "设控8设置", "曲线1设置", "曲线2设置", "曲线3设置", "曲线4设置", "曲线5设置", "曲线6设置", "曲线7设置", "曲线8设置", "曲线9设置", "曲线10设置", "曲线11设置", "曲线12设置", "曲线13设置", "曲线14设置", "曲线15设置", "曲线16设置", "ID值"] ("DataInitDef")
                    n660 = property on="表格" class="Tbl (严格)"() -> ("Selection Start"=w853:T1)  [unwired: 2 in, 2 out]
                    n661 = Unbundle By Name(w853) -> ("Row"=w851:i32)
                    n662 = property on="表格" class="Tbl (严格)"() -> ("Value"=w852:string[][])  [unwired: 2 in, 2 out]
                    n663 = Number To Decimal String(number=w851) -> (decimal integer string=w850:string)  [unwired: 1 in]
                    n664 = Index Array(array=w852, index (row)=w851, index (col)=0 ("禁用的索引 (列)")) -> (element=w849:string)
                    n665 = String Subset(string=w849, length (rest)=16 ("长度（剩余）")) -> (substring=w848:string)  [unwired: 1 in]
                    n666 = property on="曲线16设置" class="Str"("Val(Sgnl)"=w848) -> ()  [unwired: 2 in, 2 out]
                    n667 = invoke on="控件配置文件" class="Tbl (严格)" method="Set Cell Value"("X Index"=1 ("X索引"), "Y Index"=w845, "Value"=w850) -> ()  [unwired: 3 in, 6 out]
                    n668 = invoke on="控件配置文件" class="Tbl (严格)" method="Set Cell Value"("X Index"=0 ("X索引"), "Y Index"=w845, "Value"=w848) -> ()  [unwired: 3 in, 6 out]
                  }
                  frame "关联到设控1" {
                    w857 = T9 19 items=["刷新间隔", "波特率", "布尔1设置项", "布尔2设置项", "布尔3设置项", "布尔4设置项", "布尔5设置项", "显控1设置", "显控2设置", "显控3设置", "显控4设置", "显控5设置", "显控6设置", "显控7设置", "显控8设置", "显控9设置", "显控10设置", "显控11设置", "显控12设置", "设控1设置", "设控2设置", "设控3设置", "设控4设置", "设控5设置", "设控6设置", "设控7设置", "设控8设置", "曲线1设置", "曲线2设置", "曲线3设置", "曲线4设置", "曲线5设置", "曲线6设置", "曲线7设置", "曲线8设置", "曲线9设置", "曲线10设置", "曲线11设置", "曲线12设置", "曲线13设置", "曲线14设置", "曲线15设置", "曲线16设置", "ID值"] ("DataInitDef")
                    n669 = property on="表格" class="Tbl (严格)"() -> ("Selection Start"=w863:T1)  [unwired: 2 in, 2 out]
                    n670 = Unbundle By Name(w863) -> ("Row"=w861:i32)
                    n671 = property on="表格" class="Tbl (严格)"() -> ("Value"=w862:string[][])  [unwired: 2 in, 2 out]
                    n672 = Number To Decimal String(number=w861) -> (decimal integer string=w858:string)  [unwired: 1 in]
                    n673 = Index Array(array=w862, index (row)=w861, index (col)=0 ("禁用的索引 (列)")) -> (element=w855:string)
                    n674 = String Subset(string=w855, length (rest)=16 ("长度（剩余）")) -> (substring=w854:string)  [unwired: 1 in]
                    n675 = invoke on="控件配置文件" class="Tbl (严格)" method="Set Cell Value"("X Index"=1 ("X索引"), "Y Index"=w857, "Value"=w858) -> ()  [unwired: 3 in, 6 out]
                    n676 = property on="设控1" class="Str"("Caption.Text"=w854) -> ()  [unwired: 2 in, 2 out]
                    n677 = property on="设控设置 1" class="Str"("Val(Sgnl)"=w854) -> ()  [unwired: 2 in, 2 out]
                    n678 = invoke on="控件配置文件" class="Tbl (严格)" method="Set Cell Value"("X Index"=0 ("X索引"), "Y Index"=w857, "Value"=w854) -> ()  [unwired: 3 in, 6 out]
                  }
                  frame "关联到设控2" {
                    w870 = T9 20 items=["刷新间隔", "波特率", "布尔1设置项", "布尔2设置项", "布尔3设置项", "布尔4设置项", "布尔5设置项", "显控1设置", "显控2设置", "显控3设置", "显控4设置", "显控5设置", "显控6设置", "显控7设置", "显控8设置", "显控9设置", "显控10设置", "显控11设置", "显控12设置", "设控1设置", "设控2设置", "设控3设置", "设控4设置", "设控5设置", "设控6设置", "设控7设置", "设控8设置", "曲线1设置", "曲线2设置", "曲线3设置", "曲线4设置", "曲线5设置", "曲线6设置", "曲线7设置", "曲线8设置", "曲线9设置", "曲线10设置", "曲线11设置", "曲线12设置", "曲线13设置", "曲线14设置", "曲线15设置", "曲线16设置", "ID值"] ("DataInitDef")
                    n679 = property on="表格" class="Tbl (严格)"() -> ("Selection Start"=w872:T1)  [unwired: 2 in, 2 out]
                    n680 = Unbundle By Name(w872) -> ("Row"=w874:i32)
                    n681 = property on="表格" class="Tbl (严格)"() -> ("Value"=w873:string[][])  [unwired: 2 in, 2 out]
                    n682 = Number To Decimal String(number=w874) -> (decimal integer string=w875:string)  [unwired: 1 in]
                    n683 = Index Array(array=w873, index (row)=w874, index (col)=0 ("禁用的索引 (列)")) -> (element=w866:string)
                    n684 = String Subset(string=w866, length (rest)=16 ("长度（剩余）")) -> (substring=w865:string)  [unwired: 1 in]
                    n685 = invoke on="控件配置文件" class="Tbl (严格)" method="Set Cell Value"("X Index"=1 ("X索引"), "Y Index"=w870, "Value"=w875) -> ()  [unwired: 3 in, 6 out]
                    n686 = property on="设控2" class="Str"("Caption.Text"=w865) -> ()  [unwired: 2 in, 2 out]
                    n687 = property on="设控设置 2" class="Str"("Val(Sgnl)"=w865) -> ()  [unwired: 2 in, 2 out]
                    n688 = invoke on="控件配置文件" class="Tbl (严格)" method="Set Cell Value"("X Index"=0 ("X索引"), "Y Index"=w870, "Value"=w865) -> ()  [unwired: 3 in, 6 out]
                  }
                  frame "关联到设控3" {
                    w881 = T9 21 items=["刷新间隔", "波特率", "布尔1设置项", "布尔2设置项", "布尔3设置项", "布尔4设置项", "布尔5设置项", "显控1设置", "显控2设置", "显控3设置", "显控4设置", "显控5设置", "显控6设置", "显控7设置", "显控8设置", "显控9设置", "显控10设置", "显控11设置", "显控12设置", "设控1设置", "设控2设置", "设控3设置", "设控4设置", "设控5设置", "设控6设置", "设控7设置", "设控8设置", "曲线1设置", "曲线2设置", "曲线3设置", "曲线4设置", "曲线5设置", "曲线6设置", "曲线7设置", "曲线8设置", "曲线9设置", "曲线10设置", "曲线11设置", "曲线12设置", "曲线13设置", "曲线14设置", "曲线15设置", "曲线16设置", "ID值"] ("DataInitDef")
                    n689 = property on="表格" class="Tbl (严格)"() -> ("Selection Start"=w883:T1)  [unwired: 2 in, 2 out]
                    n690 = Unbundle By Name(w883) -> ("Row"=w885:i32)
                    n691 = property on="表格" class="Tbl (严格)"() -> ("Value"=w884:string[][])  [unwired: 2 in, 2 out]
                    n692 = Number To Decimal String(number=w885) -> (decimal integer string=w886:string)  [unwired: 1 in]
                    n693 = Index Array(array=w884, index (row)=w885, index (col)=0 ("禁用的索引 (列)")) -> (element=w877:string)
                    n694 = String Subset(string=w877, length (rest)=16 ("长度（剩余）")) -> (substring=w876:string)  [unwired: 1 in]
                    n695 = invoke on="控件配置文件" class="Tbl (严格)" method="Set Cell Value"("X Index"=1 ("X索引"), "Y Index"=w881, "Value"=w886) -> ()  [unwired: 3 in, 6 out]
                    n696 = property on="设控3" class="Str"("Caption.Text"=w876) -> ()  [unwired: 2 in, 2 out]
                    n697 = property on="设控设置 3" class="Str"("Val(Sgnl)"=w876) -> ()  [unwired: 2 in, 2 out]
                    n698 = invoke on="控件配置文件" class="Tbl (严格)" method="Set Cell Value"("X Index"=0 ("X索引"), "Y Index"=w881, "Value"=w876) -> ()  [unwired: 3 in, 6 out]
                  }
                  frame "关联到设控4" {
                    w892 = T9 22 items=["刷新间隔", "波特率", "布尔1设置项", "布尔2设置项", "布尔3设置项", "布尔4设置项", "布尔5设置项", "显控1设置", "显控2设置", "显控3设置", "显控4设置", "显控5设置", "显控6设置", "显控7设置", "显控8设置", "显控9设置", "显控10设置", "显控11设置", "显控12设置", "设控1设置", "设控2设置", "设控3设置", "设控4设置", "设控5设置", "设控6设置", "设控7设置", "设控8设置", "曲线1设置", "曲线2设置", "曲线3设置", "曲线4设置", "曲线5设置", "曲线6设置", "曲线7设置", "曲线8设置", "曲线9设置", "曲线10设置", "曲线11设置", "曲线12设置", "曲线13设置", "曲线14设置", "曲线15设置", "曲线16设置", "ID值"] ("DataInitDef")
                    n699 = property on="表格" class="Tbl (严格)"() -> ("Selection Start"=w897:T1)  [unwired: 2 in, 2 out]
                    n700 = Unbundle By Name(w897) -> ("Row"=w895:i32)
                    n701 = property on="表格" class="Tbl (严格)"() -> ("Value"=w896:string[][])  [unwired: 2 in, 2 out]
                    n702 = Number To Decimal String(number=w895) -> (decimal integer string=w894:string)  [unwired: 1 in]
                    n703 = Index Array(array=w896, index (row)=w895, index (col)=0 ("禁用的索引 (列)")) -> (element=w888:string)
                    n704 = String Subset(string=w888, length (rest)=16 ("长度（剩余）")) -> (substring=w887:string)  [unwired: 1 in]
                    n705 = invoke on="控件配置文件" class="Tbl (严格)" method="Set Cell Value"("X Index"=1 ("X索引"), "Y Index"=w892, "Value"=w894) -> ()  [unwired: 3 in, 6 out]
                    n706 = property on="设控4" class="Str"("Caption.Text"=w887) -> ()  [unwired: 2 in, 2 out]
                    n707 = property on="设控设置 4" class="Str"("Val(Sgnl)"=w887) -> ()  [unwired: 2 in, 2 out]
                    n708 = invoke on="控件配置文件" class="Tbl (严格)" method="Set Cell Value"("X Index"=0 ("X索引"), "Y Index"=w892, "Value"=w887) -> ()  [unwired: 3 in, 6 out]
                  }
                  frame "关联到设控5" {
                    w903 = T9 23 items=["刷新间隔", "波特率", "布尔1设置项", "布尔2设置项", "布尔3设置项", "布尔4设置项", "布尔5设置项", "显控1设置", "显控2设置", "显控3设置", "显控4设置", "显控5设置", "显控6设置", "显控7设置", "显控8设置", "显控9设置", "显控10设置", "显控11设置", "显控12设置", "设控1设置", "设控2设置", "设控3设置", "设控4设置", "设控5设置", "设控6设置", "设控7设置", "设控8设置", "曲线1设置", "曲线2设置", "曲线3设置", "曲线4设置", "曲线5设置", "曲线6设置", "曲线7设置", "曲线8设置", "曲线9设置", "曲线10设置", "曲线11设置", "曲线12设置", "曲线13设置", "曲线14设置", "曲线15设置", "曲线16设置", "ID值"] ("DataInitDef")
                    n709 = property on="表格" class="Tbl (严格)"() -> ("Selection Start"=w908:T1)  [unwired: 2 in, 2 out]
                    n710 = Unbundle By Name(w908) -> ("Row"=w906:i32)
                    n711 = property on="表格" class="Tbl (严格)"() -> ("Value"=w907:string[][])  [unwired: 2 in, 2 out]
                    n712 = Number To Decimal String(number=w906) -> (decimal integer string=w905:string)  [unwired: 1 in]
                    n713 = Index Array(array=w907, index (row)=w906, index (col)=0 ("禁用的索引 (列)")) -> (element=w899:string)
                    n714 = String Subset(string=w899, length (rest)=16 ("长度（剩余）")) -> (substring=w898:string)  [unwired: 1 in]
                    n715 = invoke on="控件配置文件" class="Tbl (严格)" method="Set Cell Value"("X Index"=1 ("X索引"), "Y Index"=w903, "Value"=w905) -> ()  [unwired: 3 in, 6 out]
                    n716 = property on="设控5" class="Str"("Caption.Text"=w898) -> ()  [unwired: 2 in, 2 out]
                    n717 = property on="设控设置 5" class="Str"("Val(Sgnl)"=w898) -> ()  [unwired: 2 in, 2 out]
                    n718 = invoke on="控件配置文件" class="Tbl (严格)" method="Set Cell Value"("X Index"=0 ("X索引"), "Y Index"=w903, "Value"=w898) -> ()  [unwired: 3 in, 6 out]
                  }
                  frame "关联到设控6" {
                    w914 = T9 24 items=["刷新间隔", "波特率", "布尔1设置项", "布尔2设置项", "布尔3设置项", "布尔4设置项", "布尔5设置项", "显控1设置", "显控2设置", "显控3设置", "显控4设置", "显控5设置", "显控6设置", "显控7设置", "显控8设置", "显控9设置", "显控10设置", "显控11设置", "显控12设置", "设控1设置", "设控2设置", "设控3设置", "设控4设置", "设控5设置", "设控6设置", "设控7设置", "设控8设置", "曲线1设置", "曲线2设置", "曲线3设置", "曲线4设置", "曲线5设置", "曲线6设置", "曲线7设置", "曲线8设置", "曲线9设置", "曲线10设置", "曲线11设置", "曲线12设置", "曲线13设置", "曲线14设置", "曲线15设置", "曲线16设置", "ID值"] ("DataInitDef")
                    n719 = property on="表格" class="Tbl (严格)"() -> ("Selection Start"=w916:T1)  [unwired: 2 in, 2 out]
                    n720 = Unbundle By Name(w916) -> ("Row"=w918:i32)
                    n721 = property on="表格" class="Tbl (严格)"() -> ("Value"=w917:string[][])  [unwired: 2 in, 2 out]
                    n722 = Number To Decimal String(number=w918) -> (decimal integer string=w919:string)  [unwired: 1 in]
                    n723 = Index Array(array=w917, index (row)=w918, index (col)=0 ("禁用的索引 (列)")) -> (element=w910:string)
                    n724 = String Subset(string=w910, length (rest)=16 ("长度（剩余）")) -> (substring=w909:string)  [unwired: 1 in]
                    n725 = invoke on="控件配置文件" class="Tbl (严格)" method="Set Cell Value"("X Index"=1 ("X索引"), "Y Index"=w914, "Value"=w919) -> ()  [unwired: 3 in, 6 out]
                    n726 = property on="设控6" class="Str"("Caption.Text"=w909) -> ()  [unwired: 2 in, 2 out]
                    n727 = property on="设控设置 6" class="Str"("Val(Sgnl)"=w909) -> ()  [unwired: 2 in, 2 out]
                    n728 = invoke on="控件配置文件" class="Tbl (严格)" method="Set Cell Value"("X Index"=0 ("X索引"), "Y Index"=w914, "Value"=w909) -> ()  [unwired: 3 in, 6 out]
                  }
                  frame "关联到设控7" {
                    w925 = T9 25 items=["刷新间隔", "波特率", "布尔1设置项", "布尔2设置项", "布尔3设置项", "布尔4设置项", "布尔5设置项", "显控1设置", "显控2设置", "显控3设置", "显控4设置", "显控5设置", "显控6设置", "显控7设置", "显控8设置", "显控9设置", "显控10设置", "显控11设置", "显控12设置", "设控1设置", "设控2设置", "设控3设置", "设控4设置", "设控5设置", "设控6设置", "设控7设置", "设控8设置", "曲线1设置", "曲线2设置", "曲线3设置", "曲线4设置", "曲线5设置", "曲线6设置", "曲线7设置", "曲线8设置", "曲线9设置", "曲线10设置", "曲线11设置", "曲线12设置", "曲线13设置", "曲线14设置", "曲线15设置", "曲线16设置", "ID值"] ("DataInitDef")
                    n729 = property on="表格" class="Tbl (严格)"() -> ("Selection Start"=w930:T1)  [unwired: 2 in, 2 out]
                    n730 = Unbundle By Name(w930) -> ("Row"=w928:i32)
                    n731 = property on="表格" class="Tbl (严格)"() -> ("Value"=w929:string[][])  [unwired: 2 in, 2 out]
                    n732 = Number To Decimal String(number=w928) -> (decimal integer string=w927:string)  [unwired: 1 in]
                    n733 = Index Array(array=w929, index (row)=w928, index (col)=0 ("禁用的索引 (列)")) -> (element=w921:string)
                    n734 = String Subset(string=w921, length (rest)=16 ("长度（剩余）")) -> (substring=w920:string)  [unwired: 1 in]
                    n735 = invoke on="控件配置文件" class="Tbl (严格)" method="Set Cell Value"("X Index"=1 ("X索引"), "Y Index"=w925, "Value"=w927) -> ()  [unwired: 3 in, 6 out]
                    n736 = property on="设控7" class="Str"("Caption.Text"=w920) -> ()  [unwired: 2 in, 2 out]
                    n737 = property on="设控设置 7" class="Str"("Val(Sgnl)"=w920) -> ()  [unwired: 2 in, 2 out]
                    n738 = invoke on="控件配置文件" class="Tbl (严格)" method="Set Cell Value"("X Index"=0 ("X索引"), "Y Index"=w925, "Value"=w920) -> ()  [unwired: 3 in, 6 out]
                  }
                  frame "关联到设控8" {
                    w936 = T9 26 items=["刷新间隔", "波特率", "布尔1设置项", "布尔2设置项", "布尔3设置项", "布尔4设置项", "布尔5设置项", "显控1设置", "显控2设置", "显控3设置", "显控4设置", "显控5设置", "显控6设置", "显控7设置", "显控8设置", "显控9设置", "显控10设置", "显控11设置", "显控12设置", "设控1设置", "设控2设置", "设控3设置", "设控4设置", "设控5设置", "设控6设置", "设控7设置", "设控8设置", "曲线1设置", "曲线2设置", "曲线3设置", "曲线4设置", "曲线5设置", "曲线6设置", "曲线7设置", "曲线8设置", "曲线9设置", "曲线10设置", "曲线11设置", "曲线12设置", "曲线13设置", "曲线14设置", "曲线15设置", "曲线16设置", "ID值"] ("DataInitDef")
                    n739 = property on="表格" class="Tbl (严格)"() -> ("Selection Start"=w938:T1)  [unwired: 2 in, 2 out]
                    n740 = Unbundle By Name(w938) -> ("Row"=w940:i32)
                    n741 = property on="表格" class="Tbl (严格)"() -> ("Value"=w939:string[][])  [unwired: 2 in, 2 out]
                    n742 = Number To Decimal String(number=w940) -> (decimal integer string=w941:string)  [unwired: 1 in]
                    n743 = Index Array(array=w939, index (row)=w940, index (col)=0 ("禁用的索引 (列)")) -> (element=w932:string)
                    n744 = String Subset(string=w932, length (rest)=16 ("长度（剩余）")) -> (substring=w931:string)  [unwired: 1 in]
                    n745 = invoke on="控件配置文件" class="Tbl (严格)" method="Set Cell Value"("X Index"=1 ("X索引"), "Y Index"=w936, "Value"=w941) -> ()  [unwired: 3 in, 6 out]
                    n746 = property on="设控8" class="Str"("Caption.Text"=w931) -> ()  [unwired: 2 in, 2 out]
                    n747 = property on="设控设置 8" class="Str"("Val(Sgnl)"=w931) -> ()  [unwired: 2 in, 2 out]
                    n748 = invoke on="控件配置文件" class="Tbl (严格)" method="Set Cell Value"("X Index"=0 ("X索引"), "Y Index"=w936, "Value"=w931) -> ()  [unwired: 3 in, 6 out]
                  }
                }
              }
            }
          }
          frame #2 {
            # "快捷菜单激活何批量EEPROM、数据导出"
            n749 = event shown="[1] 菜单选择(用户);  \"表格\": 快捷菜单选择（用户）" {
              selector: _ -> [_ _]
              dyn-events: _ -> [_ _]
              timeout: 0 -> [_ _]
              event Timeout {
                n750 = event-data() -> ()  [unwired: 1 in, 3 out]
              }
              event Menu Selection (User); "表格": Shortcut Menu Selection (User) {
                n751 = event-data() -> ("ItemTag"=w955:string)  [unwired: 1 in, 5 out]
                n752 = case shown="\"批量写入EEPROM\"" w955 {
                  frame "假", Default {
                  }
                  frame "导出参数" {
                    n753 = property on="表格" class="Tbl (严格)"() -> ("Value"=w958:string[][])  [unwired: 2 in, 2 out]
                    n754 = call <vilib>:"Application Directory.vi"() -> ("Application Directory"=w957:path)
                    n755 = call "导出参数.vi"("名称或相对路径"="Config\\导出参数列表.xltx", "基路径"=w957, "表格控件"=w958) -> ()  [unwired: 9 in]
                  }
                  frame "批量写入EEPROM" {
                    n756 = local read "刷新间隔"() -> (w965:string)
                    n757 = Decimal String To Number(string=w965) -> (number=w963:i32)  [unwired: 2 in, 1 out]
                    n758 = local read "CAN通道"() -> (w959:u8)
                    n759 = local read "ID"() -> (w960:u32)
                    n760 = Less Or Equal?(x=w963, y=1) -> (x <= y?=w961:bool)
                    n761 = Select(t=1, s=w961, f=w963) -> (s? t:f=w964:i32)
                    n762 = call "批量写入EEPROM.vi"("等待时间（毫秒）"=w964, "ID"=w960, "CAN通道"=w959) -> ()  [unwired: 8 in]
                  }
                }
              }
            }
            n763 = event shown="[1] \"波形图表\": 快捷菜单激活？" {
              selector: _ -> [_ _]
              dyn-events: _ -> [_ _]
              timeout: 0 -> [_ _]
              event Timeout {
                n764 = event-data() -> ()  [unwired: 1 in, 3 out]
              }
              event "波形图表": Shortcut Menu Activation? {
                n765 = event-data() -> ("MenuRef"=w954:refnum<k9>)  [unwired: 1 in]
                n766 = call "快捷菜单激活(波形图表).vi"("菜单引用"=w954) -> ()  [unwired: 11 in]
                n767 = event-data() -> ()  [unwired: 2 in, 1 out]
              }
            }
            n768 = event shown="[1] \"表格\": 快捷菜单激活？" {
              selector: _ -> [_ _]
              dyn-events: _ -> [_ _]
              timeout: 0 -> [_ _]
              event Timeout {
                n769 = event-data() -> ()  [unwired: 1 in, 3 out]
              }
              event "表格": Shortcut Menu Activation? {
                # "激活表格右击菜单选项"
                n770 = event-data() -> ("MenuRef"=w967:refnum<k9>)  [unwired: 1 in]
                n771 = call "快捷菜单激活(表格).vi"("菜单引用"=w967) -> ()  [unwired: 11 in]
                n772 = event-data() -> ()  [unwired: 2 in, 1 out]
              }
            }
            n773 = event shown="[1] \"布尔 1\", \"布尔 2\", \"布尔 3\", \"布尔 4\", \"布尔 5\": 快捷菜单激活？" {
              selector: _ -> [_ _ _ _ _]
              dyn-events: _ -> [_ _ _ _ _]
              timeout: 0 -> [_ _ _ _ _]
              event Timeout {
                n774 = event-data() -> ()  [unwired: 1 in, 3 out]
              }
              event "布尔 1", "布尔 2", "布尔 3", "布尔 4", "布尔 5": Shortcut Menu Activation? {
                # "撤销布尔控件的关联"
                n775 = event-data() -> ("MenuRef"=w947:refnum<k9>)  [unwired: 1 in, 3 out]
                n776 = Insert Menu Items(8:string[] ["撤销关联"] ("项名称"), 9:w947) -> ()  [unwired: 4 in, 3 out]
                n777 = event-data() -> ()  [unwired: 2 in, 1 out]
              }
              event "显控1", "显控6", "显控7", "显控2", "显控3", "显控4", "显控8", "显控9", "显控10", "显控11", "显控12", "显控5": Shortcut Menu Activation? {
                n778 = event-data() -> ("MenuRef"=w948:refnum<k9>)  [unwired: 1 in, 4 out]
                n779 = Insert Menu Items(8:string[] ["撤销关联"] ("项名称"), 9:w948) -> ()  [unwired: 4 in, 3 out]
                n780 = event-data() -> ()  [unwired: 2 in, 1 out]
              }
              event "设控1", "设控2", "设控3", "设控4", "设控5", "设控6", "设控7", "设控8": Shortcut Menu Activation? {
                n781 = event-data() -> ("MenuRef"=w950:refnum<k9>)  [unwired: 1 in, 5 out]
                n782 = event-data() -> ()  [unwired: 2 in, 1 out]
                n783 = Insert Menu Items(8:string[] ["撤销关联"] ("项名称"), 9:w950) -> ()  [unwired: 4 in, 3 out]
              }
              event "状态显示": Shortcut Menu Activation? {
                n784 = event-data() -> ("MenuRef"=w952:refnum<k9>)  [unwired: 1 in, 5 out]
                n785 = event-data() -> ()  [unwired: 2 in, 1 out]
                n786 = Insert Menu Items(8:string[] ["撤销关联"] ("项名称"), 9:w952) -> ()  [unwired: 4 in, 3 out]
              }
            }
          }
          frame #3 {
            # "所有控件撤销关联代码"
            n787 = event shown="[19] \"设控1\": 快捷菜单选择（用户）" {
              selector: _ -> [_ _ _ _ _ _ _ _ _ _ _ _ _ _ _ _ _ _ _ _ _ _ _ _ _ _ _]
              dyn-events: _ -> [_ _ _ _ _ _ _ _ _ _ _ _ _ _ _ _ _ _ _ _ _ _ _ _ _ _ _]
              timeout: 0 -> [_ _ _ _ _ _ _ _ _ _ _ _ _ _ _ _ _ _ _ _ _ _ _ _ _ _ _]
              event Timeout {
                n788 = event-data() -> ()  [unwired: 1 in, 3 out]
              }
              event "布尔 1": Shortcut Menu Selection (User) {
                w973 = T9 2 items=["刷新间隔", "波特率", "布尔1设置项", "布尔2设置项", "布尔3设置项", "布尔4设置项", "布尔5设置项", "显控1设置", "显控2设置", "显控3设置", "显控4设置", "显控5设置", "显控6设置", "显控7设置", "显控8设置", "显控9设置", "显控10设置", "显控11设置", "显控12设置", "设控1设置", "设控2设置", "设控3设置", "设控4设置", "设控5设置", "设控6设置", "设控7设置", "设控8设置", "曲线1设置", "曲线2设置", "曲线3设置", "曲线4设置", "曲线5设置", "曲线6设置", "曲线7设置", "曲线8设置", "曲线9设置", "曲线10设置", "曲线11设置", "曲线12设置", "曲线13设置", "曲线14设置", "曲线15设置", "曲线16设置", "ID值"] ("DataInitDef")
                w969 = "布尔 1" ("标题.文本")
                # "撤销关联的代码"
                n789 = event-data() -> ()  [unwired: 1 in, 8 out]
                n790 = invoke on="控件配置文件" class="Tbl (严格)" method="Set Cell Value"("X Index"=1 ("X索引"), "Y Index"=w973, "Value"="X" ("值")) -> ()  [unwired: 3 in, 6 out]
                n791 = invoke on="控件配置文件" class="Tbl (严格)" method="Set Cell Value"("X Index"=0 ("X索引"), "Y Index"=w973, "Value"=w969) -> ()  [unwired: 3 in, 6 out]
                n792 = property on="布尔 1" class="Bool (严格)"("Caption.Text"=w969) -> ()  [unwired: 2 in, 2 out]
                n793 = property on="布控1设置" class="Str"("Val(Sgnl)"=w969) -> ()  [unwired: 2 in, 2 out]
              }
              event "布尔 2": Shortcut Menu Selection (User) {
                w974 = "布尔 2" ("标题.文本")
                w978 = T9 3 items=["刷新间隔", "波特率", "布尔1设置项", "布尔2设置项", "布尔3设置项", "布尔4设置项", "布尔5设置项", "显控1设置", "显控2设置", "显控3设置", "显控4设置", "显控5设置", "显控6设置", "显控7设置", "显控8设置", "显控9设置", "显控10设置", "显控11设置", "显控12设置", "设控1设置", "设控2设置", "设控3设置", "设控4设置", "设控5设置", "设控6设置", "设控7设置", "设控8设置", "曲线1设置", "曲线2设置", "曲线3设置", "曲线4设置", "曲线5设置", "曲线6设置", "曲线7设置", "曲线8设置", "曲线9设置", "曲线10设置", "曲线11设置", "曲线12设置", "曲线13设置", "曲线14设置", "曲线15设置", "曲线16设置", "ID值"] ("DataInitDef")
                n794 = event-data() -> ()  [unwired: 1 in, 8 out]
                n795 = invoke on="控件配置文件" class="Tbl (严格)" method="Set Cell Value"("X Index"=1 ("X索引"), "Y Index"=w978, "Value"="X" ("值")) -> ()  [unwired: 3 in, 6 out]
                n796 = invoke on="控件配置文件" class="Tbl (严格)" method="Set Cell Value"("X Index"=0 ("X索引"), "Y Index"=w978, "Value"=w974) -> ()  [unwired: 3 in, 6 out]
                n797 = property on="布控2设置" class="Str"("Val(Sgnl)"=w974) -> ()  [unwired: 2 in, 2 out]
                n798 = property on="布尔 2" class="Bool (严格)"("Caption.Text"=w974) -> ()  [unwired: 2 in, 2 out]
              }
              event "布尔 3": Shortcut Menu Selection (User) {
                w983 = T9 4 items=["刷新间隔", "波特率", "布尔1设置项", "布尔2设置项", "布尔3设置项", "布尔4设置项", "布尔5设置项", "显控1设置", "显控2设置", "显控3设置", "显控4设置", "显控5设置", "显控6设置", "显控7设置", "显控8设置", "显控9设置", "显控10设置", "显控11设置", "显控12设置", "设控1设置", "设控2设置", "设控3设置", "设控4设置", "设控5设置", "设控6设置", "设控7设置", "设控8设置", "曲线1设置", "曲线2设置", "曲线3设置", "曲线4设置", "曲线5设置", "曲线6设置", "曲线7设置", "曲线8设置", "曲线9设置", "曲线10设置", "曲线11设置", "曲线12设置", "曲线13设置", "曲线14设置", "曲线15设置", "曲线16设置", "ID值"] ("DataInitDef")
                w979 = "布尔 3" ("标题.文本")
                n799 = event-data() -> ()  [unwired: 1 in, 8 out]
                n800 = invoke on="控件配置文件" class="Tbl (严格)" method="Set Cell Value"("X Index"=1 ("X索引"), "Y Index"=w983, "Value"="X" ("值")) -> ()  [unwired: 3 in, 6 out]
                n801 = invoke on="控件配置文件" class="Tbl (严格)" method="Set Cell Value"("X Index"=0 ("X索引"), "Y Index"=w983, "Value"=w979) -> ()  [unwired: 3 in, 6 out]
                n802 = property on="布尔 3" class="Bool (严格)"("Caption.Text"=w979) -> ()  [unwired: 2 in, 2 out]
                n803 = property on="布控3设置" class="Str"("Val(Sgnl)"=w979) -> ()  [unwired: 2 in, 2 out]
              }
              event "布尔 4": Shortcut Menu Selection (User) {
                w988 = T9 5 items=["刷新间隔", "波特率", "布尔1设置项", "布尔2设置项", "布尔3设置项", "布尔4设置项", "布尔5设置项", "显控1设置", "显控2设置", "显控3设置", "显控4设置", "显控5设置", "显控6设置", "显控7设置", "显控8设置", "显控9设置", "显控10设置", "显控11设置", "显控12设置", "设控1设置", "设控2设置", "设控3设置", "设控4设置", "设控5设置", "设控6设置", "设控7设置", "设控8设置", "曲线1设置", "曲线2设置", "曲线3设置", "曲线4设置", "曲线5设置", "曲线6设置", "曲线7设置", "曲线8设置", "曲线9设置", "曲线10设置", "曲线11设置", "曲线12设置", "曲线13设置", "曲线14设置", "曲线15设置", "曲线16设置", "ID值"] ("DataInitDef")
                w984 = "布尔 4" ("标题.文本")
                n804 = event-data() -> ()  [unwired: 1 in, 8 out]
                n805 = invoke on="控件配置文件" class="Tbl (严格)" method="Set Cell Value"("X Index"=1 ("X索引"), "Y Index"=w988, "Value"="X" ("值")) -> ()  [unwired: 3 in, 6 out]
                n806 = invoke on="控件配置文件" class="Tbl (严格)" method="Set Cell Value"("X Index"=0 ("X索引"), "Y Index"=w988, "Value"=w984) -> ()  [unwired: 3 in, 6 out]
                n807 = property on="布尔 4" class="Bool (严格)"("Caption.Text"=w984) -> ()  [unwired: 2 in, 2 out]
                n808 = property on="布控4设置" class="Str"("Val(Sgnl)"=w984) -> ()  [unwired: 2 in, 2 out]
              }
              event "布尔 5": Shortcut Menu Selection (User) {
                w991 = T9 6 items=["刷新间隔", "波特率", "布尔1设置项", "布尔2设置项", "布尔3设置项", "布尔4设置项", "布尔5设置项", "显控1设置", "显控2设置", "显控3设置", "显控4设置", "显控5设置", "显控6设置", "显控7设置", "显控8设置", "显控9设置", "显控10设置", "显控11设置", "显控12设置", "设控1设置", "设控2设置", "设控3设置", "设控4设置", "设控5设置", "设控6设置", "设控7设置", "设控8设置", "曲线1设置", "曲线2设置", "曲线3设置", "曲线4设置", "曲线5设置", "曲线6设置", "曲线7设置", "曲线8设置", "曲线9设置", "曲线10设置", "曲线11设置", "曲线12设置", "曲线13设置", "曲线14设置", "曲线15设置", "曲线16设置", "ID值"] ("DataInitDef")
                w993 = "布尔 5" ("标题.文本")
                n809 = event-data() -> ()  [unwired: 1 in, 8 out]
                n810 = invoke on="控件配置文件" class="Tbl (严格)" method="Set Cell Value"("X Index"=1 ("X索引"), "Y Index"=w991, "Value"="X" ("值")) -> ()  [unwired: 3 in, 6 out]
                n811 = invoke on="控件配置文件" class="Tbl (严格)" method="Set Cell Value"("X Index"=0 ("X索引"), "Y Index"=w991, "Value"=w993) -> ()  [unwired: 3 in, 6 out]
                n812 = property on="布尔 5" class="Bool (严格)"("Caption.Text"=w993) -> ()  [unwired: 2 in, 2 out]
                n813 = property on="布控5设置" class="Str"("Val(Sgnl)"=w993) -> ()  [unwired: 2 in, 2 out]
              }
              event "显控1": Shortcut Menu Selection (User) {
                w998 = T9 7 items=["刷新间隔", "波特率", "布尔1设置项", "布尔2设置项", "布尔3设置项", "布尔4设置项", "布尔5设置项", "显控1设置", "显控2设置", "显控3设置", "显控4设置", "显控5设置", "显控6设置", "显控7设置", "显控8设置", "显控9设置", "显控10设置", "显控11设置", "显控12设置", "设控1设置", "设控2设置", "设控3设置", "设控4设置", "设控5设置", "设控6设置", "设控7设置", "设控8设置", "曲线1设置", "曲线2设置", "曲线3设置", "曲线4设置", "曲线5设置", "曲线6设置", "曲线7设置", "曲线8设置", "曲线9设置", "曲线10设置", "曲线11设置", "曲线12设置", "曲线13设置", "曲线14设置", "曲线15设置", "曲线16设置", "ID值"] ("DataInitDef")
                w994 = "显控1" ("标题.文本")
                # "撤销显控关联"
                n814 = event-data() -> ()  [unwired: 1 in, 8 out]
                n815 = invoke on="控件配置文件" class="Tbl (严格)" method="Set Cell Value"("X Index"=1 ("X索引"), "Y Index"=w998, "Value"="X" ("值")) -> ()  [unwired: 3 in, 6 out]
                n816 = invoke on="控件配置文件" class="Tbl (严格)" method="Set Cell Value"("X Index"=0 ("X索引"), "Y Index"=w998, "Value"=w994) -> ()  [unwired: 3 in, 6 out]
                n817 = property on="显控1" class="Str"("Caption.Text"=w994) -> ()  [unwired: 2 in, 2 out]
                n818 = property on="显控1设置" class="Str"("Val(Sgnl)"=w994) -> ()  [unwired: 2 in, 2 out]
              }
              event "显控2": Shortcut Menu Selection (User) {
                w1003 = T9 8 items=["刷新间隔", "波特率", "布尔1设置项", "布尔2设置项", "布尔3设置项", "布尔4设置项", "布尔5设置项", "显控1设置", "显控2设置", "显控3设置", "显控4设置", "显控5设置", "显控6设置", "显控7设置", "显控8设置", "显控9设置", "显控10设置", "显控11设置", "显控12设置", "设控1设置", "设控2设置", "设控3设置", "设控4设置", "设控5设置", "设控6设置", "设控7设置", "设控8设置", "曲线1设置", "曲线2设置", "曲线3设置", "曲线4设置", "曲线5设置", "曲线6设置", "曲线7设置", "曲线8设置", "曲线9设置", "曲线10设置", "曲线11设置", "曲线12设置", "曲线13设置", "曲线14设置", "曲线15设置", "曲线16设置", "ID值"] ("DataInitDef")
                w999 = "显控2" ("标题.文本")
                n819 = event-data() -> ()  [unwired: 1 in, 8 out]
                n820 = invoke on="控件配置文件" class="Tbl (严格)" method="Set Cell Value"("X Index"=1 ("X索引"), "Y Index"=w1003, "Value"="X" ("值")) -> ()  [unwired: 3 in, 6 out]
                n821 = invoke on="控件配置文件" class="Tbl (严格)" method="Set Cell Value"("X Index"=0 ("X索引"), "Y Index"=w1003, "Value"=w999) -> ()  [unwired: 3 in, 6 out]
                n822 = property on="显控2" class="Str"("Caption.Text"=w999) -> ()  [unwired: 2 in, 2 out]
                n823 = property on="显控2设置" class="Str"("Val(Sgnl)"=w999) -> ()  [unwired: 2 in, 2 out]
              }
              event "显控3": Shortcut Menu Selection (User) {
                w1008 = T9 9 items=["刷新间隔", "波特率", "布尔1设置项", "布尔2设置项", "布尔3设置项", "布尔4设置项", "布尔5设置项", "显控1设置", "显控2设置", "显控3设置", "显控4设置", "显控5设置", "显控6设置", "显控7设置", "显控8设置", "显控9设置", "显控10设置", "显控11设置", "显控12设置", "设控1设置", "设控2设置", "设控3设置", "设控4设置", "设控5设置", "设控6设置", "设控7设置", "设控8设置", "曲线1设置", "曲线2设置", "曲线3设置", "曲线4设置", "曲线5设置", "曲线6设置", "曲线7设置", "曲线8设置", "曲线9设置", "曲线10设置", "曲线11设置", "曲线12设置", "曲线13设置", "曲线14设置", "曲线15设置", "曲线16设置", "ID值"] ("DataInitDef")
                w1004 = "显控3" ("标题.文本")
                n824 = event-data() -> ()  [unwired: 1 in, 8 out]
                n825 = invoke on="控件配置文件" class="Tbl (严格)" method="Set Cell Value"("X Index"=1 ("X索引"), "Y Index"=w1008, "Value"="X" ("值")) -> ()  [unwired: 3 in, 6 out]
                n826 = invoke on="控件配置文件" class="Tbl (严格)" method="Set Cell Value"("X Index"=0 ("X索引"), "Y Index"=w1008, "Value"=w1004) -> ()  [unwired: 3 in, 6 out]
                n827 = property on="显控3" class="Str"("Caption.Text"=w1004) -> ()  [unwired: 2 in, 2 out]
                n828 = property on="显控3设置" class="Str"("Val(Sgnl)"=w1004) -> ()  [unwired: 2 in, 2 out]
              }
              event "显控4": Shortcut Menu Selection (User) {
                w1013 = T9 10 items=["刷新间隔", "波特率", "布尔1设置项", "布尔2设置项", "布尔3设置项", "布尔4设置项", "布尔5设置项", "显控1设置", "显控2设置", "显控3设置", "显控4设置", "显控5设置", "显控6设置", "显控7设置", "显控8设置", "显控9设置", "显控10设置", "显控11设置", "显控12设置", "设控1设置", "设控2设置", "设控3设置", "设控4设置", "设控5设置", "设控6设置", "设控7设置", "设控8设置", "曲线1设置", "曲线2设置", "曲线3设置", "曲线4设置", "曲线5设置", "曲线6设置", "曲线7设置", "曲线8设置", "曲线9设置", "曲线10设置", "曲线11设置", "曲线12设置", "曲线13设置", "曲线14设置", "曲线15设置", "曲线16设置", "ID值"] ("DataInitDef")
                w1009 = "显控4" ("标题.文本")
                n829 = event-data() -> ()  [unwired: 1 in, 8 out]
                n830 = invoke on="控件配置文件" class="Tbl (严格)" method="Set Cell Value"("X Index"=1 ("X索引"), "Y Index"=w1013, "Value"="X" ("值")) -> ()  [unwired: 3 in, 6 out]
                n831 = invoke on="控件配置文件" class="Tbl (严格)" method="Set Cell Value"("X Index"=0 ("X索引"), "Y Index"=w1013, "Value"=w1009) -> ()  [unwired: 3 in, 6 out]
                n832 = property on="显控4" class="Str"("Caption.Text"=w1009) -> ()  [unwired: 2 in, 2 out]
                n833 = property on="显控4设置" class="Str"("Val(Sgnl)"=w1009) -> ()  [unwired: 2 in, 2 out]
              }
              event "显控5": Shortcut Menu Selection (User) {
                w1018 = T9 11 items=["刷新间隔", "波特率", "布尔1设置项", "布尔2设置项", "布尔3设置项", "布尔4设置项", "布尔5设置项", "显控1设置", "显控2设置", "显控3设置", "显控4设置", "显控5设置", "显控6设置", "显控7设置", "显控8设置", "显控9设置", "显控10设置", "显控11设置", "显控12设置", "设控1设置", "设控2设置", "设控3设置", "设控4设置", "设控5设置", "设控6设置", "设控7设置", "设控8设置", "曲线1设置", "曲线2设置", "曲线3设置", "曲线4设置", "曲线5设置", "曲线6设置", "曲线7设置", "曲线8设置", "曲线9设置", "曲线10设置", "曲线11设置", "曲线12设置", "曲线13设置", "曲线14设置", "曲线15设置", "曲线16设置", "ID值"] ("DataInitDef")
                w1014 = "显控5" ("标题.文本")
                n834 = event-data() -> ()  [unwired: 1 in, 8 out]
                n835 = invoke on="控件配置文件" class="Tbl (严格)" method="Set Cell Value"("X Index"=1 ("X索引"), "Y Index"=w1018, "Value"="X" ("值")) -> ()  [unwired: 3 in, 6 out]
                n836 = invoke on="控件配置文件" class="Tbl (严格)" method="Set Cell Value"("X Index"=0 ("X索引"), "Y Index"=w1018, "Value"=w1014) -> ()  [unwired: 3 in, 6 out]
                n837 = property on="显控5" class="Str"("Caption.Text"=w1014) -> ()  [unwired: 2 in, 2 out]
                n838 = property on="显控5设置" class="Str"("Val(Sgnl)"=w1014) -> ()  [unwired: 2 in, 2 out]
              }
              event "显控6": Shortcut Menu Selection (User) {
                w1023 = T9 12 items=["刷新间隔", "波特率", "布尔1设置项", "布尔2设置项", "布尔3设置项", "布尔4设置项", "布尔5设置项", "显控1设置", "显控2设置", "显控3设置", "显控4设置", "显控5设置", "显控6设置", "显控7设置", "显控8设置", "显控9设置", "显控10设置", "显控11设置", "显控12设置", "设控1设置", "设控2设置", "设控3设置", "设控4设置", "设控5设置", "设控6设置", "设控7设置", "设控8设置", "曲线1设置", "曲线2设置", "曲线3设置", "曲线4设置", "曲线5设置", "曲线6设置", "曲线7设置", "曲线8设置", "曲线9设置", "曲线10设置", "曲线11设置", "曲线12设置", "曲线13设置", "曲线14设置", "曲线15设置", "曲线16设置", "ID值"] ("DataInitDef")
                w1019 = "显控6" ("标题.文本")
                n839 = event-data() -> ()  [unwired: 1 in, 8 out]
                n840 = invoke on="控件配置文件" class="Tbl (严格)" method="Set Cell Value"("X Index"=1 ("X索引"), "Y Index"=w1023, "Value"="X" ("值")) -> ()  [unwired: 3 in, 6 out]
                n841 = invoke on="控件配置文件" class="Tbl (严格)" method="Set Cell Value"("X Index"=0 ("X索引"), "Y Index"=w1023, "Value"=w1019) -> ()  [unwired: 3 in, 6 out]
                n842 = property on="显控6" class="Str"("Caption.Text"=w1019) -> ()  [unwired: 2 in, 2 out]
                n843 = property on="显控6设置" class="Str"("Val(Sgnl)"=w1019) -> ()  [unwired: 2 in, 2 out]
              }
              event "显控7": Shortcut Menu Selection (User) {
                w1028 = T9 13 items=["刷新间隔", "波特率", "布尔1设置项", "布尔2设置项", "布尔3设置项", "布尔4设置项", "布尔5设置项", "显控1设置", "显控2设置", "显控3设置", "显控4设置", "显控5设置", "显控6设置", "显控7设置", "显控8设置", "显控9设置", "显控10设置", "显控11设置", "显控12设置", "设控1设置", "设控2设置", "设控3设置", "设控4设置", "设控5设置", "设控6设置", "设控7设置", "设控8设置", "曲线1设置", "曲线2设置", "曲线3设置", "曲线4设置", "曲线5设置", "曲线6设置", "曲线7设置", "曲线8设置", "曲线9设置", "曲线10设置", "曲线11设置", "曲线12设置", "曲线13设置", "曲线14设置", "曲线15设置", "曲线16设置", "ID值"] ("DataInitDef")
                w1024 = "显控7" ("标题.文本")
                n844 = event-data() -> ()  [unwired: 1 in, 8 out]
                n845 = invoke on="控件配置文件" class="Tbl (严格)" method="Set Cell Value"("X Index"=1 ("X索引"), "Y Index"=w1028, "Value"="X" ("值")) -> ()  [unwired: 3 in, 6 out]
                n846 = invoke on="控件配置文件" class="Tbl (严格)" method="Set Cell Value"("X Index"=0 ("X索引"), "Y Index"=w1028, "Value"=w1024) -> ()  [unwired: 3 in, 6 out]
                n847 = property on="显控7" class="Str"("Caption.Text"=w1024) -> ()  [unwired: 2 in, 2 out]
                n848 = property on="显控7设置" class="Str"("Val(Sgnl)"=w1024) -> ()  [unwired: 2 in, 2 out]
              }
              event "显控8": Shortcut Menu Selection (User) {
                w1033 = T9 14 items=["刷新间隔", "波特率", "布尔1设置项", "布尔2设置项", "布尔3设置项", "布尔4设置项", "布尔5设置项", "显控1设置", "显控2设置", "显控3设置", "显控4设置", "显控5设置", "显控6设置", "显控7设置", "显控8设置", "显控9设置", "显控10设置", "显控11设置", "显控12设置", "设控1设置", "设控2设置", "设控3设置", "设控4设置", "设控5设置", "设控6设置", "设控7设置", "设控8设置", "曲线1设置", "曲线2设置", "曲线3设置", "曲线4设置", "曲线5设置", "曲线6设置", "曲线7设置", "曲线8设置", "曲线9设置", "曲线10设置", "曲线11设置", "曲线12设置", "曲线13设置", "曲线14设置", "曲线15设置", "曲线16设置", "ID值"] ("DataInitDef")
                w1029 = "显控8" ("标题.文本")
                n849 = event-data() -> ()  [unwired: 1 in, 8 out]
                n850 = invoke on="控件配置文件" class="Tbl (严格)" method="Set Cell Value"("X Index"=1 ("X索引"), "Y Index"=w1033, "Value"="X" ("值")) -> ()  [unwired: 3 in, 6 out]
                n851 = invoke on="控件配置文件" class="Tbl (严格)" method="Set Cell Value"("X Index"=0 ("X索引"), "Y Index"=w1033, "Value"=w1029) -> ()  [unwired: 3 in, 6 out]
                n852 = property on="显控8" class="Str"("Caption.Text"=w1029) -> ()  [unwired: 2 in, 2 out]
                n853 = property on="显控8设置" class="Str"("Val(Sgnl)"=w1029) -> ()  [unwired: 2 in, 2 out]
              }
              event "显控9": Shortcut Menu Selection (User) {
                w1038 = T9 15 items=["刷新间隔", "波特率", "布尔1设置项", "布尔2设置项", "布尔3设置项", "布尔4设置项", "布尔5设置项", "显控1设置", "显控2设置", "显控3设置", "显控4设置", "显控5设置", "显控6设置", "显控7设置", "显控8设置", "显控9设置", "显控10设置", "显控11设置", "显控12设置", "设控1设置", "设控2设置", "设控3设置", "设控4设置", "设控5设置", "设控6设置", "设控7设置", "设控8设置", "曲线1设置", "曲线2设置", "曲线3设置", "曲线4设置", "曲线5设置", "曲线6设置", "曲线7设置", "曲线8设置", "曲线9设置", "曲线10设置", "曲线11设置", "曲线12设置", "曲线13设置", "曲线14设置", "曲线15设置", "曲线16设置", "ID值"] ("DataInitDef")
                w1034 = "显控9" ("标题.文本")
                n854 = event-data() -> ()  [unwired: 1 in, 8 out]
                n855 = invoke on="控件配置文件" class="Tbl (严格)" method="Set Cell Value"("X Index"=1 ("X索引"), "Y Index"=w1038, "Value"="X" ("值")) -> ()  [unwired: 3 in, 6 out]
                n856 = invoke on="控件配置文件" class="Tbl (严格)" method="Set Cell Value"("X Index"=0 ("X索引"), "Y Index"=w1038, "Value"=w1034) -> ()  [unwired: 3 in, 6 out]
                n857 = property on="显控9" class="Str"("Caption.Text"=w1034) -> ()  [unwired: 2 in, 2 out]
                n858 = property on="显控9设置" class="Str"("Val(Sgnl)"=w1034) -> ()  [unwired: 2 in, 2 out]
              }
              event "显控10": Shortcut Menu Selection (User) {
                w1043 = T9 16 items=["刷新间隔", "波特率", "布尔1设置项", "布尔2设置项", "布尔3设置项", "布尔4设置项", "布尔5设置项", "显控1设置", "显控2设置", "显控3设置", "显控4设置", "显控5设置", "显控6设置", "显控7设置", "显控8设置", "显控9设置", "显控10设置", "显控11设置", "显控12设置", "设控1设置", "设控2设置", "设控3设置", "设控4设置", "设控5设置", "设控6设置", "设控7设置", "设控8设置", "曲线1设置", "曲线2设置", "曲线3设置", "曲线4设置", "曲线5设置", "曲线6设置", "曲线7设置", "曲线8设置", "曲线9设置", "曲线10设置", "曲线11设置", "曲线12设置", "曲线13设置", "曲线14设置", "曲线15设置", "曲线16设置", "ID值"] ("DataInitDef")
                w1039 = "显控10" ("标题.文本")
                n859 = event-data() -> ()  [unwired: 1 in, 8 out]
                n860 = invoke on="控件配置文件" class="Tbl (严格)" method="Set Cell Value"("X Index"=1 ("X索引"), "Y Index"=w1043, "Value"="X" ("值")) -> ()  [unwired: 3 in, 6 out]
                n861 = invoke on="控件配置文件" class="Tbl (严格)" method="Set Cell Value"("X Index"=0 ("X索引"), "Y Index"=w1043, "Value"=w1039) -> ()  [unwired: 3 in, 6 out]
                n862 = property on="显控10" class="Str"("Caption.Text"=w1039) -> ()  [unwired: 2 in, 2 out]
                n863 = property on="显控10设置" class="Str"("Val(Sgnl)"=w1039) -> ()  [unwired: 2 in, 2 out]
              }
              event "显控11": Shortcut Menu Selection (User) {
                w1048 = T9 17 items=["刷新间隔", "波特率", "布尔1设置项", "布尔2设置项", "布尔3设置项", "布尔4设置项", "布尔5设置项", "显控1设置", "显控2设置", "显控3设置", "显控4设置", "显控5设置", "显控6设置", "显控7设置", "显控8设置", "显控9设置", "显控10设置", "显控11设置", "显控12设置", "设控1设置", "设控2设置", "设控3设置", "设控4设置", "设控5设置", "设控6设置", "设控7设置", "设控8设置", "曲线1设置", "曲线2设置", "曲线3设置", "曲线4设置", "曲线5设置", "曲线6设置", "曲线7设置", "曲线8设置", "曲线9设置", "曲线10设置", "曲线11设置", "曲线12设置", "曲线13设置", "曲线14设置", "曲线15设置", "曲线16设置", "ID值"] ("DataInitDef")
                w1044 = "显控11" ("标题.文本")
                n864 = event-data() -> ()  [unwired: 1 in, 8 out]
                n865 = invoke on="控件配置文件" class="Tbl (严格)" method="Set Cell Value"("X Index"=1 ("X索引"), "Y Index"=w1048, "Value"="X" ("值")) -> ()  [unwired: 3 in, 6 out]
                n866 = invoke on="控件配置文件" class="Tbl (严格)" method="Set Cell Value"("X Index"=0 ("X索引"), "Y Index"=w1048, "Value"=w1044) -> ()  [unwired: 3 in, 6 out]
                n867 = property on="显控11" class="Str"("Caption.Text"=w1044) -> ()  [unwired: 2 in, 2 out]
                n868 = property on="显控11设置" class="Str"("Val(Sgnl)"=w1044) -> ()  [unwired: 2 in, 2 out]
              }
              event "显控12": Shortcut Menu Selection (User) {
                w1053 = T9 18 items=["刷新间隔", "波特率", "布尔1设置项", "布尔2设置项", "布尔3设置项", "布尔4设置项", "布尔5设置项", "显控1设置", "显控2设置", "显控3设置", "显控4设置", "显控5设置", "显控6设置", "显控7设置", "显控8设置", "显控9设置", "显控10设置", "显控11设置", "显控12设置", "设控1设置", "设控2设置", "设控3设置", "设控4设置", "设控5设置", "设控6设置", "设控7设置", "设控8设置", "曲线1设置", "曲线2设置", "曲线3设置", "曲线4设置", "曲线5设置", "曲线6设置", "曲线7设置", "曲线8设置", "曲线9设置", "曲线10设置", "曲线11设置", "曲线12设置", "曲线13设置", "曲线14设置", "曲线15设置", "曲线16设置", "ID值"] ("DataInitDef")
                w1049 = "显控12" ("标题.文本")
                n869 = event-data() -> ()  [unwired: 1 in, 8 out]
                n870 = invoke on="控件配置文件" class="Tbl (严格)" method="Set Cell Value"("X Index"=1 ("X索引"), "Y Index"=w1053, "Value"="X" ("值")) -> ()  [unwired: 3 in, 6 out]
                n871 = invoke on="控件配置文件" class="Tbl (严格)" method="Set Cell Value"("X Index"=0 ("X索引"), "Y Index"=w1053, "Value"=w1049) -> ()  [unwired: 3 in, 6 out]
                n872 = property on="显控12" class="Str"("Caption.Text"=w1049) -> ()  [unwired: 2 in, 2 out]
                n873 = property on="显控12设置" class="Str"("Val(Sgnl)"=w1049) -> ()  [unwired: 2 in, 2 out]
              }
              event "波形图表": Shortcut Menu Selection (User) {
                n874 = event-data() -> ("ItemTag"=w1054:string)  [unwired: 1 in]
                n875 = case shown="\"删除曲线8\"" w1054 {
                  frame "删除曲线1" {
                    w1055 = "曲线1" ("值")
                    w1056 = T9 27 items=["刷新间隔", "波特率", "布尔1设置项", "布尔2设置项", "布尔3设置项", "布尔4设置项", "布尔5设置项", "显控1设置", "显控2设置", "显控3设置", "显控4设置", "显控5设置", "显控6设置", "显控7设置", "显控8设置", "显控9设置", "显控10设置", "显控11设置", "显控12设置", "设控1设置", "设控2设置", "设控3设置", "设控4设置", "设控5设置", "设控6设置", "设控7设置", "设控8设置", "曲线1设置", "曲线2设置", "曲线3设置", "曲线4设置", "曲线5设置", "曲线6设置", "曲线7设置", "曲线8设置", "曲线9设置", "曲线10设置", "曲线11设置", "曲线12设置", "曲线13设置", "曲线14设置", "曲线15设置", "曲线16设置", "ID值"] ("DataInitDef")
                    n876 = invoke on="控件配置文件" class="Tbl (严格)" method="Set Cell Value"("X Index"=1 ("X索引"), "Y Index"=w1056, "Value"="X" ("值")) -> ()  [unwired: 3 in, 6 out]
                    n877 = invoke on="控件配置文件" class="Tbl (严格)" method="Set Cell Value"("X Index"=0 ("X索引"), "Y Index"=w1056, "Value"=w1055) -> ()  [unwired: 3 in, 6 out]
                    n878 = property on="曲线1设置" class="Str"("Val(Sgnl)"=w1055) -> ()  [unwired: 2 in, 2 out]
                  }
                  frame "假", Default {
                  }
                  frame "删除曲线2" {
                    w1060 = "曲线2" ("值")
                    w1061 = T9 28 items=["刷新间隔", "波特率", "布尔1设置项", "布尔2设置项", "布尔3设置项", "布尔4设置项", "布尔5设置项", "显控1设置", "显控2设置", "显控3设置", "显控4设置", "显控5设置", "显控6设置", "显控7设置", "显控8设置", "显控9设置", "显控10设置", "显控11设置", "显控12设置", "设控1设置", "设控2设置", "设控3设置", "设控4设置", "设控5设置", "设控6设置", "设控7设置", "设控8设置", "曲线1设置", "曲线2设置", "曲线3设置", "曲线4设置", "曲线5设置", "曲线6设置", "曲线7设置", "曲线8设置", "曲线9设置", "曲线10设置", "曲线11设置", "曲线12设置", "曲线13设置", "曲线14设置", "曲线15设置", "曲线16设置", "ID值"] ("DataInitDef")
                    n879 = invoke on="控件配置文件" class="Tbl (严格)" method="Set Cell Value"("X Index"=1 ("X索引"), "Y Index"=w1061, "Value"="X" ("值")) -> ()  [unwired: 3 in, 6 out]
                    n880 = invoke on="控件配置文件" class="Tbl (严格)" method="Set Cell Value"("X Index"=0 ("X索引"), "Y Index"=w1061, "Value"=w1060) -> ()  [unwired: 3 in, 6 out]
                    n881 = property on="曲线2设置" class="Str"("Val(Sgnl)"=w1060) -> ()  [unwired: 2 in, 2 out]
                  }
                  frame "删除曲线3" {
                    w1065 = "曲线3" ("值")
                    w1066 = T9 29 items=["刷新间隔", "波特率", "布尔1设置项", "布尔2设置项", "布尔3设置项", "布尔4设置项", "布尔5设置项", "显控1设置", "显控2设置", "显控3设置", "显控4设置", "显控5设置", "显控6设置", "显控7设置", "显控8设置", "显控9设置", "显控10设置", "显控11设置", "显控12设置", "设控1设置", "设控2设置", "设控3设置", "设控4设置", "设控5设置", "设控6设置", "设控7设置", "设控8设置", "曲线1设置", "曲线2设置", "曲线3设置", "曲线4设置", "曲线5设置", "曲线6设置", "曲线7设置", "曲线8设置", "曲线9设置", "曲线10设置", "曲线11设置", "曲线12设置", "曲线13设置", "曲线14设置", "曲线15设置", "曲线16设置", "ID值"] ("DataInitDef")
                    n882 = invoke on="控件配置文件" class="Tbl (严格)" method="Set Cell Value"("X Index"=1 ("X索引"), "Y Index"=w1066, "Value"="X" ("值")) -> ()  [unwired: 3 in, 6 out]
                    n883 = invoke on="控件配置文件" class="Tbl (严格)" method="Set Cell Value"("X Index"=0 ("X索引"), "Y Index"=w1066, "Value"=w1065) -> ()  [unwired: 3 in, 6 out]
                    n884 = property on="曲线3设置" class="Str"("Val(Sgnl)"=w1065) -> ()  [unwired: 2 in, 2 out]
                  }
                  frame "删除曲线4" {
                    w1070 = "曲线4" ("值")
                    w1071 = T9 30 items=["刷新间隔", "波特率", "布尔1设置项", "布尔2设置项", "布尔3设置项", "布尔4设置项", "布尔5设置项", "显控1设置", "显控2设置", "显控3设置", "显控4设置", "显控5设置", "显控6设置", "显控7设置", "显控8设置", "显控9设置", "显控10设置", "显控11设置", "显控12设置", "设控1设置", "设控2设置", "设控3设置", "设控4设置", "设控5设置", "设控6设置", "设控7设置", "设控8设置", "曲线1设置", "曲线2设置", "曲线3设置", "曲线4设置", "曲线5设置", "曲线6设置", "曲线7设置", "曲线8设置", "曲线9设置", "曲线10设置", "曲线11设置", "曲线12设置", "曲线13设置", "曲线14设置", "曲线15设置", "曲线16设置", "ID值"] ("DataInitDef")
                    n885 = invoke on="控件配置文件" class="Tbl (严格)" method="Set Cell Value"("X Index"=1 ("X索引"), "Y Index"=w1071, "Value"="X" ("值")) -> ()  [unwired: 3 in, 6 out]
                    n886 = invoke on="控件配置文件" class="Tbl (严格)" method="Set Cell Value"("X Index"=0 ("X索引"), "Y Index"=w1071, "Value"=w1070) -> ()  [unwired: 3 in, 6 out]
                    n887 = property on="曲线4设置" class="Str"("Val(Sgnl)"=w1070) -> ()  [unwired: 2 in, 2 out]
                  }
                  frame "删除曲线5" {
                    w1075 = "曲线5" ("值")
                    w1076 = T9 31 items=["刷新间隔", "波特率", "布尔1设置项", "布尔2设置项", "布尔3设置项", "布尔4设置项", "布尔5设置项", "显控1设置", "显控2设置", "显控3设置", "显控4设置", "显控5设置", "显控6设置", "显控7设置", "显控8设置", "显控9设置", "显控10设置", "显控11设置", "显控12设置", "设控1设置", "设控2设置", "设控3设置", "设控4设置", "设控5设置", "设控6设置", "设控7设置", "设控8设置", "曲线1设置", "曲线2设置", "曲线3设置", "曲线4设置", "曲线5设置", "曲线6设置", "曲线7设置", "曲线8设置", "曲线9设置", "曲线10设置", "曲线11设置", "曲线12设置", "曲线13设置", "曲线14设置", "曲线15设置", "曲线16设置", "ID值"] ("DataInitDef")
                    n888 = invoke on="控件配置文件" class="Tbl (严格)" method="Set Cell Value"("X Index"=1 ("X索引"), "Y Index"=w1076, "Value"="X" ("值")) -> ()  [unwired: 3 in, 6 out]
                    n889 = invoke on="控件配置文件" class="Tbl (严格)" method="Set Cell Value"("X Index"=0 ("X索引"), "Y Index"=w1076, "Value"=w1075) -> ()  [unwired: 3 in, 6 out]
                    n890 = property on="曲线5设置" class="Str"("Val(Sgnl)"=w1075) -> ()  [unwired: 2 in, 2 out]
                  }
                  frame "删除曲线6" {
                    w1080 = "曲线6" ("值")
                    w1081 = T9 32 items=["刷新间隔", "波特率", "布尔1设置项", "布尔2设置项", "布尔3设置项", "布尔4设置项", "布尔5设置项", "显控1设置", "显控2设置", "显控3设置", "显控4设置", "显控5设置", "显控6设置", "显控7设置", "显控8设置", "显控9设置", "显控10设置", "显控11设置", "显控12设置", "设控1设置", "设控2设置", "设控3设置", "设控4设置", "设控5设置", "设控6设置", "设控7设置", "设控8设置", "曲线1设置", "曲线2设置", "曲线3设置", "曲线4设置", "曲线5设置", "曲线6设置", "曲线7设置", "曲线8设置", "曲线9设置", "曲线10设置", "曲线11设置", "曲线12设置", "曲线13设置", "曲线14设置", "曲线15设置", "曲线16设置", "ID值"] ("DataInitDef")
                    n891 = invoke on="控件配置文件" class="Tbl (严格)" method="Set Cell Value"("X Index"=1 ("X索引"), "Y Index"=w1081, "Value"="X" ("值")) -> ()  [unwired: 3 in, 6 out]
                    n892 = invoke on="控件配置文件" class="Tbl (严格)" method="Set Cell Value"("X Index"=0 ("X索引"), "Y Index"=w1081, "Value"=w1080) -> ()  [unwired: 3 in, 6 out]
                    n893 = property on="曲线6设置" class="Str"("Val(Sgnl)"=w1080) -> ()  [unwired: 2 in, 2 out]
                  }
                  frame "清除图表" {
                    n894 = property on="波形图表" class="WFChart (严格)"("History Data"=dynamicdata[] [] ("历史数据")) -> ()  [unwired: 2 in, 2 out]
                  }
                  frame "删除曲线7" {
                    w1086 = "曲线7" ("值")
                    w1087 = T9 33 items=["刷新间隔", "波特率", "布尔1设置项", "布尔2设置项", "布尔3设置项", "布尔4设置项", "布尔5设置项", "显控1设置", "显控2设置", "显控3设置", "显控4设置", "显控5设置", "显控6设置", "显控7设置", "显控8设置", "显控9设置", "显控10设置", "显控11设置", "显控12设置", "设控1设置", "设控2设置", "设控3设置", "设控4设置", "设控5设置", "设控6设置", "设控7设置", "设控8设置", "曲线1设置", "曲线2设置", "曲线3设置", "曲线4设置", "曲线5设置", "曲线6设置", "曲线7设置", "曲线8设置", "曲线9设置", "曲线10设置", "曲线11设置", "曲线12设置", "曲线13设置", "曲线14设置", "曲线15设置", "曲线16设置", "ID值"] ("DataInitDef")
                    n895 = invoke on="控件配置文件" class="Tbl (严格)" method="Set Cell Value"("X Index"=1 ("X索引"), "Y Index"=w1087, "Value"="X" ("值")) -> ()  [unwired: 3 in, 6 out]
                    n896 = invoke on="控件配置文件" class="Tbl (严格)" method="Set Cell Value"("X Index"=0 ("X索引"), "Y Index"=w1087, "Value"=w1086) -> ()  [unwired: 3 in, 6 out]
                    n897 = property on="曲线7设置" class="Str"("Val(Sgnl)"=w1086) -> ()  [unwired: 2 in, 2 out]
                  }
                  frame "删除所有曲线" {
                    n898 = stacked-sequence {
                      frame #0 {
                        w1091 = "曲线1" ("值")
                        w1092 = T9 27 items=["刷新间隔", "波特率", "布尔1设置项", "布尔2设置项", "布尔3设置项", "布尔4设置项", "布尔5设置项", "显控1设置", "显控2设置", "显控3设置", "显控4设置", "显控5设置", "显控6设置", "显控7设置", "显控8设置", "显控9设置", "显控10设置", "显控11设置", "显控12设置", "设控1设置", "设控2设置", "设控3设置", "设控4设置", "设控5设置", "设控6设置", "设控7设置", "设控8设置", "曲线1设置", "曲线2设置", "曲线3设置", "曲线4设置", "曲线5设置", "曲线6设置", "曲线7设置", "曲线8设置", "曲线9设置", "曲线10设置", "曲线11设置", "曲线12设置", "曲线13设置", "曲线14设置", "曲线15设置", "曲线16设置", "ID值"] ("DataInitDef")
                        n899 = invoke on="控件配置文件" class="Tbl (严格)" method="Set Cell Value"("X Index"=1 ("X索引"), "Y Index"=w1092, "Value"="X" ("值")) -> ()  [unwired: 3 in, 6 out]
                        n900 = invoke on="控件配置文件" class="Tbl (严格)" method="Set Cell Value"("X Index"=0 ("X索引"), "Y Index"=w1092, "Value"=w1091) -> ()  [unwired: 3 in, 6 out]
                        n901 = property on="曲线1设置" class="Str"("Val(Sgnl)"=w1091) -> ()  [unwired: 2 in, 2 out]
                      }
                      frame #1 {
                        w1096 = "曲线2" ("值")
                        w1097 = T9 28 items=["刷新间隔", "波特率", "布尔1设置项", "布尔2设置项", "布尔3设置项", "布尔4设置项", "布尔5设置项", "显控1设置", "显控2设置", "显控3设置", "显控4设置", "显控5设置", "显控6设置", "显控7设置", "显控8设置", "显控9设置", "显控10设置", "显控11设置", "显控12设置", "设控1设置", "设控2设置", "设控3设置", "设控4设置", "设控5设置", "设控6设置", "设控7设置", "设控8设置", "曲线1设置", "曲线2设置", "曲线3设置", "曲线4设置", "曲线5设置", "曲线6设置", "曲线7设置", "曲线8设置", "曲线9设置", "曲线10设置", "曲线11设置", "曲线12设置", "曲线13设置", "曲线14设置", "曲线15设置", "曲线16设置", "ID值"] ("DataInitDef")
                        n902 = invoke on="控件配置文件" class="Tbl (严格)" method="Set Cell Value"("X Index"=1 ("X索引"), "Y Index"=w1097, "Value"="X" ("值")) -> ()  [unwired: 3 in, 6 out]
                        n903 = invoke on="控件配置文件" class="Tbl (严格)" method="Set Cell Value"("X Index"=0 ("X索引"), "Y Index"=w1097, "Value"=w1096) -> ()  [unwired: 3 in, 6 out]
                        n904 = property on="曲线2设置" class="Str"("Val(Sgnl)"=w1096) -> ()  [unwired: 2 in, 2 out]
                      }
                      frame #2 {
                        w1101 = "曲线3" ("值")
                        w1102 = T9 29 items=["刷新间隔", "波特率", "布尔1设置项", "布尔2设置项", "布尔3设置项", "布尔4设置项", "布尔5设置项", "显控1设置", "显控2设置", "显控3设置", "显控4设置", "显控5设置", "显控6设置", "显控7设置", "显控8设置", "显控9设置", "显控10设置", "显控11设置", "显控12设置", "设控1设置", "设控2设置", "设控3设置", "设控4设置", "设控5设置", "设控6设置", "设控7设置", "设控8设置", "曲线1设置", "曲线2设置", "曲线3设置", "曲线4设置", "曲线5设置", "曲线6设置", "曲线7设置", "曲线8设置", "曲线9设置", "曲线10设置", "曲线11设置", "曲线12设置", "曲线13设置", "曲线14设置", "曲线15设置", "曲线16设置", "ID值"] ("DataInitDef")
                        n905 = invoke on="控件配置文件" class="Tbl (严格)" method="Set Cell Value"("X Index"=1 ("X索引"), "Y Index"=w1102, "Value"="X" ("值")) -> ()  [unwired: 3 in, 6 out]
                        n906 = invoke on="控件配置文件" class="Tbl (严格)" method="Set Cell Value"("X Index"=0 ("X索引"), "Y Index"=w1102, "Value"=w1101) -> ()  [unwired: 3 in, 6 out]
                        n907 = property on="曲线3设置" class="Str"("Val(Sgnl)"=w1101) -> ()  [unwired: 2 in, 2 out]
                      }
                      frame #3 {
                        w1106 = "曲线4" ("值")
                        w1107 = T9 30 items=["刷新间隔", "波特率", "布尔1设置项", "布尔2设置项", "布尔3设置项", "布尔4设置项", "布尔5设置项", "显控1设置", "显控2设置", "显控3设置", "显控4设置", "显控5设置", "显控6设置", "显控7设置", "显控8设置", "显控9设置", "显控10设置", "显控11设置", "显控12设置", "设控1设置", "设控2设置", "设控3设置", "设控4设置", "设控5设置", "设控6设置", "设控7设置", "设控8设置", "曲线1设置", "曲线2设置", "曲线3设置", "曲线4设置", "曲线5设置", "曲线6设置", "曲线7设置", "曲线8设置", "曲线9设置", "曲线10设置", "曲线11设置", "曲线12设置", "曲线13设置", "曲线14设置", "曲线15设置", "曲线16设置", "ID值"] ("DataInitDef")
                        n908 = invoke on="控件配置文件" class="Tbl (严格)" method="Set Cell Value"("X Index"=1 ("X索引"), "Y Index"=w1107, "Value"="X" ("值")) -> ()  [unwired: 3 in, 6 out]
                        n909 = invoke on="控件配置文件" class="Tbl (严格)" method="Set Cell Value"("X Index"=0 ("X索引"), "Y Index"=w1107, "Value"=w1106) -> ()  [unwired: 3 in, 6 out]
                        n910 = property on="曲线4设置" class="Str"("Val(Sgnl)"=w1106) -> ()  [unwired: 2 in, 2 out]
                      }
                      frame #4 {
                        w1111 = "曲线5" ("值")
                        w1112 = T9 31 items=["刷新间隔", "波特率", "布尔1设置项", "布尔2设置项", "布尔3设置项", "布尔4设置项", "布尔5设置项", "显控1设置", "显控2设置", "显控3设置", "显控4设置", "显控5设置", "显控6设置", "显控7设置", "显控8设置", "显控9设置", "显控10设置", "显控11设置", "显控12设置", "设控1设置", "设控2设置", "设控3设置", "设控4设置", "设控5设置", "设控6设置", "设控7设置", "设控8设置", "曲线1设置", "曲线2设置", "曲线3设置", "曲线4设置", "曲线5设置", "曲线6设置", "曲线7设置", "曲线8设置", "曲线9设置", "曲线10设置", "曲线11设置", "曲线12设置", "曲线13设置", "曲线14设置", "曲线15设置", "曲线16设置", "ID值"] ("DataInitDef")
                        n911 = invoke on="控件配置文件" class="Tbl (严格)" method="Set Cell Value"("X Index"=1 ("X索引"), "Y Index"=w1112, "Value"="X" ("值")) -> ()  [unwired: 3 in, 6 out]
                        n912 = invoke on="控件配置文件" class="Tbl (严格)" method="Set Cell Value"("X Index"=0 ("X索引"), "Y Index"=w1112, "Value"=w1111) -> ()  [unwired: 3 in, 6 out]
                        n913 = property on="曲线5设置" class="Str"("Val(Sgnl)"=w1111) -> ()  [unwired: 2 in, 2 out]
                      }
                      frame #5 {
                        w1116 = "曲线6" ("值")
                        w1117 = T9 32 items=["刷新间隔", "波特率", "布尔1设置项", "布尔2设置项", "布尔3设置项", "布尔4设置项", "布尔5设置项", "显控1设置", "显控2设置", "显控3设置", "显控4设置", "显控5设置", "显控6设置", "显控7设置", "显控8设置", "显控9设置", "显控10设置", "显控11设置", "显控12设置", "设控1设置", "设控2设置", "设控3设置", "设控4设置", "设控5设置", "设控6设置", "设控7设置", "设控8设置", "曲线1设置", "曲线2设置", "曲线3设置", "曲线4设置", "曲线5设置", "曲线6设置", "曲线7设置", "曲线8设置", "曲线9设置", "曲线10设置", "曲线11设置", "曲线12设置", "曲线13设置", "曲线14设置", "曲线15设置", "曲线16设置", "ID值"] ("DataInitDef")
                        n914 = invoke on="控件配置文件" class="Tbl (严格)" method="Set Cell Value"("X Index"=1 ("X索引"), "Y Index"=w1117, "Value"="X" ("值")) -> ()  [unwired: 3 in, 6 out]
                        n915 = invoke on="控件配置文件" class="Tbl (严格)" method="Set Cell Value"("X Index"=0 ("X索引"), "Y Index"=w1117, "Value"=w1116) -> ()  [unwired: 3 in, 6 out]
                        n916 = property on="曲线6设置" class="Str"("Val(Sgnl)"=w1116) -> ()  [unwired: 2 in, 2 out]
                      }
                      frame #6 {
                        w1121 = "曲线7" ("值")
                        w1122 = T9 33 items=["刷新间隔", "波特率", "布尔1设置项", "布尔2设置项", "布尔3设置项", "布尔4设置项", "布尔5设置项", "显控1设置", "显控2设置", "显控3设置", "显控4设置", "显控5设置", "显控6设置", "显控7设置", "显控8设置", "显控9设置", "显控10设置", "显控11设置", "显控12设置", "设控1设置", "设控2设置", "设控3设置", "设控4设置", "设控5设置", "设控6设置", "设控7设置", "设控8设置", "曲线1设置", "曲线2设置", "曲线3设置", "曲线4设置", "曲线5设置", "曲线6设置", "曲线7设置", "曲线8设置", "曲线9设置", "曲线10设置", "曲线11设置", "曲线12设置", "曲线13设置", "曲线14设置", "曲线15设置", "曲线16设置", "ID值"] ("DataInitDef")
                        n917 = invoke on="控件配置文件" class="Tbl (严格)" method="Set Cell Value"("X Index"=1 ("X索引"), "Y Index"=w1122, "Value"="X" ("值")) -> ()  [unwired: 3 in, 6 out]
                        n918 = invoke on="控件配置文件" class="Tbl (严格)" method="Set Cell Value"("X Index"=0 ("X索引"), "Y Index"=w1122, "Value"=w1121) -> ()  [unwired: 3 in, 6 out]
                        n919 = property on="曲线7设置" class="Str"("Val(Sgnl)"=w1121) -> ()  [unwired: 2 in, 2 out]
                      }
                      frame #7 {
                        w1130 = "曲线8" ("值")
                        w1128 = T9 34 items=["刷新间隔", "波特率", "布尔1设置项", "布尔2设置项", "布尔3设置项", "布尔4设置项", "布尔5设置项", "显控1设置", "显控2设置", "显控3设置", "显控4设置", "显控5设置", "显控6设置", "显控7设置", "显控8设置", "显控9设置", "显控10设置", "显控11设置", "显控12设置", "设控1设置", "设控2设置", "设控3设置", "设控4设置", "设控5设置", "设控6设置", "设控7设置", "设控8设置", "曲线1设置", "曲线2设置", "曲线3设置", "曲线4设置", "曲线5设置", "曲线6设置", "曲线7设置", "曲线8设置", "曲线9设置", "曲线10设置", "曲线11设置", "曲线12设置", "曲线13设置", "曲线14设置", "曲线15设置", "曲线16设置", "ID值"] ("DataInitDef")
                        n920 = invoke on="控件配置文件" class="Tbl (严格)" method="Set Cell Value"("X Index"=1 ("X索引"), "Y Index"=w1128, "Value"="X" ("值")) -> ()  [unwired: 3 in, 6 out]
                        n921 = invoke on="控件配置文件" class="Tbl (严格)" method="Set Cell Value"("X Index"=0 ("X索引"), "Y Index"=w1128, "Value"=w1130) -> ()  [unwired: 3 in, 6 out]
                        n922 = property on="曲线8设置" class="Str"("Val(Sgnl)"=w1130) -> ()  [unwired: 2 in, 2 out]
                      }
                      frame #8 {
                        w1131 = T9 35 items=["刷新间隔", "波特率", "布尔1设置项", "布尔2设置项", "布尔3设置项", "布尔4设置项", "布尔5设置项", "显控1设置", "显控2设置", "显控3设置", "显控4设置", "显控5设置", "显控6设置", "显控7设置", "显控8设置", "显控9设置", "显控10设置", "显控11设置", "显控12设置", "设控1设置", "设控2设置", "设控3设置", "设控4设置", "设控5设置", "设控6设置", "设控7设置", "设控8设置", "曲线1设置", "曲线2设置", "曲线3设置", "曲线4设置", "曲线5设置", "曲线6设置", "曲线7设置", "曲线8设置", "曲线9设置", "曲线10设置", "曲线11设置", "曲线12设置", "曲线13设置", "曲线14设置", "曲线15设置", "曲线16设置", "ID值"] ("DataInitDef")
                        w1135 = "曲线9" ("值")
                        n923 = invoke on="控件配置文件" class="Tbl (严格)" method="Set Cell Value"("X Index"=1 ("X索引"), "Y Index"=w1131, "Value"="X" ("值")) -> ()  [unwired: 3 in, 6 out]
                        n924 = invoke on="控件配置文件" class="Tbl (严格)" method="Set Cell Value"("X Index"=0 ("X索引"), "Y Index"=w1131, "Value"=w1135) -> ()  [unwired: 3 in, 6 out]
                        n925 = property on="曲线9设置" class="Str"("Val(Sgnl)"=w1135) -> ()  [unwired: 2 in, 2 out]
                      }
                      frame #9 {
                        w1140 = T9 36 items=["刷新间隔", "波特率", "布尔1设置项", "布尔2设置项", "布尔3设置项", "布尔4设置项", "布尔5设置项", "显控1设置", "显控2设置", "显控3设置", "显控4设置", "显控5设置", "显控6设置", "显控7设置", "显控8设置", "显控9设置", "显控10设置", "显控11设置", "显控12设置", "设控1设置", "设控2设置", "设控3设置", "设控4设置", "设控5设置", "设控6设置", "设控7设置", "设控8设置", "曲线1设置", "曲线2设置", "曲线3设置", "曲线4设置", "曲线5设置", "曲线6设置", "曲线7设置", "曲线8设置", "曲线9设置", "曲线10设置", "曲线11设置", "曲线12设置", "曲线13设置", "曲线14设置", "曲线15设置", "曲线16设置", "ID值"] ("DataInitDef")
                        w1139 = "曲线10" ("值")
                        n926 = invoke on="控件配置文件" class="Tbl (严格)" method="Set Cell Value"("X Index"=1 ("X索引"), "Y Index"=w1140, "Value"="X" ("值")) -> ()  [unwired: 3 in, 6 out]
                        n927 = invoke on="控件配置文件" class="Tbl (严格)" method="Set Cell Value"("X Index"=0 ("X索引"), "Y Index"=w1140, "Value"=w1139) -> ()  [unwired: 3 in, 6 out]
                        n928 = property on="曲线10设置" class="Str"("Val(Sgnl)"=w1139) -> ()  [unwired: 2 in, 2 out]
                      }
                      frame #10 {
                        w1145 = T9 37 items=["刷新间隔", "波特率", "布尔1设置项", "布尔2设置项", "布尔3设置项", "布尔4设置项", "布尔5设置项", "显控1设置", "显控2设置", "显控3设置", "显控4设置", "显控5设置", "显控6设置", "显控7设置", "显控8设置", "显控9设置", "显控10设置", "显控11设置", "显控12设置", "设控1设置", "设控2设置", "设控3设置", "设控4设置", "设控5设置", "设控6设置", "设控7设置", "设控8设置", "曲线1设置", "曲线2设置", "曲线3设置", "曲线4设置", "曲线5设置", "曲线6设置", "曲线7设置", "曲线8设置", "曲线9设置", "曲线10设置", "曲线11设置", "曲线12设置", "曲线13设置", "曲线14设置", "曲线15设置", "曲线16设置", "ID值"] ("DataInitDef")
                        w1144 = "曲线11" ("值")
                        n929 = invoke on="控件配置文件" class="Tbl (严格)" method="Set Cell Value"("X Index"=1 ("X索引"), "Y Index"=w1145, "Value"="X" ("值")) -> ()  [unwired: 3 in, 6 out]
                        n930 = invoke on="控件配置文件" class="Tbl (严格)" method="Set Cell Value"("X Index"=0 ("X索引"), "Y Index"=w1145, "Value"=w1144) -> ()  [unwired: 3 in, 6 out]
                        n931 = property on="曲线11设置" class="Str"("Val(Sgnl)"=w1144) -> ()  [unwired: 2 in, 2 out]
                      }
                      frame #11 {
                        w1150 = T9 38 items=["刷新间隔", "波特率", "布尔1设置项", "布尔2设置项", "布尔3设置项", "布尔4设置项", "布尔5设置项", "显控1设置", "显控2设置", "显控3设置", "显控4设置", "显控5设置", "显控6设置", "显控7设置", "显控8设置", "显控9设置", "显控10设置", "显控11设置", "显控12设置", "设控1设置", "设控2设置", "设控3设置", "设控4设置", "设控5设置", "设控6设置", "设控7设置", "设控8设置", "曲线1设置", "曲线2设置", "曲线3设置", "曲线4设置", "曲线5设置", "曲线6设置", "曲线7设置", "曲线8设置", "曲线9设置", "曲线10设置", "曲线11设置", "曲线12设置", "曲线13设置", "曲线14设置", "曲线15设置", "曲线16设置", "ID值"] ("DataInitDef")
                        w1149 = "曲线12" ("值")
                        n932 = invoke on="控件配置文件" class="Tbl (严格)" method="Set Cell Value"("X Index"=1 ("X索引"), "Y Index"=w1150, "Value"="X" ("值")) -> ()  [unwired: 3 in, 6 out]
                        n933 = invoke on="控件配置文件" class="Tbl (严格)" method="Set Cell Value"("X Index"=0 ("X索引"), "Y Index"=w1150, "Value"=w1149) -> ()  [unwired: 3 in, 6 out]
                        n934 = property on="曲线12设置" class="Str"("Val(Sgnl)"=w1149) -> ()  [unwired: 2 in, 2 out]
                      }
                      frame #12 {
                        w1155 = T9 39 items=["刷新间隔", "波特率", "布尔1设置项", "布尔2设置项", "布尔3设置项", "布尔4设置项", "布尔5设置项", "显控1设置", "显控2设置", "显控3设置", "显控4设置", "显控5设置", "显控6设置", "显控7设置", "显控8设置", "显控9设置", "显控10设置", "显控11设置", "显控12设置", "设控1设置", "设控2设置", "设控3设置", "设控4设置", "设控5设置", "设控6设置", "设控7设置", "设控8设置", "曲线1设置", "曲线2设置", "曲线3设置", "曲线4设置", "曲线5设置", "曲线6设置", "曲线7设置", "曲线8设置", "曲线9设置", "曲线10设置", "曲线11设置", "曲线12设置", "曲线13设置", "曲线14设置", "曲线15设置", "曲线16设置", "ID值"] ("DataInitDef")
                        w1154 = "曲线13" ("值")
                        n935 = invoke on="控件配置文件" class="Tbl (严格)" method="Set Cell Value"("X Index"=1 ("X索引"), "Y Index"=w1155, "Value"="X" ("值")) -> ()  [unwired: 3 in, 6 out]
                        n936 = invoke on="控件配置文件" class="Tbl (严格)" method="Set Cell Value"("X Index"=0 ("X索引"), "Y Index"=w1155, "Value"=w1154) -> ()  [unwired: 3 in, 6 out]
                        n937 = property on="曲线13设置" class="Str"("Val(Sgnl)"=w1154) -> ()  [unwired: 2 in, 2 out]
                      }
                      frame #13 {
                        w1160 = T9 40 items=["刷新间隔", "波特率", "布尔1设置项", "布尔2设置项", "布尔3设置项", "布尔4设置项", "布尔5设置项", "显控1设置", "显控2设置", "显控3设置", "显控4设置", "显控5设置", "显控6设置", "显控7设置", "显控8设置", "显控9设置", "显控10设置", "显控11设置", "显控12设置", "设控1设置", "设控2设置", "设控3设置", "设控4设置", "设控5设置", "设控6设置", "设控7设置", "设控8设置", "曲线1设置", "曲线2设置", "曲线3设置", "曲线4设置", "曲线5设置", "曲线6设置", "曲线7设置", "曲线8设置", "曲线9设置", "曲线10设置", "曲线11设置", "曲线12设置", "曲线13设置", "曲线14设置", "曲线15设置", "曲线16设置", "ID值"] ("DataInitDef")
                        w1159 = "曲线14" ("值")
                        n938 = invoke on="控件配置文件" class="Tbl (严格)" method="Set Cell Value"("X Index"=1 ("X索引"), "Y Index"=w1160, "Value"="X" ("值")) -> ()  [unwired: 3 in, 6 out]
                        n939 = invoke on="控件配置文件" class="Tbl (严格)" method="Set Cell Value"("X Index"=0 ("X索引"), "Y Index"=w1160, "Value"=w1159) -> ()  [unwired: 3 in, 6 out]
                        n940 = property on="曲线14设置" class="Str"("Val(Sgnl)"=w1159) -> ()  [unwired: 2 in, 2 out]
                      }
                      frame #14 {
                        w1165 = T9 41 items=["刷新间隔", "波特率", "布尔1设置项", "布尔2设置项", "布尔3设置项", "布尔4设置项", "布尔5设置项", "显控1设置", "显控2设置", "显控3设置", "显控4设置", "显控5设置", "显控6设置", "显控7设置", "显控8设置", "显控9设置", "显控10设置", "显控11设置", "显控12设置", "设控1设置", "设控2设置", "设控3设置", "设控4设置", "设控5设置", "设控6设置", "设控7设置", "设控8设置", "曲线1设置", "曲线2设置", "曲线3设置", "曲线4设置", "曲线5设置", "曲线6设置", "曲线7设置", "曲线8设置", "曲线9设置", "曲线10设置", "曲线11设置", "曲线12设置", "曲线13设置", "曲线14设置", "曲线15设置", "曲线16设置", "ID值"] ("DataInitDef")
                        w1164 = "曲线15" ("值")
                        n941 = invoke on="控件配置文件" class="Tbl (严格)" method="Set Cell Value"("X Index"=1 ("X索引"), "Y Index"=w1165, "Value"="X" ("值")) -> ()  [unwired: 3 in, 6 out]
                        n942 = invoke on="控件配置文件" class="Tbl (严格)" method="Set Cell Value"("X Index"=0 ("X索引"), "Y Index"=w1165, "Value"=w1164) -> ()  [unwired: 3 in, 6 out]
                        n943 = property on="曲线15设置" class="Str"("Val(Sgnl)"=w1164) -> ()  [unwired: 2 in, 2 out]
                      }
                      frame #15 {
                        w1170 = T9 42 items=["刷新间隔", "波特率", "布尔1设置项", "布尔2设置项", "布尔3设置项", "布尔4设置项", "布尔5设置项", "显控1设置", "显控2设置", "显控3设置", "显控4设置", "显控5设置", "显控6设置", "显控7设置", "显控8设置", "显控9设置", "显控10设置", "显控11设置", "显控12设置", "设控1设置", "设控2设置", "设控3设置", "设控4设置", "设控5设置", "设控6设置", "设控7设置", "设控8设置", "曲线1设置", "曲线2设置", "曲线3设置", "曲线4设置", "曲线5设置", "曲线6设置", "曲线7设置", "曲线8设置", "曲线9设置", "曲线10设置", "曲线11设置", "曲线12设置", "曲线13设置", "曲线14设置", "曲线15设置", "曲线16设置", "ID值"] ("DataInitDef")
                        w1169 = "曲线16" ("值")
                        n944 = invoke on="控件配置文件" class="Tbl (严格)" method="Set Cell Value"("X Index"=1 ("X索引"), "Y Index"=w1170, "Value"="X" ("值")) -> ()  [unwired: 3 in, 6 out]
                        n945 = invoke on="控件配置文件" class="Tbl (严格)" method="Set Cell Value"("X Index"=0 ("X索引"), "Y Index"=w1170, "Value"=w1169) -> ()  [unwired: 3 in, 6 out]
                        n946 = property on="曲线16设置" class="Str"("Val(Sgnl)"=w1169) -> ()  [unwired: 2 in, 2 out]
                      }
                    }
                  }
                  frame "删除曲线8" {
                    w1175 = "曲线8" ("值")
                    w1173 = T9 34 items=["刷新间隔", "波特率", "布尔1设置项", "布尔2设置项", "布尔3设置项", "布尔4设置项", "布尔5设置项", "显控1设置", "显控2设置", "显控3设置", "显控4设置", "显控5设置", "显控6设置", "显控7设置", "显控8设置", "显控9设置", "显控10设置", "显控11设置", "显控12设置", "设控1设置", "设控2设置", "设控3设置", "设控4设置", "设控5设置", "设控6设置", "设控7设置", "设控8设置", "曲线1设置", "曲线2设置", "曲线3设置", "曲线4设置", "曲线5设置", "曲线6设置", "曲线7设置", "曲线8设置", "曲线9设置", "曲线10设置", "曲线11设置", "曲线12设置", "曲线13设置", "曲线14设置", "曲线15设置", "曲线16设置", "ID值"] ("DataInitDef")
                    n947 = invoke on="控件配置文件" class="Tbl (严格)" method="Set Cell Value"("X Index"=1 ("X索引"), "Y Index"=w1173, "Value"="X" ("值")) -> ()  [unwired: 3 in, 6 out]
                    n948 = invoke on="控件配置文件" class="Tbl (严格)" method="Set Cell Value"("X Index"=0 ("X索引"), "Y Index"=w1173, "Value"=w1175) -> ()  [unwired: 3 in, 6 out]
                    n949 = property on="曲线8设置" class="Str"("Val(Sgnl)"=w1175) -> ()  [unwired: 2 in, 2 out]
                  }
                  frame "删除曲线9" {
                    w1178 = T9 35 items=["刷新间隔", "波特率", "布尔1设置项", "布尔2设置项", "布尔3设置项", "布尔4设置项", "布尔5设置项", "显控1设置", "显控2设置", "显控3设置", "显控4设置", "显控5设置", "显控6设置", "显控7设置", "显控8设置", "显控9设置", "显控10设置", "显控11设置", "显控12设置", "设控1设置", "设控2设置", "设控3设置", "设控4设置", "设控5设置", "设控6设置", "设控7设置", "设控8设置", "曲线1设置", "曲线2设置", "曲线3设置", "曲线4设置", "曲线5设置", "曲线6设置", "曲线7设置", "曲线8设置", "曲线9设置", "曲线10设置", "曲线11设置", "曲线12设置", "曲线13设置", "曲线14设置", "曲线15设置", "曲线16设置", "ID值"] ("DataInitDef")
                    w1180 = "曲线9" ("值")
                    n950 = invoke on="控件配置文件" class="Tbl (严格)" method="Set Cell Value"("X Index"=1 ("X索引"), "Y Index"=w1178, "Value"="X" ("值")) -> ()  [unwired: 3 in, 6 out]
                    n951 = invoke on="控件配置文件" class="Tbl (严格)" method="Set Cell Value"("X Index"=0 ("X索引"), "Y Index"=w1178, "Value"=w1180) -> ()  [unwired: 3 in, 6 out]
                    n952 = property on="曲线9设置" class="Str"("Val(Sgnl)"=w1180) -> ()  [unwired: 2 in, 2 out]
                  }
                  frame "删除曲线10" {
                    w1183 = T9 36 items=["刷新间隔", "波特率", "布尔1设置项", "布尔2设置项", "布尔3设置项", "布尔4设置项", "布尔5设置项", "显控1设置", "显控2设置", "显控3设置", "显控4设置", "显控5设置", "显控6设置", "显控7设置", "显控8设置", "显控9设置", "显控10设置", "显控11设置", "显控12设置", "设控1设置", "设控2设置", "设控3设置", "设控4设置", "设控5设置", "设控6设置", "设控7设置", "设控8设置", "曲线1设置", "曲线2设置", "曲线3设置", "曲线4设置", "曲线5设置", "曲线6设置", "曲线7设置", "曲线8设置", "曲线9设置", "曲线10设置", "曲线11设置", "曲线12设置", "曲线13设置", "曲线14设置", "曲线15设置", "曲线16设置", "ID值"] ("DataInitDef")
                    w1185 = "曲线10" ("值")
                    n953 = invoke on="控件配置文件" class="Tbl (严格)" method="Set Cell Value"("X Index"=1 ("X索引"), "Y Index"=w1183, "Value"="X" ("值")) -> ()  [unwired: 3 in, 6 out]
                    n954 = invoke on="控件配置文件" class="Tbl (严格)" method="Set Cell Value"("X Index"=0 ("X索引"), "Y Index"=w1183, "Value"=w1185) -> ()  [unwired: 3 in, 6 out]
                    n955 = property on="曲线10设置" class="Str"("Val(Sgnl)"=w1185) -> ()  [unwired: 2 in, 2 out]
                  }
                  frame "删除曲线11" {
                    w1188 = T9 37 items=["刷新间隔", "波特率", "布尔1设置项", "布尔2设置项", "布尔3设置项", "布尔4设置项", "布尔5设置项", "显控1设置", "显控2设置", "显控3设置", "显控4设置", "显控5设置", "显控6设置", "显控7设置", "显控8设置", "显控9设置", "显控10设置", "显控11设置", "显控12设置", "设控1设置", "设控2设置", "设控3设置", "设控4设置", "设控5设置", "设控6设置", "设控7设置", "设控8设置", "曲线1设置", "曲线2设置", "曲线3设置", "曲线4设置", "曲线5设置", "曲线6设置", "曲线7设置", "曲线8设置", "曲线9设置", "曲线10设置", "曲线11设置", "曲线12设置", "曲线13设置", "曲线14设置", "曲线15设置", "曲线16设置", "ID值"] ("DataInitDef")
                    w1190 = "曲线11" ("值")
                    n956 = invoke on="控件配置文件" class="Tbl (严格)" method="Set Cell Value"("X Index"=1 ("X索引"), "Y Index"=w1188, "Value"="X" ("值")) -> ()  [unwired: 3 in, 6 out]
                    n957 = invoke on="控件配置文件" class="Tbl (严格)" method="Set Cell Value"("X Index"=0 ("X索引"), "Y Index"=w1188, "Value"=w1190) -> ()  [unwired: 3 in, 6 out]
                    n958 = property on="曲线11设置" class="Str"("Val(Sgnl)"=w1190) -> ()  [unwired: 2 in, 2 out]
                  }
                  frame "删除曲线12" {
                    w1193 = T9 38 items=["刷新间隔", "波特率", "布尔1设置项", "布尔2设置项", "布尔3设置项", "布尔4设置项", "布尔5设置项", "显控1设置", "显控2设置", "显控3设置", "显控4设置", "显控5设置", "显控6设置", "显控7设置", "显控8设置", "显控9设置", "显控10设置", "显控11设置", "显控12设置", "设控1设置", "设控2设置", "设控3设置", "设控4设置", "设控5设置", "设控6设置", "设控7设置", "设控8设置", "曲线1设置", "曲线2设置", "曲线3设置", "曲线4设置", "曲线5设置", "曲线6设置", "曲线7设置", "曲线8设置", "曲线9设置", "曲线10设置", "曲线11设置", "曲线12设置", "曲线13设置", "曲线14设置", "曲线15设置", "曲线16设置", "ID值"] ("DataInitDef")
                    w1195 = "曲线12" ("值")
                    n959 = invoke on="控件配置文件" class="Tbl (严格)" method="Set Cell Value"("X Index"=1 ("X索引"), "Y Index"=w1193, "Value"="X" ("值")) -> ()  [unwired: 3 in, 6 out]
                    n960 = invoke on="控件配置文件" class="Tbl (严格)" method="Set Cell Value"("X Index"=0 ("X索引"), "Y Index"=w1193, "Value"=w1195) -> ()  [unwired: 3 in, 6 out]
                    n961 = property on="曲线12设置" class="Str"("Val(Sgnl)"=w1195) -> ()  [unwired: 2 in, 2 out]
                  }
                  frame "删除曲线13" {
                    w1198 = T9 39 items=["刷新间隔", "波特率", "布尔1设置项", "布尔2设置项", "布尔3设置项", "布尔4设置项", "布尔5设置项", "显控1设置", "显控2设置", "显控3设置", "显控4设置", "显控5设置", "显控6设置", "显控7设置", "显控8设置", "显控9设置", "显控10设置", "显控11设置", "显控12设置", "设控1设置", "设控2设置", "设控3设置", "设控4设置", "设控5设置", "设控6设置", "设控7设置", "设控8设置", "曲线1设置", "曲线2设置", "曲线3设置", "曲线4设置", "曲线5设置", "曲线6设置", "曲线7设置", "曲线8设置", "曲线9设置", "曲线10设置", "曲线11设置", "曲线12设置", "曲线13设置", "曲线14设置", "曲线15设置", "曲线16设置", "ID值"] ("DataInitDef")
                    w1200 = "曲线13" ("值")
                    n962 = invoke on="控件配置文件" class="Tbl (严格)" method="Set Cell Value"("X Index"=1 ("X索引"), "Y Index"=w1198, "Value"="X" ("值")) -> ()  [unwired: 3 in, 6 out]
                    n963 = invoke on="控件配置文件" class="Tbl (严格)" method="Set Cell Value"("X Index"=0 ("X索引"), "Y Index"=w1198, "Value"=w1200) -> ()  [unwired: 3 in, 6 out]
                    n964 = property on="曲线13设置" class="Str"("Val(Sgnl)"=w1200) -> ()  [unwired: 2 in, 2 out]
                  }
                  frame "删除曲线14" {
                    w1203 = T9 40 items=["刷新间隔", "波特率", "布尔1设置项", "布尔2设置项", "布尔3设置项", "布尔4设置项", "布尔5设置项", "显控1设置", "显控2设置", "显控3设置", "显控4设置", "显控5设置", "显控6设置", "显控7设置", "显控8设置", "显控9设置", "显控10设置", "显控11设置", "显控12设置", "设控1设置", "设控2设置", "设控3设置", "设控4设置", "设控5设置", "设控6设置", "设控7设置", "设控8设置", "曲线1设置", "曲线2设置", "曲线3设置", "曲线4设置", "曲线5设置", "曲线6设置", "曲线7设置", "曲线8设置", "曲线9设置", "曲线10设置", "曲线11设置", "曲线12设置", "曲线13设置", "曲线14设置", "曲线15设置", "曲线16设置", "ID值"] ("DataInitDef")
                    w1205 = "曲线14" ("值")
                    n965 = invoke on="控件配置文件" class="Tbl (严格)" method="Set Cell Value"("X Index"=1 ("X索引"), "Y Index"=w1203, "Value"="X" ("值")) -> ()  [unwired: 3 in, 6 out]
                    n966 = invoke on="控件配置文件" class="Tbl (严格)" method="Set Cell Value"("X Index"=0 ("X索引"), "Y Index"=w1203, "Value"=w1205) -> ()  [unwired: 3 in, 6 out]
                    n967 = property on="曲线14设置" class="Str"("Val(Sgnl)"=w1205) -> ()  [unwired: 2 in, 2 out]
                  }
                  frame "删除曲线15" {
                    w1208 = T9 41 items=["刷新间隔", "波特率", "布尔1设置项", "布尔2设置项", "布尔3设置项", "布尔4设置项", "布尔5设置项", "显控1设置", "显控2设置", "显控3设置", "显控4设置", "显控5设置", "显控6设置", "显控7设置", "显控8设置", "显控9设置", "显控10设置", "显控11设置", "显控12设置", "设控1设置", "设控2设置", "设控3设置", "设控4设置", "设控5设置", "设控6设置", "设控7设置", "设控8设置", "曲线1设置", "曲线2设置", "曲线3设置", "曲线4设置", "曲线5设置", "曲线6设置", "曲线7设置", "曲线8设置", "曲线9设置", "曲线10设置", "曲线11设置", "曲线12设置", "曲线13设置", "曲线14设置", "曲线15设置", "曲线16设置", "ID值"] ("DataInitDef")
                    w1210 = "曲线15" ("值")
                    n968 = invoke on="控件配置文件" class="Tbl (严格)" method="Set Cell Value"("X Index"=1 ("X索引"), "Y Index"=w1208, "Value"="X" ("值")) -> ()  [unwired: 3 in, 6 out]
                    n969 = invoke on="控件配置文件" class="Tbl (严格)" method="Set Cell Value"("X Index"=0 ("X索引"), "Y Index"=w1208, "Value"=w1210) -> ()  [unwired: 3 in, 6 out]
                    n970 = property on="曲线15设置" class="Str"("Val(Sgnl)"=w1210) -> ()  [unwired: 2 in, 2 out]
                  }
                  frame "删除曲线16" {
                    w1213 = T9 42 items=["刷新间隔", "波特率", "布尔1设置项", "布尔2设置项", "布尔3设置项", "布尔4设置项", "布尔5设置项", "显控1设置", "显控2设置", "显控3设置", "显控4设置", "显控5设置", "显控6设置", "显控7设置", "显控8设置", "显控9设置", "显控10设置", "显控11设置", "显控12设置", "设控1设置", "设控2设置", "设控3设置", "设控4设置", "设控5设置", "设控6设置", "设控7设置", "设控8设置", "曲线1设置", "曲线2设置", "曲线3设置", "曲线4设置", "曲线5设置", "曲线6设置", "曲线7设置", "曲线8设置", "曲线9设置", "曲线10设置", "曲线11设置", "曲线12设置", "曲线13设置", "曲线14设置", "曲线15设置", "曲线16设置", "ID值"] ("DataInitDef")
                    w1215 = "曲线16" ("值")
                    n971 = invoke on="控件配置文件" class="Tbl (严格)" method="Set Cell Value"("X Index"=1 ("X索引"), "Y Index"=w1213, "Value"="X" ("值")) -> ()  [unwired: 3 in, 6 out]
                    n972 = invoke on="控件配置文件" class="Tbl (严格)" method="Set Cell Value"("X Index"=0 ("X索引"), "Y Index"=w1213, "Value"=w1215) -> ()  [unwired: 3 in, 6 out]
                    n973 = property on="曲线16设置" class="Str"("Val(Sgnl)"=w1215) -> ()  [unwired: 2 in, 2 out]
                  }
                }
              }
              event "设控1": Shortcut Menu Selection (User) {
                w1218 = T9 19 items=["刷新间隔", "波特率", "布尔1设置项", "布尔2设置项", "布尔3设置项", "布尔4设置项", "布尔5设置项", "显控1设置", "显控2设置", "显控3设置", "显控4设置", "显控5设置", "显控6设置", "显控7设置", "显控8设置", "显控9设置", "显控10设置", "显控11设置", "显控12设置", "设控1设置", "设控2设置", "设控3设置", "设控4设置", "设控5设置", "设控6设置", "设控7设置", "设控8设置", "曲线1设置", "曲线2设置", "曲线3设置", "曲线4设置", "曲线5设置", "曲线6设置", "曲线7设置", "曲线8设置", "曲线9设置", "曲线10设置", "曲线11设置", "曲线12设置", "曲线13设置", "曲线14设置", "曲线15设置", "曲线16设置", "ID值"] ("DataInitDef")
                w1220 = "设控1" ("标题.文本")
                n974 = event-data() -> ()  [unwired: 1 in, 8 out]
                n975 = invoke on="控件配置文件" class="Tbl (严格)" method="Set Cell Value"("X Index"=1 ("X索引"), "Y Index"=w1218, "Value"="X" ("值")) -> ()  [unwired: 3 in, 6 out]
                n976 = invoke on="控件配置文件" class="Tbl (严格)" method="Set Cell Value"("X Index"=0 ("X索引"), "Y Index"=w1218, "Value"=w1220) -> ()  [unwired: 3 in, 6 out]
                n977 = property on="设控1" class="Str"("Caption.Text"=w1220) -> ()  [unwired: 2 in, 2 out]
                n978 = property on="设控设置 1" class="Str"("Val(Sgnl)"=w1220) -> ()  [unwired: 2 in, 2 out]
              }
              event "设控2": Shortcut Menu Selection (User) {
                w1223 = T9 20 items=["刷新间隔", "波特率", "布尔1设置项", "布尔2设置项", "布尔3设置项", "布尔4设置项", "布尔5设置项", "显控1设置", "显控2设置", "显控3设置", "显控4设置", "显控5设置", "显控6设置", "显控7设置", "显控8设置", "显控9设置", "显控10设置", "显控11设置", "显控12设置", "设控1设置", "设控2设置", "设控3设置", "设控4设置", "设控5设置", "设控6设置", "设控7设置", "设控8设置", "曲线1设置", "曲线2设置", "曲线3设置", "曲线4设置", "曲线5设置", "曲线6设置", "曲线7设置", "曲线8设置", "曲线9设置", "曲线10设置", "曲线11设置", "曲线12设置", "曲线13设置", "曲线14设置", "曲线15设置", "曲线16设置", "ID值"] ("DataInitDef")
                w1225 = "设控2" ("标题.文本")
                n979 = event-data() -> ()  [unwired: 1 in, 8 out]
                n980 = invoke on="控件配置文件" class="Tbl (严格)" method="Set Cell Value"("X Index"=1 ("X索引"), "Y Index"=w1223, "Value"="X" ("值")) -> ()  [unwired: 3 in, 6 out]
                n981 = invoke on="控件配置文件" class="Tbl (严格)" method="Set Cell Value"("X Index"=0 ("X索引"), "Y Index"=w1223, "Value"=w1225) -> ()  [unwired: 3 in, 6 out]
                n982 = property on="设控2" class="Str"("Caption.Text"=w1225) -> ()  [unwired: 2 in, 2 out]
                n983 = property on="设控设置 2" class="Str"("Val(Sgnl)"=w1225) -> ()  [unwired: 2 in, 2 out]
              }
              event "设控3": Shortcut Menu Selection (User) {
                w1228 = T9 21 items=["刷新间隔", "波特率", "布尔1设置项", "布尔2设置项", "布尔3设置项", "布尔4设置项", "布尔5设置项", "显控1设置", "显控2设置", "显控3设置", "显控4设置", "显控5设置", "显控6设置", "显控7设置", "显控8设置", "显控9设置", "显控10设置", "显控11设置", "显控12设置", "设控1设置", "设控2设置", "设控3设置", "设控4设置", "设控5设置", "设控6设置", "设控7设置", "设控8设置", "曲线1设置", "曲线2设置", "曲线3设置", "曲线4设置", "曲线5设置", "曲线6设置", "曲线7设置", "曲线8设置", "曲线9设置", "曲线10设置", "曲线11设置", "曲线12设置", "曲线13设置", "曲线14设置", "曲线15设置", "曲线16设置", "ID值"] ("DataInitDef")
                w1230 = "设控3" ("标题.文本")
                n984 = event-data() -> ()  [unwired: 1 in, 8 out]
                n985 = invoke on="控件配置文件" class="Tbl (严格)" method="Set Cell Value"("X Index"=1 ("X索引"), "Y Index"=w1228, "Value"="X" ("值")) -> ()  [unwired: 3 in, 6 out]
                n986 = invoke on="控件配置文件" class="Tbl (严格)" method="Set Cell Value"("X Index"=0 ("X索引"), "Y Index"=w1228, "Value"=w1230) -> ()  [unwired: 3 in, 6 out]
                n987 = property on="设控3" class="Str"("Caption.Text"=w1230) -> ()  [unwired: 2 in, 2 out]
                n988 = property on="设控设置 3" class="Str"("Val(Sgnl)"=w1230) -> ()  [unwired: 2 in, 2 out]
              }
              event "设控4": Shortcut Menu Selection (User) {
                w1233 = T9 22 items=["刷新间隔", "波特率", "布尔1设置项", "布尔2设置项", "布尔3设置项", "布尔4设置项", "布尔5设置项", "显控1设置", "显控2设置", "显控3设置", "显控4设置", "显控5设置", "显控6设置", "显控7设置", "显控8设置", "显控9设置", "显控10设置", "显控11设置", "显控12设置", "设控1设置", "设控2设置", "设控3设置", "设控4设置", "设控5设置", "设控6设置", "设控7设置", "设控8设置", "曲线1设置", "曲线2设置", "曲线3设置", "曲线4设置", "曲线5设置", "曲线6设置", "曲线7设置", "曲线8设置", "曲线9设置", "曲线10设置", "曲线11设置", "曲线12设置", "曲线13设置", "曲线14设置", "曲线15设置", "曲线16设置", "ID值"] ("DataInitDef")
                w1235 = "设控4" ("标题.文本")
                n989 = event-data() -> ()  [unwired: 1 in, 8 out]
                n990 = invoke on="控件配置文件" class="Tbl (严格)" method="Set Cell Value"("X Index"=1 ("X索引"), "Y Index"=w1233, "Value"="X" ("值")) -> ()  [unwired: 3 in, 6 out]
                n991 = invoke on="控件配置文件" class="Tbl (严格)" method="Set Cell Value"("X Index"=0 ("X索引"), "Y Index"=w1233, "Value"=w1235) -> ()  [unwired: 3 in, 6 out]
                n992 = property on="设控4" class="Str"("Caption.Text"=w1235) -> ()  [unwired: 2 in, 2 out]
                n993 = property on="设控设置 4" class="Str"("Val(Sgnl)"=w1235) -> ()  [unwired: 2 in, 2 out]
              }
              event "设控5": Shortcut Menu Selection (User) {
                w1240 = T9 23 items=["刷新间隔", "波特率", "布尔1设置项", "布尔2设置项", "布尔3设置项", "布尔4设置项", "布尔5设置项", "显控1设置", "显控2设置", "显控3设置", "显控4设置", "显控5设置", "显控6设置", "显控7设置", "显控8设置", "显控9设置", "显控10设置", "显控11设置", "显控12设置", "设控1设置", "设控2设置", "设控3设置", "设控4设置", "设控5设置", "设控6设置", "设控7设置", "设控8设置", "曲线1设置", "曲线2设置", "曲线3设置", "曲线4设置", "曲线5设置", "曲线6设置", "曲线7设置", "曲线8设置", "曲线9设置", "曲线10设置", "曲线11设置", "曲线12设置", "曲线13设置", "曲线14设置", "曲线15设置", "曲线16设置", "ID值"] ("DataInitDef")
                w1239 = "设控5" ("标题.文本")
                n994 = event-data() -> ()  [unwired: 1 in, 8 out]
                n995 = invoke on="控件配置文件" class="Tbl (严格)" method="Set Cell Value"("X Index"=1 ("X索引"), "Y Index"=w1240, "Value"="X" ("值")) -> ()  [unwired: 3 in, 6 out]
                n996 = invoke on="控件配置文件" class="Tbl (严格)" method="Set Cell Value"("X Index"=0 ("X索引"), "Y Index"=w1240, "Value"=w1239) -> ()  [unwired: 3 in, 6 out]
                n997 = property on="设控5" class="Str"("Caption.Text"=w1239) -> ()  [unwired: 2 in, 2 out]
                n998 = property on="设控设置 5" class="Str"("Val(Sgnl)"=w1239) -> ()  [unwired: 2 in, 2 out]
              }
              event "设控6": Shortcut Menu Selection (User) {
                w1245 = T9 24 items=["刷新间隔", "波特率", "布尔1设置项", "布尔2设置项", "布尔3设置项", "布尔4设置项", "布尔5设置项", "显控1设置", "显控2设置", "显控3设置", "显控4设置", "显控5设置", "显控6设置", "显控7设置", "显控8设置", "显控9设置", "显控10设置", "显控11设置", "显控12设置", "设控1设置", "设控2设置", "设控3设置", "设控4设置", "设控5设置", "设控6设置", "设控7设置", "设控8设置", "曲线1设置", "曲线2设置", "曲线3设置", "曲线4设置", "曲线5设置", "曲线6设置", "曲线7设置", "曲线8设置", "曲线9设置", "曲线10设置", "曲线11设置", "曲线12设置", "曲线13设置", "曲线14设置", "曲线15设置", "曲线16设置", "ID值"] ("DataInitDef")
                w1244 = "设控6" ("标题.文本")
                n999 = event-data() -> ()  [unwired: 1 in, 8 out]
                n1000 = invoke on="控件配置文件" class="Tbl (严格)" method="Set Cell Value"("X Index"=1 ("X索引"), "Y Index"=w1245, "Value"="X" ("值")) -> ()  [unwired: 3 in, 6 out]
                n1001 = invoke on="控件配置文件" class="Tbl (严格)" method="Set Cell Value"("X Index"=0 ("X索引"), "Y Index"=w1245, "Value"=w1244) -> ()  [unwired: 3 in, 6 out]
                n1002 = property on="设控6" class="Str"("Caption.Text"=w1244) -> ()  [unwired: 2 in, 2 out]
                n1003 = property on="设控设置 6" class="Str"("Val(Sgnl)"=w1244) -> ()  [unwired: 2 in, 2 out]
              }
              event "设控7": Shortcut Menu Selection (User) {
                w1248 = T9 25 items=["刷新间隔", "波特率", "布尔1设置项", "布尔2设置项", "布尔3设置项", "布尔4设置项", "布尔5设置项", "显控1设置", "显控2设置", "显控3设置", "显控4设置", "显控5设置", "显控6设置", "显控7设置", "显控8设置", "显控9设置", "显控10设置", "显控11设置", "显控12设置", "设控1设置", "设控2设置", "设控3设置", "设控4设置", "设控5设置", "设控6设置", "设控7设置", "设控8设置", "曲线1设置", "曲线2设置", "曲线3设置", "曲线4设置", "曲线5设置", "曲线6设置", "曲线7设置", "曲线8设置", "曲线9设置", "曲线10设置", "曲线11设置", "曲线12设置", "曲线13设置", "曲线14设置", "曲线15设置", "曲线16设置", "ID值"] ("DataInitDef")
                w1250 = "设控7" ("标题.文本")
                n1004 = event-data() -> ()  [unwired: 1 in, 8 out]
                n1005 = invoke on="控件配置文件" class="Tbl (严格)" method="Set Cell Value"("X Index"=1 ("X索引"), "Y Index"=w1248, "Value"="X" ("值")) -> ()  [unwired: 3 in, 6 out]
                n1006 = invoke on="控件配置文件" class="Tbl (严格)" method="Set Cell Value"("X Index"=0 ("X索引"), "Y Index"=w1248, "Value"=w1250) -> ()  [unwired: 3 in, 6 out]
                n1007 = property on="设控7" class="Str"("Caption.Text"=w1250) -> ()  [unwired: 2 in, 2 out]
                n1008 = property on="设控设置 7" class="Str"("Val(Sgnl)"=w1250) -> ()  [unwired: 2 in, 2 out]
              }
              event "设控8": Shortcut Menu Selection (User) {
                w1253 = T9 26 items=["刷新间隔", "波特率", "布尔1设置项", "布尔2设置项", "布尔3设置项", "布尔4设置项", "布尔5设置项", "显控1设置", "显控2设置", "显控3设置", "显控4设置", "显控5设置", "显控6设置", "显控7设置", "显控8设置", "显控9设置", "显控10设置", "显控11设置", "显控12设置", "设控1设置", "设控2设置", "设控3设置", "设控4设置", "设控5设置", "设控6设置", "设控7设置", "设控8设置", "曲线1设置", "曲线2设置", "曲线3设置", "曲线4设置", "曲线5设置", "曲线6设置", "曲线7设置", "曲线8设置", "曲线9设置", "曲线10设置", "曲线11设置", "曲线12设置", "曲线13设置", "曲线14设置", "曲线15设置", "曲线16设置", "ID值"] ("DataInitDef")
                w1255 = "设控8" ("标题.文本")
                n1009 = event-data() -> ()  [unwired: 1 in, 8 out]
                n1010 = invoke on="控件配置文件" class="Tbl (严格)" method="Set Cell Value"("X Index"=1 ("X索引"), "Y Index"=w1253, "Value"="X" ("值")) -> ()  [unwired: 3 in, 6 out]
                n1011 = invoke on="控件配置文件" class="Tbl (严格)" method="Set Cell Value"("X Index"=0 ("X索引"), "Y Index"=w1253, "Value"=w1255) -> ()  [unwired: 3 in, 6 out]
                n1012 = property on="设控8" class="Str"("Caption.Text"=w1255) -> ()  [unwired: 2 in, 2 out]
                n1013 = property on="设控设置 8" class="Str"("Val(Sgnl)"=w1255) -> ()  [unwired: 2 in, 2 out]
              }
            }
          }
          frame #4 {
            # "导入表格参数处理代码"
            n1014 = event shown="[1] \"选择参数表\": 值改变" {
              selector: _ -> [_ _]
              dyn-events: _ -> [_ _]
              timeout: 0 -> [_ _]
              event Timeout {
                n1015 = event-data() -> ()  [unwired: 1 in, 3 out]
              }
              event "选择参数表": Value Change {
                # "读取指定的EXCEL文件，从中导入要显示的参数"
                n1016 = event-data() -> ()  [unwired: 1 in, 3 out]
                n1017 = flat-sequence {
                  tunnel: ["选择参数表"] -> w1262
                  tunnel: [w1265] -> w1261
                  tunnel: [w1264] -> w1260
                  tunnel: w1262 -> [w1277]
                  tunnel: w1261 -> [w1276]
                  tunnel: w1260 -> [w1272]
                  tunnel: [w1277] -> w1259
                  tunnel: [w1276] -> w1258
                  tunnel: [w1271] -> w1257
                  tunnel: w1259 -> [w1288]
                  tunnel: w1258 -> [w1289]
                  tunnel: w1257 -> [w1287]
                  frame #0 {
                    n1018 = call <vilib>:"Create Report.vi"("report type"=Report_Type."Excel", "template (empty)"="选择参数表") -> ("report out"=w1269:refnum<class "NI_report.lvclass">, "error out"=w1268:errorcluster)  [unwired: 12 in]
                    n1019 = call <vilib>:"Excel Get Last Row.vi"("report in"=w1269, "error in (no error)"=w1268) -> ("report out"=w1267:refnum<class "NI_report.lvclass">, "MS Office parameters out"=w1264:T11, "error out"=w1266:errorcluster)  [unwired: 11 in]
                    n1020 = call-dynamic "Dispose Report.vi"("report in"=w1267, "error in (no error)"=w1266) -> ("error out"=w1265:errorcluster)  [unwired: 13 in]
                  }
                  frame #1 {
                    n1021 = Unbundle By Name(w1272) -> ("position (excel)"=w1273:cluster{"row":i32, "column":i32})
                    n1022 = Unbundle By Name(w1273) -> ("row"=w1274:i32)
                    n1023 = Bundle By Name(cluster=w1273, "row"=w1274, "column"=9) -> (w1271:cluster{"row":i32, "column":i32})
                  }
                  frame #2 {
                    n1024 = call "Excel Read.vi"("error in (no error)"=w1289, "end (-1, -1)"=w1287, "start (-1, -1)"=cluster{"row":i32, "column":i32} {"row"=0, "column"=0}, "template (empty)"=w1288) -> ("error out"=w1286:errorcluster, "Array"=w1281:string[][])  [unwired: 6 in]
                    n1025 = Unbundle By Name(w1286) -> ("status"=w1284:bool, "source"=w1285:string)  [unwired: 1 out]
                    n1026 = Array To Spreadsheet String(array=w1281, 3:"%s" ("格式字符串")) -> (spreadsheet string=w1283:string)  [unwired: 1 in]
                    n1027 = call <vilib>:"Application Directory.vi"() -> ("Application Directory"=w1279:path)
                    n1028 = call "显示对话框信息"("Enable"=w1284, "Message"=w1285) -> ()  [unwired: 8 in, 2 out]
                    n1029 = Build Path(base path=w1279, name or relative path="Config\\DATA.txt" ("名称或相对路径")) -> (appended path=w1278:path)
                    n1030 = Write to Text File(file (use dialog)=w1278, text=w1283) -> ()  [unwired: 2 in, 3 out]
                  }
                }
              }
            }
          }
        }
      }
      frame #2 {
        # "更新与显示有关的控件"
        n1031 = Quotient & Remainder(x="i2", y=10) -> (x-y*floor(x/y)=w1294:u32)  [unwired: 1 out]
        n1032 = Increment(x="i2") -> (x+1=w1293:u32)
        n1033 = Equal To 0?(x=w1294) -> (x = 0?=w1291:bool)
        n1034 = local write "i2"(w1293) -> ()
        n1035 = case shown="真" w1291 {
          frame False {
          }
          frame True {
            n1036 = stacked-sequence {
              frame #0 {
                # "发送跟新的值"
                n1037 = property on="CANBURF" class="Arr (严格)"() -> ("Value"=w1301:u32[][])  [unwired: 2 in, 2 out]
                n1038 = event shown="[1] \"要发送的数据\": 值改变" {
                  selector: _ -> [_ _]
                  dyn-events: _ -> [_ _]
                  timeout: 0 -> [_ _]
                  tunnel: w1301 -> [w1303 w1308]
                  tunnel: [w1303 w1309] -> w1299
                  event Timeout {
                    n1039 = event-data() -> ()  [unwired: 1 in, 3 out]
                  }
                  event "要发送的数据": Value Change {
                    # "实时修改参数设置控件更新的值"
                    n1040 = event-data() -> ("NewVal"=w1310:cluster{"地址":u16, "数据":i32, "行数":i32, "ID":i32})  [unwired: 1 in, 5 out]
                    n1041 = Unbundle(w1310) -> ("地址"=w1304:u16, "数据"=w1305:i32)  [unwired: 2 out]
                    n1042 = flat-sequence {
                      tunnel: w1305 -> [w1315]
                      tunnel: w1308 -> [w1312]
                      tunnel: [w1315] -> w1307
                      tunnel: [w1313] -> w1306
                      tunnel: w1304 -> [w1314]
                      tunnel: w1307 -> [w1331]
                      tunnel: w1306 -> [w1330]
                      tunnel: [w1328] -> w1309
                      tunnel: w1308 -> [w1327]
                      frame #0 {
                        n1043 = local read "当前显示表格总行数"() -> (w1311:i32)
                        n1044 = while {
                          tunnel: [w1320] -> w1313
                          tunnel: w1312 -> [w1319]
                          tunnel: w1314 -> [w1317]
                          tunnel: w1311 -> [w1316]
                          i -> [w1322]
                          stop <- w1324 stop-if-true
                          # "查找CANBURF中与表格第0行相匹配的行数"
                          n1045 = Greater?(x=w1322, y=w1316) -> (0:w1325:bool)
                          n1046 = Index Array(array=w1319, index (row)=w1322, index (col)=0 ("禁用的索引 (列)")) -> (element=w1318:u32)
                          n1047 = Equal?(x=w1318, y=w1317) -> (x = y?=w1323:bool)
                          n1048 = Or(x=w1323, y=w1325) -> (x .or. y?=w1324:bool)
                          n1049 = Select(t=w1322, s=w1323, f=0) -> (s? t:f=w1320:i32)
                        }
                      }
                      frame #1 {
                        n1050 = Replace Array Subset(array=w1327, new element=w1331, index (row)=w1330, index (col)=1 ("禁用的索引 (列)")) -> (w1328:u32[][])
                        n1051 = local write "CANBURF"(w1328) -> ()
                      }
                    }
                  }
                }
                n1052 = local read "表格"() -> (w1298:string[][])
                n1053 = local read "当前显示表格总行数"() -> (w1300:i32)
                n1054 = call "表格显示内容刷新V2.vi"("数据模式"="数据模式", "表格"=w1298, "CANBURF"=w1299, "当前显示表格总行数"=w1300) -> ("输出数组"=w1297:string[][])  [unwired: 7 in]
                n1055 = property on="表格" class="Tbl (严格)"("Value"=w1297) -> ()  [unwired: 2 in, 2 out]
              }
              frame #1 {
                # "故障状态显示，请修改config文件夹下的ERROR.TXT故障字典的内容，务必填写正确的故障地址"
                n1056 = stacked-sequence {
                  frame #0 {
                    # "从故障字典中获取代表故障信息的地址"
                    n1057 = local read "故障地址"() -> (w1335:string[])
                    n1058 = local read "故障字典"() -> (w1332:string[][])
                    n1059 = Array Size(array=w1335) -> (size(s)=w1336:i32)
                    n1060 = Delete From Array "删除数组元素"(array=w1335, length=w1336) -> (array with subset deleted=w1334:string[])  [unwired: 1 in, 1 out]
                    n1061 = for "For循环" {
                      tunnel: w1332 -> [w1341] mode=indexing
                      shift-right: [w1340] -> w1333
                      shift-left: w1334 -> [w1339]
                      n1062 = Index Array(array=w1341, index=1 ("禁用的索引 (列)")) -> (element=w1342:string)
                      n1063 = Index Array(array=w1341, index=0 ("禁用的索引 (列)")) -> (element=w1345:string)
                      n1064 = Equal?(x=w1345, y="") -> ()  [unwired: 1 out]
                      n1065 = Equal?(x=w1345, y="地址") -> (x = y?=w1343:bool)
                      n1066 = case shown="真" w1343 {
                        tunnel: w1342 -> [_ w1350]
                        tunnel: [w1347 w1349] -> w1340
                        tunnel: w1339 -> [w1347 w1348]
                        frame False {
                        }
                        frame True {
                          n1067 = Build Array (concatenate)(w1348, w1350) -> (w1349:string[])
                        }
                      }
                    }
                    "故障地址" <- w1333
                  }
                  frame #1 {
                    # "通过故障地址搜索表格的对应位置获取故障信息"
                    n1068 = local read "故障地址"() -> (w1353:string[])
                    n1069 = local read "表格"() -> (w1352:string[][])
                    n1070 = for "For循环" {
                      tunnel: w1353 -> [w1354] mode=indexing
                      tunnel: w1352 -> [w1356]
                      tunnel: [w1355] -> w1351 mode=indexing
                      n1071 = while {
                        tunnel: w1356 -> [w1360]
                        tunnel: w1354 -> [w1365]
                        tunnel: [w1358] -> w1355
                        i -> [w1359]
                        stop <- w1362 stop-if-true
                        n1072 = Index Array(array=w1360, index (row)=w1359, index (col)=1 ("禁用的索引 (列)")) -> (element=w1357:string)
                        n1073 = Equal?(x=w1357, y="") -> (x = y?=w1363:bool)
                        n1074 = Equal?(x=w1365, y=w1357) -> (x = y?=w1361:bool)
                        n1075 = Or(x=w1361, y=w1363) -> (x .or. y?=w1362:bool)
                        n1076 = case shown="真" w1361 {
                          tunnel: w1360 -> [_ w1370]
                          tunnel: w1359 -> [_ w1369]
                          tunnel: [_ w1367] -> w1358
                          frame False {
                          }
                          frame True {
                            n1077 = Index Array(array=w1370, index (row)=w1369, index (col)=2 ("禁用的索引 (列)")) -> (element=w1367:string)
                          }
                        }
                      }
                    }
                    "故障信息" <- w1351
                  }
                  frame #2 {
                    # "将故障信息中的每一个位于故障字典的内容对应起来，并将等于1的故障位的内容挑选出来"
                    n1078 = local read "故障信息"() -> (w1375:string[])
                    n1079 = local read "故障内容"() -> (w1374:string[])
                    n1080 = local read "故障字典"() -> (w1373:string[][])
                    n1081 = local read "数据模式"() -> (w1371:bool)
                    n1082 = call "故障处理.vi"("数据模式"=w1371, "故障字典"=w1373, "原故障内容"=w1374, "故障信息"=w1375) -> ("故障内容"=w1372:string[])  [unwired: 7 in]
                    n1083 = local write "故障内容"(w1372) -> ()
                  }
                  frame #3 {
                    # "将对应故障内容显示在屏幕上"
                    n1084 = local read "故障内容"() -> (w1381:string[])
                    n1085 = Array To Spreadsheet String(delimiter (Tab)="\n" ("分隔符(Tab)"), array=w1381, 3:"%s" ("格式字符串")) -> (spreadsheet string=w1376:string)
                    n1086 = Not Equal?(x=w1376, y="") -> (x != y?=w1377:bool)
                    n1087 = case shown="真" w1377 {
                      tunnel: w1376 -> [_ w1385]
                      frame False {
                        n1088 = property on="状态显示" class="Str"("Text.TextColor"=u32 0 ("文本.文本颜色:文本颜色")) -> ()  [unwired: 2 in, 2 out]
                        n1089 = local write "状态显示"("无故障" ("状态显示")) -> ()
                      }
                      frame True {
                        n1090 = local write "状态显示"(w1385) -> ()
                        n1091 = property on="状态显示" class="Str"("Text.TextColor"=u32 16711680 ("文本.文本颜色:文本颜色")) -> ()  [unwired: 2 in, 2 out]
                      }
                    }
                  }
                }
              }
              frame #2 {
                w1398 = T9 21 items=["刷新间隔", "波特率", "布尔1设置项", "布尔2设置项", "布尔3设置项", "布尔4设置项", "布尔5设置项", "显控1设置", "显控2设置", "显控3设置", "显控4设置", "显控5设置", "显控6设置", "显控7设置", "显控8设置", "显控9设置", "显控10设置", "显控11设置", "显控12设置", "设控1设置", "设控2设置", "设控3设置", "设控4设置", "设控5设置", "设控6设置", "设控7设置", "设控8设置", "曲线1设置", "曲线2设置", "曲线3设置", "曲线4设置", "曲线5设置", "曲线6设置", "曲线7设置", "曲线8设置", "曲线9设置", "曲线10设置", "曲线11设置", "曲线12设置", "曲线13设置", "曲线14设置", "曲线15设置", "曲线16设置", "ID值"] ("DataInitDef")
                w1399 = T9 20 items=["刷新间隔", "波特率", "布尔1设置项", "布尔2设置项", "布尔3设置项", "布尔4设置项", "布尔5设置项", "显控1设置", "显控2设置", "显控3设置", "显控4设置", "显控5设置", "显控6设置", "显控7设置", "显控8设置", "显控9设置", "显控10设置", "显控11设置", "显控12设置", "设控1设置", "设控2设置", "设控3设置", "设控4设置", "设控5设置", "设控6设置", "设控7设置", "设控8设置", "曲线1设置", "曲线2设置", "曲线3设置", "曲线4设置", "曲线5设置", "曲线6设置", "曲线7设置", "曲线8设置", "曲线9设置", "曲线10设置", "曲线11设置", "曲线12设置", "曲线13设置", "曲线14设置", "曲线15设置", "曲线16设置", "ID值"] ("DataInitDef")
                w1400 = T9 22 items=["刷新间隔", "波特率", "布尔1设置项", "布尔2设置项", "布尔3设置项", "布尔4设置项", "布尔5设置项", "显控1设置", "显控2设置", "显控3设置", "显控4设置", "显控5设置", "显控6设置", "显控7设置", "显控8设置", "显控9设置", "显控10设置", "显控11设置", "显控12设置", "设控1设置", "设控2设置", "设控3设置", "设控4设置", "设控5设置", "设控6设置", "设控7设置", "设控8设置", "曲线1设置", "曲线2设置", "曲线3设置", "曲线4设置", "曲线5设置", "曲线6设置", "曲线7设置", "曲线8设置", "曲线9设置", "曲线10设置", "曲线11设置", "曲线12设置", "曲线13设置", "曲线14设置", "曲线15设置", "曲线16设置", "ID值"] ("DataInitDef")
                w1401 = T9 23 items=["刷新间隔", "波特率", "布尔1设置项", "布尔2设置项", "布尔3设置项", "布尔4设置项", "布尔5设置项", "显控1设置", "显控2设置", "显控3设置", "显控4设置", "显控5设置", "显控6设置", "显控7设置", "显控8设置", "显控9设置", "显控10设置", "显控11设置", "显控12设置", "设控1设置", "设控2设置", "设控3设置", "设控4设置", "设控5设置", "设控6设置", "设控7设置", "设控8设置", "曲线1设置", "曲线2设置", "曲线3设置", "曲线4设置", "曲线5设置", "曲线6设置", "曲线7设置", "曲线8设置", "曲线9设置", "曲线10设置", "曲线11设置", "曲线12设置", "曲线13设置", "曲线14设置", "曲线15设置", "曲线16设置", "ID值"] ("DataInitDef")
                w1402 = T9 24 items=["刷新间隔", "波特率", "布尔1设置项", "布尔2设置项", "布尔3设置项", "布尔4设置项", "布尔5设置项", "显控1设置", "显控2设置", "显控3设置", "显控4设置", "显控5设置", "显控6设置", "显控7设置", "显控8设置", "显控9设置", "显控10设置", "显控11设置", "显控12设置", "设控1设置", "设控2设置", "设控3设置", "设控4设置", "设控5设置", "设控6设置", "设控7设置", "设控8设置", "曲线1设置", "曲线2设置", "曲线3设置", "曲线4设置", "曲线5设置", "曲线6设置", "曲线7设置", "曲线8设置", "曲线9设置", "曲线10设置", "曲线11设置", "曲线12设置", "曲线13设置", "曲线14设置", "曲线15设置", "曲线16设置", "ID值"] ("DataInitDef")
                w1403 = T9 25 items=["刷新间隔", "波特率", "布尔1设置项", "布尔2设置项", "布尔3设置项", "布尔4设置项", "布尔5设置项", "显控1设置", "显控2设置", "显控3设置", "显控4设置", "显控5设置", "显控6设置", "显控7设置", "显控8设置", "显控9设置", "显控10设置", "显控11设置", "显控12设置", "设控1设置", "设控2设置", "设控3设置", "设控4设置", "设控5设置", "设控6设置", "设控7设置", "设控8设置", "曲线1设置", "曲线2设置", "曲线3设置", "曲线4设置", "曲线5设置", "曲线6设置", "曲线7设置", "曲线8设置", "曲线9设置", "曲线10设置", "曲线11设置", "曲线12设置", "曲线13设置", "曲线14设置", "曲线15设置", "曲线16设置", "ID值"] ("DataInitDef")
                w1396 = T9 19 items=["刷新间隔", "波特率", "布尔1设置项", "布尔2设置项", "布尔3设置项", "布尔4设置项", "布尔5设置项", "显控1设置", "显控2设置", "显控3设置", "显控4设置", "显控5设置", "显控6设置", "显控7设置", "显控8设置", "显控9设置", "显控10设置", "显控11设置", "显控12设置", "设控1设置", "设控2设置", "设控3设置", "设控4设置", "设控5设置", "设控6设置", "设控7设置", "设控8设置", "曲线1设置", "曲线2设置", "曲线3设置", "曲线4设置", "曲线5设置", "曲线6设置", "曲线7设置", "曲线8设置", "曲线9设置", "曲线10设置", "曲线11设置", "曲线12设置", "曲线13设置", "曲线14设置", "曲线15设置", "曲线16设置", "ID值"] ("DataInitDef")
                w1397 = T9 26 items=["刷新间隔", "波特率", "布尔1设置项", "布尔2设置项", "布尔3设置项", "布尔4设置项", "布尔5设置项", "显控1设置", "显控2设置", "显控3设置", "显控4设置", "显控5设置", "显控6设置", "显控7设置", "显控8设置", "显控9设置", "显控10设置", "显控11设置", "显控12设置", "设控1设置", "设控2设置", "设控3设置", "设控4设置", "设控5设置", "设控6设置", "设控7设置", "设控8设置", "曲线1设置", "曲线2设置", "曲线3设置", "曲线4设置", "曲线5设置", "曲线6设置", "曲线7设置", "曲线8设置", "曲线9设置", "曲线10设置", "曲线11设置", "曲线12设置", "曲线13设置", "曲线14设置", "曲线15设置", "曲线16设置", "ID值"] ("DataInitDef")
                w1409 = T9 8 items=["刷新间隔", "波特率", "布尔1设置项", "布尔2设置项", "布尔3设置项", "布尔4设置项", "布尔5设置项", "显控1设置", "显控2设置", "显控3设置", "显控4设置", "显控5设置", "显控6设置", "显控7设置", "显控8设置", "显控9设置", "显控10设置", "显控11设置", "显控12设置", "设控1设置", "设控2设置", "设控3设置", "设控4设置", "设控5设置", "设控6设置", "设控7设置", "设控8设置", "曲线1设置", "曲线2设置", "曲线3设置", "曲线4设置", "曲线5设置", "曲线6设置", "曲线7设置", "曲线8设置", "曲线9设置", "曲线10设置", "曲线11设置", "曲线12设置", "曲线13设置", "曲线14设置", "曲线15设置", "曲线16设置", "ID值"] ("DataInitDef")
                w1408 = T9 9 items=["刷新间隔", "波特率", "布尔1设置项", "布尔2设置项", "布尔3设置项", "布尔4设置项", "布尔5设置项", "显控1设置", "显控2设置", "显控3设置", "显控4设置", "显控5设置", "显控6设置", "显控7设置", "显控8设置", "显控9设置", "显控10设置", "显控11设置", "显控12设置", "设控1设置", "设控2设置", "设控3设置", "设控4设置", "设控5设置", "设控6设置", "设控7设置", "设控8设置", "曲线1设置", "曲线2设置", "曲线3设置", "曲线4设置", "曲线5设置", "曲线6设置", "曲线7设置", "曲线8设置", "曲线9设置", "曲线10设置", "曲线11设置", "曲线12设置", "曲线13设置", "曲线14设置", "曲线15设置", "曲线16设置", "ID值"] ("DataInitDef")
                w1407 = T9 10 items=["刷新间隔", "波特率", "布尔1设置项", "布尔2设置项", "布尔3设置项", "布尔4设置项", "布尔5设置项", "显控1设置", "显控2设置", "显控3设置", "显控4设置", "显控5设置", "显控6设置", "显控7设置", "显控8设置", "显控9设置", "显控10设置", "显控11设置", "显控12设置", "设控1设置", "设控2设置", "设控3设置", "设控4设置", "设控5设置", "设控6设置", "设控7设置", "设控8设置", "曲线1设置", "曲线2设置", "曲线3设置", "曲线4设置", "曲线5设置", "曲线6设置", "曲线7设置", "曲线8设置", "曲线9设置", "曲线10设置", "曲线11设置", "曲线12设置", "曲线13设置", "曲线14设置", "曲线15设置", "曲线16设置", "ID值"] ("DataInitDef")
                w1406 = T9 11 items=["刷新间隔", "波特率", "布尔1设置项", "布尔2设置项", "布尔3设置项", "布尔4设置项", "布尔5设置项", "显控1设置", "显控2设置", "显控3设置", "显控4设置", "显控5设置", "显控6设置", "显控7设置", "显控8设置", "显控9设置", "显控10设置", "显控11设置", "显控12设置", "设控1设置", "设控2设置", "设控3设置", "设控4设置", "设控5设置", "设控6设置", "设控7设置", "设控8设置", "曲线1设置", "曲线2设置", "曲线3设置", "曲线4设置", "曲线5设置", "曲线6设置", "曲线7设置", "曲线8设置", "曲线9设置", "曲线10设置", "曲线11设置", "曲线12设置", "曲线13设置", "曲线14设置", "曲线15设置", "曲线16设置", "ID值"] ("DataInitDef")
                w1405 = T9 18 items=["刷新间隔", "波特率", "布尔1设置项", "布尔2设置项", "布尔3设置项", "布尔4设置项", "布尔5设置项", "显控1设置", "显控2设置", "显控3设置", "显控4设置", "显控5设置", "显控6设置", "显控7设置", "显控8设置", "显控9设置", "显控10设置", "显控11设置", "显控12设置", "设控1设置", "设控2设置", "设控3设置", "设控4设置", "设控5设置", "设控6设置", "设控7设置", "设控8设置", "曲线1设置", "曲线2设置", "曲线3设置", "曲线4设置", "曲线5设置", "曲线6设置", "曲线7设置", "曲线8设置", "曲线9设置", "曲线10设置", "曲线11设置", "曲线12设置", "曲线13设置", "曲线14设置", "曲线15设置", "曲线16设置", "ID值"] ("DataInitDef")
                w1404 = T9 12 items=["刷新间隔", "波特率", "布尔1设置项", "布尔2设置项", "布尔3设置项", "布尔4设置项", "布尔5设置项", "显控1设置", "显控2设置", "显控3设置", "显控4设置", "显控5设置", "显控6设置", "显控7设置", "显控8设置", "显控9设置", "显控10设置", "显控11设置", "显控12设置", "设控1设置", "设控2设置", "设控3设置", "设控4设置", "设控5设置", "设控6设置", "设控7设置", "设控8设置", "曲线1设置", "曲线2设置", "曲线3设置", "曲线4设置", "曲线5设置", "曲线6设置", "曲线7设置", "曲线8设置", "曲线9设置", "曲线10设置", "曲线11设置", "曲线12设置", "曲线13设置", "曲线14设置", "曲线15设置", "曲线16设置", "ID值"] ("DataInitDef")
                w1415 = T9 7 items=["刷新间隔", "波特率", "布尔1设置项", "布尔2设置项", "布尔3设置项", "布尔4设置项", "布尔5设置项", "显控1设置", "显控2设置", "显控3设置", "显控4设置", "显控5设置", "显控6设置", "显控7设置", "显控8设置", "显控9设置", "显控10设置", "显控11设置", "显控12设置", "设控1设置", "设控2设置", "设控3设置", "设控4设置", "设控5设置", "设控6设置", "设控7设置", "设控8设置", "曲线1设置", "曲线2设置", "曲线3设置", "曲线4设置", "曲线5设置", "曲线6设置", "曲线7设置", "曲线8设置", "曲线9设置", "曲线10设置", "曲线11设置", "曲线12设置", "曲线13设置", "曲线14设置", "曲线15设置", "曲线16设置", "ID值"] ("DataInitDef")
                w1410 = T9 13 items=["刷新间隔", "波特率", "布尔1设置项", "布尔2设置项", "布尔3设置项", "布尔4设置项", "布尔5设置项", "显控1设置", "显控2设置", "显控3设置", "显控4设置", "显控5设置", "显控6设置", "显控7设置", "显控8设置", "显控9设置", "显控10设置", "显控11设置", "显控12设置", "设控1设置", "设控2设置", "设控3设置", "设控4设置", "设控5设置", "设控6设置", "设控7设置", "设控8设置", "曲线1设置", "曲线2设置", "曲线3设置", "曲线4设置", "曲线5设置", "曲线6设置", "曲线7设置", "曲线8设置", "曲线9设置", "曲线10设置", "曲线11设置", "曲线12设置", "曲线13设置", "曲线14设置", "曲线15设置", "曲线16设置", "ID值"] ("DataInitDef")
                w1414 = T9 14 items=["刷新间隔", "波特率", "布尔1设置项", "布尔2设置项", "布尔3设置项", "布尔4设置项", "布尔5设置项", "显控1设置", "显控2设置", "显控3设置", "显控4设置", "显控5设置", "显控6设置", "显控7设置", "显控8设置", "显控9设置", "显控10设置", "显控11设置", "显控12设置", "设控1设置", "设控2设置", "设控3设置", "设控4设置", "设控5设置", "设控6设置", "设控7设置", "设控8设置", "曲线1设置", "曲线2设置", "曲线3设置", "曲线4设置", "曲线5设置", "曲线6设置", "曲线7设置", "曲线8设置", "曲线9设置", "曲线10设置", "曲线11设置", "曲线12设置", "曲线13设置", "曲线14设置", "曲线15设置", "曲线16设置", "ID值"] ("DataInitDef")
                w1411 = T9 15 items=["刷新间隔", "波特率", "布尔1设置项", "布尔2设置项", "布尔3设置项", "布尔4设置项", "布尔5设置项", "显控1设置", "显控2设置", "显控3设置", "显控4设置", "显控5设置", "显控6设置", "显控7设置", "显控8设置", "显控9设置", "显控10设置", "显控11设置", "显控12设置", "设控1设置", "设控2设置", "设控3设置", "设控4设置", "设控5设置", "设控6设置", "设控7设置", "设控8设置", "曲线1设置", "曲线2设置", "曲线3设置", "曲线4设置", "曲线5设置", "曲线6设置", "曲线7设置", "曲线8设置", "曲线9设置", "曲线10设置", "曲线11设置", "曲线12设置", "曲线13设置", "曲线14设置", "曲线15设置", "曲线16设置", "ID值"] ("DataInitDef")
                w1413 = T9 16 items=["刷新间隔", "波特率", "布尔1设置项", "布尔2设置项", "布尔3设置项", "布尔4设置项", "布尔5设置项", "显控1设置", "显控2设置", "显控3设置", "显控4设置", "显控5设置", "显控6设置", "显控7设置", "显控8设置", "显控9设置", "显控10设置", "显控11设置", "显控12设置", "设控1设置", "设控2设置", "设控3设置", "设控4设置", "设控5设置", "设控6设置", "设控7设置", "设控8设置", "曲线1设置", "曲线2设置", "曲线3设置", "曲线4设置", "曲线5设置", "曲线6设置", "曲线7设置", "曲线8设置", "曲线9设置", "曲线10设置", "曲线11设置", "曲线12设置", "曲线13设置", "曲线14设置", "曲线15设置", "曲线16设置", "ID值"] ("DataInitDef")
                w1412 = T9 17 items=["刷新间隔", "波特率", "布尔1设置项", "布尔2设置项", "布尔3设置项", "布尔4设置项", "布尔5设置项", "显控1设置", "显控2设置", "显控3设置", "显控4设置", "显控5设置", "显控6设置", "显控7设置", "显控8设置", "显控9设置", "显控10设置", "显控11设置", "显控12设置", "设控1设置", "设控2设置", "设控3设置", "设控4设置", "设控5设置", "设控6设置", "设控7设置", "设控8设置", "曲线1设置", "曲线2设置", "曲线3设置", "曲线4设置", "曲线5设置", "曲线6设置", "曲线7设置", "曲线8设置", "曲线9设置", "曲线10设置", "曲线11设置", "曲线12设置", "曲线13设置", "曲线14设置", "曲线15设置", "曲线16设置", "ID值"] ("DataInitDef")
                n1092 = local read "控件配置文件"() -> (w1429:string[][])
                n1093 = local read "表格"() -> (w1428:string[][])
                n1094 = call "显示处理.vi"("项目"=w1411, "配置文件"=w1429, "表格"=w1428) -> ("显示"=→"显控9":string)  [unwired: 8 in]
                n1095 = call "显示处理.vi"("项目"=w1413, "配置文件"=w1429, "表格"=w1428) -> ("显示"=→"显控10":string)  [unwired: 8 in]
                n1096 = call "显示处理.vi"("项目"=w1414, "配置文件"=w1429, "表格"=w1428) -> ("显示"=→"显控8":string)  [unwired: 8 in]
                n1097 = call "显示处理.vi"("项目"=w1410, "配置文件"=w1429, "表格"=w1428) -> ("显示"=→"显控7":string)  [unwired: 8 in]
                n1098 = call "显示处理.vi"("项目"=w1412, "配置文件"=w1429, "表格"=w1428) -> ("显示"=→"显控11":string)  [unwired: 8 in]
                n1099 = call "显示处理.vi"("项目"=w1415, "配置文件"=w1429, "表格"=w1428) -> ("显示"=→"显控1":string)  [unwired: 8 in]
                n1100 = call "显示处理.vi"("项目"=w1408, "配置文件"=w1429, "表格"=w1428) -> ("显示"=→"显控3":string)  [unwired: 8 in]
                n1101 = call "显示处理.vi"("项目"=w1409, "配置文件"=w1429, "表格"=w1428) -> ("显示"=→"显控2":string)  [unwired: 8 in]
                n1102 = call "显示处理.vi"("项目"=w1407, "配置文件"=w1429, "表格"=w1428) -> ("显示"=→"显控4":string)  [unwired: 8 in]
                n1103 = call "显示处理.vi"("项目"=w1406, "配置文件"=w1429, "表格"=w1428) -> ("显示"=→"显控5":string)  [unwired: 8 in]
                n1104 = call "显示处理.vi"("项目"=w1405, "配置文件"=w1429, "表格"=w1428) -> ("显示"=→"显控12":string)  [unwired: 8 in]
                n1105 = call "显示处理.vi"("项目"=w1404, "配置文件"=w1429, "表格"=w1428) -> ("显示"=→"显控6":string)  [unwired: 8 in]
                n1106 = local read "控件配置文件"() -> (w1394:string[][])
                n1107 = local read "表格"() -> (w1395:string[][])
                n1108 = call "显示处理.vi"("项目"=w1396, "配置文件"=w1394, "表格"=w1395) -> ("显示"=w1393:string)  [unwired: 8 in]
                n1109 = call "显示处理.vi"("项目"=w1399, "配置文件"=w1394, "表格"=w1395) -> ("显示"=w1392:string)  [unwired: 8 in]
                n1110 = call "显示处理.vi"("项目"=w1398, "配置文件"=w1394, "表格"=w1395) -> ("显示"=w1391:string)  [unwired: 8 in]
                n1111 = call "显示处理.vi"("项目"=w1400, "配置文件"=w1394, "表格"=w1395) -> ("显示"=w1390:string)  [unwired: 8 in]
                n1112 = call "显示处理.vi"("项目"=w1401, "配置文件"=w1394, "表格"=w1395) -> ("显示"=w1389:string)  [unwired: 8 in]
                n1113 = call "显示处理.vi"("项目"=w1402, "配置文件"=w1394, "表格"=w1395) -> ("显示"=w1388:string)  [unwired: 8 in]
                n1114 = call "显示处理.vi"("项目"=w1403, "配置文件"=w1394, "表格"=w1395) -> ("显示"=w1387:string)  [unwired: 8 in]
                n1115 = call "显示处理.vi"("项目"=w1397, "配置文件"=w1394, "表格"=w1395) -> ("显示"=w1386:string)  [unwired: 8 in]
                n1116 = local write "设控6"(w1388) -> ()
                n1117 = local write "设控7"(w1387) -> ()
                n1118 = local write "设控1"(w1393) -> ()
                n1119 = local write "设控4"(w1390) -> ()
                n1120 = local write "设控8"(w1386) -> ()
                n1121 = local write "设控2"(w1392) -> ()
                n1122 = local write "设控3"(w1391) -> ()
                n1123 = local write "设控5"(w1389) -> ()
              }
            }
          }
        }
      }
      frame #3 {
        n1124 = disable-structure shown="启用" {
          frame Disabled {
          }
          frame Enabled {
          }
        }
      }
    }
    n1125 = Wait on Notification(notifier=w26) -> (error out=w27:errorcluster)  [unwired: 3 in, 3 out]
  }
  n1126 = Build Path(base path=w16, name or relative path="Config\\Config.ini" ("名称或相对路径")) -> (appended path=w15:path)
  n1127 = timed-loop {
    shift-right: [w1447] -> _
    shift-left: w24 -> [w1448]
    shift-right: [w1445] -> w3
    shift-left: errorcluster {"status"=FALSE, "code"=0, "source"=""} ("error constant") -> [w1446]
    tunnel: w15 -> [w1442]
    timing: w20 -> [_]
    timing-out: [_] -> w19
    shift-right: [w1440] -> w13
    shift-left: w10 -> [w1435]
    shift-right: [w1439] -> w12
    shift-left: w14 -> [w1441]
    tunnel: w7 -> [w1434]
    stop <- FALSE stop-if-true
    # "主程序通信VI状态机"
    n1128 = node-c288() -> ()  [unwired: 1 in, 1 out]
    n1129 = Increment(x="i1") -> (x+1=w1430:i32)
    n1130 = case shown="\"Process\"" w1448 {
      tunnel: [w1507 w1538 w1564 w1579 w1733 w1737 w1743] -> w1447
      tunnel: [w1508 FALSE ("停止循环？") FALSE ("停止循环？") FALSE ("停止循环？") TRUE ("停止循环？") FALSE ("停止循环？") FALSE ("布尔 2")] -> _
      tunnel: w1446 -> [_ w1551 w1570 _ w1730 w1739 w1744]
      tunnel: [w1501 w1549 w1561 _ w1732 w1738 w1744] -> w1445
      tunnel: "重新连接" -> [w1506 w1537 w1563 w1578 _ _ _]
      tunnel: w1430 -> [_ _ _ w1572 _ _ _]
      tunnel: w1442 -> [w1500 _ _ _ _ _ _]
      frame "Initialize", Default {
        w1502 = State."ERROR"  # 下一个状态
        w1508 = FALSE  # 停止循环？
        w1505 = State."ResetCAN"  # 下一个状态
        # "初始化－对应用程序进行初始化。"
        n1131 = Select(t=w1505, s=TRUE, f=State."Exit" ("下一个状态")) -> (s? t:f=w1503:T3)
        n1132 = flat-sequence {
          tunnel: w1500 -> [w1510]
          tunnel: [w1510] -> w1499
          tunnel: w1499 -> [w1519]
          tunnel: [w1522] -> w1501
          frame #0 {
            n1133 = for {
              N: 8 -> [_]
              i -> [w1512]
              n1134 = Add(x=81, y=w1512) -> (x+y=w1511:i32)
              n1135 = call "CAN Uninitialize.vi"("Channel"=w1511) -> ()  [unwired: 9 in, 2 out]
            }
          }
          frame #1 {
            w1515 = T9 0 items=["刷新间隔", "波特率", "布尔1设置项", "布尔2设置项", "布尔3设置项", "布尔4设置项", "布尔5设置项", "显控1设置", "显控2设置", "显控3设置", "显控4设置", "显控5设置", "显控6设置", "显控7设置", "显控8设置", "显控9设置", "显控10设置", "显控11设置", "显控12设置", "设控1设置", "设控2设置", "设控3设置", "设控4设置", "设控5设置", "设控6设置", "设控7设置", "设控8设置", "曲线1设置", "曲线2设置", "曲线3设置", "曲线4设置", "曲线5设置", "曲线6设置", "曲线7设置", "曲线8设置", "曲线9设置", "曲线10设置", "曲线11设置", "曲线12设置", "曲线13设置", "曲线14设置", "曲线15设置", "曲线16设置", "ID值"] ("DataInitDef")
            w1516 = T12 0 items=["CONFIG"] ("Config Section")
            w1521 = T9 1 items=["刷新间隔", "波特率", "布尔1设置项", "布尔2设置项", "布尔3设置项", "布尔4设置项", "布尔5设置项", "显控1设置", "显控2设置", "显控3设置", "显控4设置", "显控5设置", "显控6设置", "显控7设置", "显控8设置", "显控9设置", "显控10设置", "显控11设置", "显控12设置", "设控1设置", "设控2设置", "设控3设置", "设控4设置", "设控5设置", "设控6设置", "设控7设置", "设控8设置", "曲线1设置", "曲线2设置", "曲线3设置", "曲线4设置", "曲线5设置", "曲线6设置", "曲线7设置", "曲线8设置", "曲线9设置", "曲线10设置", "曲线11设置", "曲线12设置", "曲线13设置", "曲线14设置", "曲线15设置", "曲线16设置", "ID值"] ("DataInitDef")
            # "1、从配置文件中读取上一次的记录。"
            n1136 = call "Read ini.vi"("configuration file path"=w1519) -> ("数组"=w1514:string[][])  [unwired: 10 in]
            "配置文件" <- w1514
            n1137 = Index Array(array=w1514, index (row)=w1516, index (col)=w1515) -> (element=w1520:string)
            n1138 = Index Array(array=w1514, index (row)=w1516, index (col)=w1521) -> (element=w1518:string)
            n1139 = property on="刷新间隔" class="Str"("Value"=w1520) -> ()  [unwired: 2 in, 2 out]
            n1140 = Hexadecimal String To Number(string=w1518) -> (number=w1517:u32)  [unwired: 2 in, 1 out]
            n1141 = property on="波特率" class="Ring (严格)"("Value"=w1517) -> ()  [unwired: 2 in, 2 out]
          }
          frame #2 {
            # "2、初始化CAN"
            n1142 = while {
              tunnel: [w1532] -> w1522
              i -> [w1525]
              stop <- w1526 stop-if-true
              w1524 = u8 81 ("Channel")
              n1143 = Add(x=w1524, y=w1525) -> (x+y=w1523:i32)
              "CAN通道" <- w1523
              n1144 = call "CAN Initialize.vi"("Btr0Btr1"="波特率", "Channel"=w1523) -> ("error out"=w1532:errorcluster, "function return"=w1527:u32)  [unwired: 8 in]
              n1145 = Equal To 0?(x=w1527) -> (x = 0?=w1528:bool)
              n1146 = Greater?(x=w1524, y=7) -> (0:w1529:bool)
              n1147 = Or(x=w1529, y=w1528) -> (x .or. y?=w1526:bool)
            }
          }
        }
        n1148 = Select(t=w1502, s=w1506, f=w1503) -> (s? t:f=w1507:T3)
        n1149 = call <vilib>:"Application Directory.vi"() -> ("Application Directory"=w1498:path)
        n1150 = Path To String(path=w1498) -> (string=w1497:string)
        n1151 = Reverse String(1:w1497) -> (0:w1496:string)
        n1152 = Match Pattern(string=w1496, regular expression="\\" ("正则表达式")) -> (before substring=w1494:string)  [unwired: 1 in, 3 out]
        n1153 = Reverse String(1:w1494) -> (0:w1493:string)
        n1154 = property on="项目名" class="Str"("Caption.Text"=w1493) -> ()  [unwired: 2 in, 2 out]
      }
      frame "ResetCAN" {
        # "复位CAN模块，并读取CAN模块的状态"
        n1155 = local read "CAN通道"() -> (w1534:u8)
        n1156 = call "CAN Reset.vi"("error in (no error)"=w1551, "Channel"=w1534) -> ("error out"=w1550:errorcluster, "function return"=w1545:u32)  [unwired: 8 in]
        n1157 = call "CAN Get Status.vi"("error in (no error)"=w1550, "Channel"=w1534) -> ("error out"=w1549:errorcluster, "function return"=w1548:u32)  [unwired: 8 in]
        n1158 = Equal To 0?(x=w1545) -> (x = 0?=w1544:bool)
        n1159 = Equal To 0?(x=w1548) -> (x = 0?=w1543:bool)
        n1160 = And(x=w1544, y=w1543) -> (x .and. y?=w1535:bool)
        n1161 = Select(t=State."SetCAN" ("下一个状态"), s=w1535, f=State."ERROR" ("返回初始状态")) -> (s? t:f=w1541:T3)
        n1162 = Select(t=w1541, s=TRUE, f=State."Exit" ("返回初始状态")) -> (s? t:f=w1539:T3)
        n1163 = Select(t=State."ERROR" ("下一个状态"), s=w1537, f=w1539) -> (s? t:f=w1538:T3)
      }
      frame "SetCAN" {
        w1566 = State."ERROR"  # 下一个状态
        w1568 = State."Exit"  # 返回初始状态
        w1567 = State."Process"  # 初始状态
        # "设置CAN模块的参数"
        n1164 = local read "CAN通道"() -> (w1554:u8)
        n1165 = Select(t=w1567, s=TRUE, f=w1568) -> (s? t:f=w1565:T3)
        n1166 = call "CAN Get Value.vi"("BufferLength"=u32 4, "error in (no error)"=w1570, "Parameter"=u8 1, "Channel"=w1554) -> ("error out"=w1555:errorcluster)  [unwired: 4 in, 3 out]
        n1167 = Select(t=w1566, s=w1563, f=w1565) -> (s? t:f=w1564:T3)
        n1168 = call "CAN Set Value.vi"("BufferLength"=u32 1280, "error in (no error)"=w1555, "Parameter"=u8 3, "Channel"=w1554) -> ("error out"=w1556:errorcluster)  [unwired: 5 in, 2 out]
        n1169 = local read "ID"() -> (w1559:u32)
        n1170 = call "CAN Filter Messages.vi"("Mode"=u8 2, "error in (no error)"=w1556, "ToID"=w1559, "FromID"=w1559, "Channel"=w1554) -> ("error out"=w1561:errorcluster)  [unwired: 5 in, 1 out]
      }
      frame "Process" {
        w1573 = State."ERROR"  # 下一个状态
        w1576 = State."Exit"  # 返回初始状态
        w1577 = State."Process"  # 初始状态
        n1171 = stacked-sequence {
          tunnel: w1572 -> [_ _ w1665]
          frame #0 {
            n1172 = while {
              stop <- w1584 continue-if-true
              (unwired) TRUE ("y")
              n1173 = local read "CAN通道"() -> (w1582:u8)
              n1174 = local read "ID"() -> (w1583:u32)
              n1175 = call "CAN Read.vi"("Channel"=w1582) -> ("data"=w1586:u8[], "function return"=w1585:u32, "ID"=w1581:u32)  [unwired: 6 in, 2 out]
              n1176 = Equal To 0?(x=w1585) -> (x = 0?=w1584:bool)
              n1177 = Equal?(x=w1581, y=w1583) -> (x = y?=w1580:bool)
              n1178 = And(x=w1584, y=w1580) -> (x .and. y?=w1587:bool)
              n1179 = case shown="真" w1587 {
                tunnel: w1586 -> [_ w1615]
                tunnel: w1581 -> [_ w1604]
                frame False {
                  n1180 = local read "刷新间隔"() -> (w1594:string)
                  n1181 = Decimal String To Number(string=w1594) -> (number=w1593:i32)  [unwired: 2 in, 1 out]
                  n1182 = local read "错误计数器"() -> (w1595:u32)
                  n1183 = Multiply(x=w1593, y=2) -> (x*y=w1590:i32)
                  n1184 = Increment(x=w1595) -> (x+1=w1598:u32)
                  n1185 = Add(x=10, y=w1590) -> (x+y=w1589:i32)
                  n1186 = Greater?(x=w1598, y=w1589) -> (0:w1599:bool)
                  n1187 = Decrement(x=w1589) -> (x-1=w1591:i32)
                  n1188 = Greater?(x=w1595, y=w1591) -> (0:w1596:bool)
                  n1189 = Select(t=w1589, s=w1599, f=w1598) -> (s? t:f=→"错误计数器":u32)
                  n1190 = case shown="假" w1596 {
                    frame False {
                      n1191 = property on="通信状态" class="Str"("Value"="正常" ("通信状态")) -> ()  [unwired: 2 in, 2 out]
                      n1192 = property on="通信状态" class="Str"("Text.TextColor"=u32 65280 ("文本.文本颜色:文本颜色")) -> ()  [unwired: 2 in, 2 out]
                    }
                    frame True {
                      n1193 = property on="通信状态" class="Str"("Value"="错误" ("通信状态")) -> ()  [unwired: 2 in, 2 out]
                      n1194 = property on="通信状态" class="Str"("Text.TextColor"=u32 16711680 ("文本.文本颜色:文本颜色")) -> ()  [unwired: 2 in, 2 out]
                    }
                  }
                }
                frame True {
                  # "CRC验证码校验"
                  n1195 = Split 1D Array(array=w1615, index=6 ("索引")) -> (first subarray=w1605:u8[], second subarray=w1611:u8[])
                  n1196 = call "CRC_A965 .vi"("U8"=w1605) -> ("CRC-16"=w1608:u16)  [unwired: 10 in]
                  n1197 = Index Array(array=w1611, index=1 ("索引")) -> (element=w1612:u8)
                  n1198 = Index Array(array=w1611, index=0 ("索引")) -> (element=w1609:u8)
                  n1199 = Join Numbers(hi=w1612, lo=w1609) -> ((hi.lo)=w1607:u16)
                  n1200 = Equal?(x=w1608, y=w1607) -> (x = y?=w1606:bool)
                  n1201 = case shown="真" w1606 {
                    tunnel: w1605 -> [_ w1622]
                    tunnel: w1604 -> [_ w1616]
                    frame False {
                    }
                    frame True {
                      # "当收到的功能码为1时，写入表格"
                      n1202 = Index Array(array=w1622, index=0 ("索引")) -> (element=w1650:u8)
                      n1203 = Index Array(array=w1622, index=1 ("索引")) -> (element=w1639:u8)
                      n1204 = Index Array(array=w1622, index=2 ("索引")) -> (element=w1647:u8)
                      n1205 = Index Array(array=w1622, index=3 ("索引")) -> (element=w1637:u8)
                      n1206 = Index Array(array=w1622, index=4 ("索引")) -> (element=w1628:u8)
                      n1207 = Index Array(array=w1622, index=5 ("索引")) -> (element=w1625:u8)
                      n1208 = To Unsigned Word Integer(number=w1625) -> (unsigned 16bit integer=w1624:u16)
                      n1209 = To Unsigned Word Integer(number=w1637) -> (unsigned 16bit integer=w1636:u16)
                      n1210 = And(x=w1639, y=u8 15) -> (x .and. y?=w1635:u8)
                      n1211 = Logical Shift(y=i16 -4, x=w1639) -> (x << y=w1638:u8)
                      n1212 = Logical Shift(y=i16 8, x=w1624) -> (x << y=w1626:u16)
                      n1213 = To Unsigned Word Integer(number=w1635) -> (unsigned 16bit integer=w1634:u16)
                      n1214 = And(x=w1638, y=u16 3) -> (x .and. y?=w1632:u16)
                      n1215 = Logical Shift(y=i16 8, x=w1636) -> (x << y=w1643:u16)
                      n1216 = Add(x=w1628, y=w1626) -> (x+y=w1623:u16)
                      n1217 = Add(x=w1647, y=w1643) -> (x+y=w1619:u16)
                      n1218 = Logical Shift(y=i16 8, x=w1634) -> (x << y=w1641:u16)
                      n1219 = To Unsigned Long Integer(number=w1623) -> (unsigned 32bit integer=w1621:u32)
                      n1220 = Add(x=w1650, y=w1641) -> (x+y=w1646:u16)
                      n1221 = Logical Shift(y=i16 16, x=w1621) -> (x << y=w1617:u32)
                      n1222 = Equal?(x=w1632, y=u16 1) -> (x = y?=w1633:bool)
                      n1223 = Add(x=w1619, y=w1617) -> (x+y=w1618:u32)
                      n1224 = case shown="真" w1633 {
                        tunnel: w1646 -> [_ w1659]
                        tunnel: w1618 -> [_ w1658]
                        tunnel: w1616 -> [_ w1657]
                        frame False {
                        }
                        frame True {
                          n1225 = Build Array(w1659, w1658, w1657) -> (w1656:u32[])
                          n1226 = local read "CANBURF"() -> (w1655:u32[][])
                          n1227 = local write "错误计数器"(u32 0 ("数值 2")) -> ()
                          n1228 = call "收到的数据排序V2.vi"("BUF"=w1655, "输入数据"=w1656) -> ("BUF OUT"=w1654:u32[][])  [unwired: 7 in]
                          n1229 = local write "CANBURF"(w1654) -> ()
                        }
                      }
                    }
                  }
                }
              }
            }
          }
          frame #1 {
            n1230 = event shown="[1] \"要发送的数据\": 值改变" {
              selector: _ -> [_ _]
              dyn-events: _ -> [_ _]
              timeout: 0 -> [_ _]
              event Timeout {
                n1231 = event-data() -> ()  [unwired: 1 in, 3 out]
              }
              event "要发送的数据": Value Change {
                # "写入命令VI"
                n1232 = event-data() -> ()  [unwired: 1 in, 6 out]
                n1233 = local read "ID"() -> (w1662:u32)
                n1234 = property on="要发送的数据" class="Clust (严格)"() -> ("Value"=w1664:cluster{"地址":u16, "数据":i32, "行数":i32, "ID":i32})  [unwired: 2 in, 2 out]
                n1235 = local read "CAN通道"() -> (w1663:u8)
                n1236 = call "数据写入.vi"("CAN通道"=w1663, "ID"=w1662, "簇"=w1664) -> ()  [unwired: 9 in]
              }
            }
          }
          frame #2 {
            n1237 = Decimal String To Number(string="刷新间隔") -> (number=w1671:i32)  [unwired: 2 in, 1 out]
            n1238 = Equal To 0?(x=w1671) -> (x = 0?=w1668:bool)
            n1239 = Select(t=1, s=w1668, f=w1671) -> (s? t:f=w1669:i32)
            n1240 = Quotient & Remainder(x=w1665, y=w1669) -> (x-y*floor(x/y)=w1667:i32)  [unwired: 1 out]
            n1241 = Equal To 0?(x=w1667) -> (x = 0?=w1666:bool)
            n1242 = case shown="真" w1666 {
              frame False {
              }
              frame True {
                # "本框架为CAN通信主要框架，实现每隔指定的时间对参数列表中的参数进行循环发送和读取"
                n1243 = local read "表格"() -> (w1675:string[][])
                n1244 = property on="循环指针" class="DigNum (严格)"() -> ("Value"=w1674:u16)  [unwired: 2 in, 2 out]
                n1245 = disable-structure shown="禁用" {
                  disable-tunnel: w1675 -> [w1688 _]
                  disable-tunnel: w1674 -> [w1687 _]
                  frame Disabled {
                    n1246 = Index Array(array=w1688, index (row)=w1687, index (col)=7 ("禁用的索引 (列)")) -> (element=w1682:string)
                    n1247 = Hexadecimal String To Number(string=w1682) -> (number=w1681:u32)  [unwired: 2 in, 1 out]
                    n1248 = Equal?(x=w1682, y="") -> (x = y?=w1684:bool)
                    n1249 = Select(s=w1684, f=w1681) -> (s? t:f=→"运行ID":u32)  [unwired: 1 in]
                  }
                  frame Enabled {
                  }
                }
                n1250 = Index Array(array=w1675, index (row)=w1674, index (col)=0 ("禁用的索引 (列)")) -> (element=w1678:string)
                n1251 = Increment(x=w1674) -> (x+1=→"循环指针":u16)
                n1252 = local read "ID"() -> (w1673:u32)
                n1253 = Equal?(x=w1678, y="") -> (x = y?=w1676:bool)
                n1254 = case shown="真" w1676 {
                  tunnel: w1675 -> [w1692 _]
                  tunnel: w1674 -> [w1691 _]
                  tunnel: w1673 -> [w1690 _]
                  frame False {
                    # "如果下一行的第0列没有任何数据，则认为本表已经循环完毕。将指针回零重新下一轮的循环123456"
                    n1255 = local read "CAN通道"() -> (w1689:u8)
                    n1256 = call "循环读取命令.vi"("循环指针"=w1691, "表格"=w1692, "ID"=w1690, "CAN通道"=w1689) -> ()  [unwired: 8 in]
                  }
                  frame True {
                    # "如果下一行的第0列没有任何数据，则认为本表已经循环完毕。将指针回零重新下一轮的循环"
                    n1257 = stacked-sequence {
                      frame #0 {
                        n1258 = Tick Count (ms)() -> (millisecond timer value=w1694:u32)
                        n1259 = feedback-in #1(w1694) -> ()
                        n1260 = feedback #1() -> (w1695:u32)  [unwired: 1 in]
                        n1261 = Subtract(x=w1694, y=w1695) -> (x-y=w1696:u32)
                        n1262 = Divide(x=w1696, y=1000) -> (x/y=w1698:dbl)
                        n1263 = Number To Fractional String(number=w1698, precision (6)=i16 3 ("精度(6)")) -> (F-format string=w1697:string)  [unwired: 2 in]
                        n1264 = property on="轮询一次周期" class="Str"("Value"=w1697) -> ()  [unwired: 2 in, 2 out]
                      }
                      frame #1 {
                        n1265 = flat-sequence {
                          frame #0 {
                            # "波形记录"
                            n1266 = local read "控件配置文件"() -> (w1713:string[][])
                            n1267 = local read "表格"() -> (w1714:string[][])
                            n1268 = call "波形记录处理.vi"("控件配置文件"=w1713, "表格"=w1714) -> ("曲线数量"=w1705:u16, "曲线名称"=w1703:string[], "波形图"=w1707:dynamicdata)  [unwired: 5 in]
                            n1269 = case shown="真" "清除历史记录" {
                              frame False {
                              }
                              frame True {
                                n1270 = property on="波形图表" class="WFChart (严格)"("History Data"=dynamicdata[] [] ("历史数据")) -> ()  [unwired: 2 in, 2 out]
                              }
                            }
                            n1271 = feedback #2() -> (w1711:u16)  [unwired: 1 in]
                            n1272 = feedback-in #2(w1705) -> ()
                            n1273 = feedback #3() -> (w1704:string[])  [unwired: 1 in]
                            n1274 = feedback-in #3(w1703) -> ()
                            n1275 = case shown="真" "记录波形更新" {
                              tunnel: w1707 -> [_ w1718]
                              frame False {
                              }
                              frame True {
                                "波形图表" <- w1718
                              }
                            }
                            n1276 = Equal To 0?(x=w1705) -> (x = 0?=w1708:bool)
                            n1277 = Not Equal?(x=w1705, y=w1711) -> (x != y?=w1702:bool)
                            n1278 = Not Equal?(x=w1703, y=w1704) -> (x != y?=w1701:bool)
                            n1279 = Or(x=w1702, y=w1701) -> (x .or. y?=w1700:bool)
                            n1280 = feedback #4() -> (w1710:bool)  [unwired: 1 in]
                            n1281 = feedback-in #4(w1700) -> ()
                            n1282 = case shown="真" w1700 {
                              tunnel: w1703 -> [_ w1719]
                              tunnel: w1705 -> [_ w1720]
                              frame False {
                              }
                              frame True {
                                n1283 = stacked-sequence {
                                tunnel: w1720 -> [w1722 _]
                                tunnel: w1719 -> [_ w1724]
                                frame #0 {
                                n1284 = Greater Than 0?(x=w1722) -> (x > 0?=w1723:bool)
                                n1285 = property on="波形图表" class="WFChart (严格)"("LegNumRows"=w1722, "Legend Visible"=w1723, "Dig Display(s) Visible"=FALSE ("数字显示可见"), "LegPlotMin"=w1722) -> ()  [unwired: 2 in, 2 out]
                                }
                                frame #1 {
                                n1286 = for "For循环" {
                                tunnel: w1724 -> [w1725] mode=indexing
                                i -> [w1726]
                                n1287 = call "字符串比对X.vi"("字符串"=w1725) -> ("布尔"=w1727:bool)  [unwired: 10 in]
                                n1288 = property on="波形图表" class="WFChart (严格)"("Active Plot"=w1726, "Plot.Plot Name"=w1725, "Plot.Visible?"=w1727) -> ()  [unwired: 2 in, 2 out]
                                }
                                }
                                }
                              }
                            }
                            n1289 = Not Equal?(x=w1710, y=w1700) -> (x != y?=w1709:bool)
                            n1290 = case shown="真" w1709 {
                              frame False {
                              }
                              frame True {
                                n1291 = property on="波形图表" class="WFChart (严格)"("Dig Display(s) Visible"=TRUE) -> ()  [unwired: 2 in, 2 out]
                              }
                            }
                            n1292 = case shown="真" w1708 {
                              frame False {
                              }
                              frame True {
                                n1293 = property on="波形图表" class="WFChart (严格)"("Dig Display(s) Visible"=FALSE ("数字显示可见")) -> ()  [unwired: 2 in, 2 out]
                              }
                            }
                          }
                        }
                      }
                      frame #2 {
                        n1294 = property on="循环指针" class="DigNum (严格)"("Value"=u16 0 ("循环指针")) -> ()  [unwired: 2 in, 2 out]
                      }
                    }
                  }
                }
              }
            }
          }
        }
        n1295 = Select(t=w1577, s=TRUE, f=w1576) -> (s? t:f=w1575:T3)
        n1296 = Select(t=w1573, s=w1578, f=w1575) -> (s? t:f=w1579:T3)
      }
      frame "Exit" {
        w1733 = State."STOP"  # （下一个状态）
        # "退出－退出应用程序。"
        n1297 = local read "CAN通道"() -> (w1729:u8)
        n1298 = call "CAN Uninitialize.vi"("error in (no error)"=w1730, "Channel"=w1729) -> ("error out"=w1732:errorcluster)  [unwired: 8 in, 1 out]
      }
      frame "ERROR" {
        w1737 = State."Initialize"  # 初始状态
        n1299 = local read "CAN通道"() -> (w1735:u8)
        n1300 = call "CAN Uninitialize.vi"("error in (no error)"=w1739, "Channel"=w1735) -> ("error out"=w1740:errorcluster)  [unwired: 8 in, 1 out]
        n1301 = call <vilib>:"Simple Error Handler.vi"("error code (no error:0)"=0, "error in (no error)"=w1740) -> ("error out"=w1738:errorcluster)  [unwired: 3 in, 4 out]
        n1302 = Wait (ms)(milliseconds to wait=u32 10 ("等待时间（毫秒）")) -> ()  [unwired: 1 out]
      }
      frame "STOP" {
        w1743 = State."STOP"  # （未用值）
      }
    }
    n1303 = event shown="[1] \"波特率\", \"刷新间隔\", \"布控1设置\", \"显控1设置\", \"显控2设置\", \"显控3设置\", \"显控4设置\", \"显控5设置\", \"显控6设置\", \"显控7设置\", \"显控8设置\", \"显控9设置\", \"显控10设置\", \"显控11设置\", \"显控12设置\", \"布控2设置\", \"布控3设置\", \"布控4设置\", \"设控设置 1\", \"设控设置 2\", \"设控设置 3\", \"设控设置 4\", \"设控设置 5\", \"设控设置 6\", \"设控设置 7\", \"设控设置 8\", \"曲线1设置\", \"曲线2设置\", \"曲线3设置\", \"曲线4设置\", \"曲线5设置\", \"曲线6设置\", \"曲线7设置\", \"曲线8设置\", \"ID\", \"布控5设置\", \"曲线9设置\", \"曲线10设置\", \"曲线11设置\", \"曲线12设置\", \"曲线13设置\", \"曲线14设置\", \"曲线15设置\", \"曲线16设置\", \"数据模式\": 值改变" {
      selector: _ -> [_ _]
      dyn-events: _ -> [_ _]
      timeout: 0 -> [_ _]
      tunnel: w1442 -> [_ w1463]
      tunnel: w1434 -> [_ w1460]
      event Timeout {
        n1304 = event-data() -> ()  [unwired: 1 in, 3 out]
      }
      event "波特率", "刷新间隔", "布控1设置", "显控1设置", "显控2设置", "显控3设置", "显控4设置", "显控5设置", "显控6设置", "显控7设置", "显控8设置", "显控9设置", "显控10设置", "显控11设置", "显控12设置", "布控2设置", "布控3设置", "布控4设置", "设控设置 1", "设控设置 2", "设控设置 3", "设控设置 4", "设控设置 5", "设控设置 6", "设控设置 7", "设控设置 8", "曲线1设置", "曲线2设置", "曲线3设置", "曲线4设置", "曲线5设置", "曲线6设置", "曲线7设置", "曲线8设置", "ID", "布控5设置", "曲线9设置", "曲线10设置", "曲线11设置", "曲线12设置", "曲线13设置", "曲线14设置", "曲线15设置", "曲线16设置", "数据模式": Value Change {
        # "参数保存。当有更多的参数需要保存时，在此框图中增加事件触发和相应的元素"
        n1305 = event-data() -> ()  [unwired: 1 in, 3 out]
        n1306 = property on="刷新间隔" class="Str"() -> ("Label.Text"=w1469:string)  [unwired: 2 in, 2 out]
        n1307 = property on="波特率" class="Ring (严格)"() -> ("Value"=w1470:u16)  [unwired: 2 in, 2 out]
        n1308 = property on="波特率" class="Ring (严格)"() -> ("Label.Text"=w1467:string)  [unwired: 2 in, 2 out]
        n1309 = property on="刷新间隔" class="Str"() -> ("Value"=w1468:string)  [unwired: 2 in, 2 out]
        n1310 = Number To Hexadecimal String(2:w1470) -> (0:w1466:string)  [unwired: 1 in]
        n1311 = Build Array(w1469, w1468) -> (w1462:string[])
        n1312 = Build Array(w1467, w1466) -> (w1461:string[])
        n1313 = Build Array(w1462, w1461) -> (w1464:string[][])
        n1314 = call "Write ini.vi"("configuration file path"=w1463, "数组"=w1464, "段"="CONFIG" ("元素")) -> ()  [unwired: 9 in]
        n1315 = stacked-sequence {
          tunnel: w1460 -> [_ _ w1489]
          frame #0 {
            w1475 = T9 43 items=["刷新间隔", "波特率", "布尔1设置项", "布尔2设置项", "布尔3设置项", "布尔4设置项", "布尔5设置项", "显控1设置", "显控2设置", "显控3设置", "显控4设置", "显控5设置", "显控6设置", "显控7设置", "显控8设置", "显控9设置", "显控10设置", "显控11设置", "显控12设置", "设控1设置", "设控2设置", "设控3设置", "设控4设置", "设控5设置", "设控6设置", "设控7设置", "设控8设置", "曲线1设置", "曲线2设置", "曲线3设置", "曲线4设置", "曲线5设置", "曲线6设置", "曲线7设置", "曲线8设置", "曲线9设置", "曲线10设置", "曲线11设置", "曲线12设置", "曲线13设置", "曲线14设置", "曲线15设置", "曲线16设置", "ID值"] ("DataInitDef")
            n1316 = local read "ID"() -> (w1472:u32)
            n1317 = Number To Hexadecimal String(2:w1472) -> (0:w1471:string)  [unwired: 1 in]
            n1318 = invoke on="控件配置文件" class="Tbl (严格)" method="Set Cell Value"("X Index"=1 ("X索引"), "Y Index"=w1475, "Value"=w1471) -> ()  [unwired: 3 in, 6 out]
            n1319 = invoke on="控件配置文件" class="Tbl (严格)" method="Set Cell Value"("X Index"=0 ("X索引"), "Y Index"=w1475, "Value"="ID" ("值")) -> ()  [unwired: 3 in, 6 out]
          }
          frame #1 {
            w1477 = T9 44 items=["刷新间隔", "波特率", "布尔1设置项", "布尔2设置项", "布尔3设置项", "布尔4设置项", "布尔5设置项", "显控1设置", "显控2设置", "显控3设置", "显控4设置", "显控5设置", "显控6设置", "显控7设置", "显控8设置", "显控9设置", "显控10设置", "显控11设置", "显控12设置", "设控1设置", "设控2设置", "设控3设置", "设控4设置", "设控5设置", "设控6设置", "设控7设置", "设控8设置", "曲线1设置", "曲线2设置", "曲线3设置", "曲线4设置", "曲线5设置", "曲线6设置", "曲线7设置", "曲线8设置", "曲线9设置", "曲线10设置", "曲线11设置", "曲线12设置", "曲线13设置", "曲线14设置", "曲线15设置", "曲线16设置", "ID值", "数据模式"] ("DataInitDef")
            n1320 = local read "数据模式"() -> (w1478:bool)
            n1321 = Boolean To (0,1)(Boolean=w1478) -> (0, 1=w1479:i16)
            n1322 = Number To Hexadecimal String(2:w1479) -> (0:w1480:string)  [unwired: 1 in]
            n1323 = invoke on="控件配置文件" class="Tbl (严格)" method="Set Cell Value"("X Index"=1 ("X索引"), "Y Index"=w1477, "Value"=w1480) -> ()  [unwired: 3 in, 6 out]
            n1324 = invoke on="控件配置文件" class="Tbl (严格)" method="Set Cell Value"("X Index"=0 ("X索引"), "Y Index"=w1477, "Value"="数据模式" ("值")) -> ()  [unwired: 3 in, 6 out]
          }
          frame #2 {
            n1325 = property on="控件配置文件" class="Tbl (严格)"() -> ("Value"=w1487:string[][])  [unwired: 2 in, 2 out]
            n1326 = Array To Spreadsheet String(array=w1487, 3:"%s" ("格式字符串")) -> (spreadsheet string=w1486:string)  [unwired: 1 in]
            n1327 = Write to Text File(file (use dialog)=w1489, text=w1486) -> (refnum out=w1485:refnum<file>, error out=w1484:errorcluster)  [unwired: 2 in, 1 out]
            n1328 = Close File(refnum=w1485, error in=w1484) -> ()  [unwired: 2 out]
          }
        }
      }
    }
    n1329 = local write "i1"(w1430) -> ()
    n1330 = Quotient & Remainder(x=w1430, y=20) -> (x-y*floor(x/y)=w1437:i32)  [unwired: 1 out]
    n1331 = event shown="[1] \"退出\": 值改变" {
      selector: _ -> [_ _]
      dyn-events: _ -> [_ _]
      timeout: 0 -> [_ _]
      event Timeout {
        n1332 = event-data() -> ()  [unwired: 1 in, 3 out]
      }
      event "退出": Value Change {
        n1333 = event-data() -> ()  [unwired: 1 in, 6 out]
        n1334 = Two Button Dialog(message="确定退出" ("消息")) -> (T button?=w1450:bool)  [unwired: 2 in]
        n1335 = case shown="真" w1450 {
          frame False {
          }
          frame True {
            n1336 = local read "CAN通道"() -> (w1451:u8)
            n1337 = Quit LabVIEW(quit? (T)=TRUE ("退出？(T)")) -> ()
            n1338 = call "CAN Uninitialize.vi"("Channel"=w1451) -> ()  [unwired: 9 in, 2 out]
          }
        }
      }
    }
    n1339 = Equal To 0?(x=w1437) -> (x = 0?=w1436:bool)
    n1340 = case shown="真" w1436 {
      tunnel: w1435 -> [w1454 w1458]
      tunnel: w1441 -> [w1453 w1457]
      tunnel: [w1454 w1456] -> w1440
      tunnel: [w1453 w1455] -> w1439
      frame False {
      }
      frame True {
        # "每20ms发送一个通知启动界面程序"
        n1341 = call "Error_mx.vi"() -> ()  [unwired: 12 in]
        n1342 = Send Notification(notification="RUN" ("通知"), notifier=w1458, error in (no error)=w1457) -> (notifier out=w1456:refnum<notifier>, error out=w1455:errorcluster)
      }
    }
    n1343 = node-c288() -> ()  [unwired: 1 in, 1 out]
  }
  n1344 = node-c288(w19) -> ()  [unwired: 1 out]
  n1345 = local read "CAN通道"() -> (w1:u8)
  n1346 = local read "CAN通道"() -> (w2:u8)
  n1347 = Release Notifier(notifier=w13, error in (no error)=w12) -> (error out=w4:errorcluster)  [unwired: 1 in, 2 out]
  n1348 = call "CAN Uninitialize.vi"("error in (no error)"=w3, "Channel"=w1) -> ("error out"=w21:errorcluster)  [unwired: 8 in, 1 out]
  n1349 = call "CAN Uninitialize.vi"("error in (no error)"=w4, "Channel"=w2) -> ("error out"=w5:errorcluster)  [unwired: 8 in, 1 out]
  n1350 = call <vilib>:"Simple Error Handler.vi"("error code (no error:0)"=0, "error in (no error)"=w5) -> ()  [unwired: 3 in, 5 out]
  n1351 = call <vilib>:"Simple Error Handler.vi"("error code (no error:0)"=0, "error in (no error)"=w21) -> ()  [unwired: 3 in, 5 out]
